vi "runStudy_USRP_2ChNCS_7.vi"() -> (2 "Ch2Amp":dbl[](graph), 3 "Ch1Amp":dbl[](graph), 4 "# elements in queue 2":i32)   [LabVIEW 2016]
uses:
  <instrlib>/niUSRP/niUSRP Timestamp.ctl
  <vilib>/Utility/miscctls.llb/LVDateTimeRec.ctl
  <vilib>/sound2/lvsound2.llb/Sound File Position.ctl
  <vilib>/sound2/lvsound2.llb/Sampling Mode.ctl
  <vilib>/sound2/lvsound2.llb/Sound Data Format.ctl
  <vilib>/Analysis/3filter.llb/Filter Passband Type.ctl
  <instrlib>/niUSRP/niUSRP Configure Time Start Trigger.vi
  <vilib>/sound2/lvsound2.llb/Sound Input Read (DBL).vi
  <instrlib>/niUSRP/niUSRP Write Tx Data (2D CDB).vi
  <instrlib>/niUSRP/niUSRP Fetch Rx Data (2D CDB).vi
  <vilib>/Analysis/3filter.llb/Butterworth Filter (DBL).vi
  <vilib>/Analysis/3filter.llb/Butterworth Filter (CDB).vi
  <vilib>/sound2/lvsound2.llb/Sound File Info (path).vi
  <vilib>/sound2/lvsound2.llb/Sound File Read Open.vi
  <vilib>/sound2/lvsound2.llb/Sound File Read (DBL).vi
  <vilib>/sound2/lvsound2.llb/Sound Output Write (DBL).vi
  <vilib>/measure/NI_MABase.lvlib
  <vilib>/Analysis/NI_AALBase.lvlib
  <vilib>/Analysis/NI_AALPro.lvlib
panel:
  in  "Sound R3a":T1=2 items=["Absolute"=0, "Relative"=2]
  in  "Play sound":u16(ring) items=["No sound", "Demo deep breathing", "Demo fast shallow breathing", "Demo slow shallow breathing", "Demo breath hold", "Demo cough/ laugh", "Demo abdomen movement", "Calibration", "Routine 1", "Routine 3b", "Routine 4/5/7", "Calm music", "Routine 3a"]
  in  "Sound Dcough":T1=2 items=["Absolute"=0, "Relative"=2]
  in  "Sound Dhold":T1=2 items=["Absolute"=0, "Relative"=2]
  in  "Sound Dabd":T1=2 items=["Absolute"=0, "Relative"=2]
  in  "Sound Dss":T1=2 items=["Absolute"=0, "Relative"=2]
  in  "Play/Stop":bool
  in  "Sound Ddeep":T1=2 items=["Absolute"=0, "Relative"=2]
  in  "Sound Dfs":T1=2 items=["Absolute"=0, "Relative"=2]
  in  "Sound R3b":T1=2 items=["Absolute"=0, "Relative"=2]
  in  "Sound R457":T1=2 items=["Absolute"=0, "Relative"=2]
  out "Next Task":string
  out "Calib 7":bool caption="Time has Elapsed"
  out "Calib 5":bool caption="Time has Elapsed"
  out "Calib 4":bool caption="Time has Elapsed"
  out "Calib 3":bool caption="Time has Elapsed"
  in  "Sound Calib":T1=2 items=["Absolute"=0, "Relative"=2]
  out "Calib 1":bool caption="Time has Elapsed"
  in  "Abd Circumference (cm)":string="0"
  in  "Thorax Circumference (cm)":string="0"
  out "Current Task time":dbl(slide) scale=0.0..60.0
  in  "Flush Th":i32=50
  in  "Stop 3":bool
  out "# elements in Mic":i32=5200
  in  "FlushMic":bool
  out "Mic":waveform(dbl)[](graph)
  in  "Device ID":u32 format="%.0x"
  in  "Number of Samples/ch":i32=5000
  in  "Sound Music":T1=2 items=["Absolute"=0, "Relative"=2]
  out "#2b":bool caption="Time has Elapsed"
  in  "Sound R1":T1=2 items=["Absolute"=0, "Relative"=2]
  in  "number of samples/ch":i32=5000
  out "#7":bool caption="Time has Elapsed"
  out "#2a":bool caption="Time has Elapsed"
  out "#6":bool caption="Time has Elapsed"
  out "#5":bool caption="Time has Elapsed"
  out "#4":bool caption="Time has Elapsed"
  in  "Comments":string
  in  "Tab Control 6":enum32{"Amp @500Hz", "Ph @500Hz"}(tab)
  out "IQ Graph 5":dbl[][](graph)
  out "IQ Graph 6":dbl[][](graph)
  in  "Tab Control 3":enum32{"Ch1 Amp", "Ch1 Ph"}(tab)
  in  "fh 1":dbl=26.0 format="%0.2f"
  in  "fl 1":dbl=0.7 format="%0.4f"
  out "Ch1Ph":dbl[](graph)
  in  "fl 3":dbl=0.7 format="%0.4f"
  in  "fh 3":dbl=26.0 format="%0.2f"
  in  "Tab Control 2":enum32{"Amp @50kHz", "Ph @50kHz"}(tab)
  out "Amp both":dbl[][](graph)
  out "Phase Both":dbl[][](graph)
  in  "Tab Control":enum32{"Ch2 Amp", "Ch2 Ph"}(tab)
  in  "fh 2":dbl=26.0 format="%0.2f"
  in  "fl 2":dbl=15.0 format="%0.4f"
  out "Ch2Ph":dbl[](graph)
  in  "fl 4":dbl=15.0 format="%0.4f"
  in  "fh 4":dbl=26.0 format="%0.2f"
  out "ArraySz":i32[](array[numeric])
  in  "Stop Test":bool
  out "#1":bool caption="Time has Elapsed"
  out "#3b":bool caption="Time has Elapsed"
  out "#3a":bool caption="Time has Elapsed"
  out "Elapsed Time (s)":dbl
  in  "Protocol":u16(ring) items=["Not Running", "Test Run", "Routine 1", "Routine 2a", "Routine 2b", "Routine 3a", "Routine 3b", "Routine 4", "Routine 5", "Routine 6", "Routine 7", "Calib1", "calib3", "Calib4", "Calib5", "Calib8"]
  out "Read:Tx IQ Rate":dbl=5000000.0
  out "Read:Rx IQ Rate":dbl=5000000.0
  out "date time rec":T2
  out "Total Routine Time":dbl(slide) scale=0.0..415.0
  out "Current Task":string
  in  "Weight (lbs)":string="0"
  in  "Case Number":string="0"
  in  "Height (cm)":string="0"
  in  "Sex":string(combo)="Female"
  in  "Age (years)":string="0"
  out "Numeric 2":i32=1
  out "Save":bool
  out "Flush":bool
  out "Buffer":bool
  out "Output":i32=1
  out "Configuration:Bandwidth":dbl=5000000.0
  out "Ch2 Amplitude":dbl=0.5 step=0.05 format="%#.6g"
  out "Ch1 Amplitude":dbl=0.5 step=0.05 format="%#.6g"
  out "Dis Sampling Rate":dbl=500.0 format="%#_6p"
  in  "DownSamplingRatio 2":i32=100
  out "Sampling Rate":dbl=50000.0 format="%#_6p"
  out "2Ch Waveforms":dbl[][](array[numeric])
  out "IterationNum":i32=1009
  in  "DownSamplingRatio":i32=40
  out "# elements in queue":i32
  out "BW/2":dbl=1000.0
  out "# of queue 1":i32
  in  "Dis1":bool=TRUE
  out "IQ Graph":dbl[][](graph)
  out "Tx1 Waveform":cdb[][](array[numeric])
  in  "Rx carrier frequency [Hz]":dbl=1900000000.0 format="%#_6p"
  in  "Tx carrier frequency [Hz]":dbl=1900000000.0 format="%#_6p"
  in  "Rx1 Gain 2":dbl=32.0 format="%#_6f"
  in  "Tx1 Gain 2":dbl=22.0 format="%#_6f"
  out "error out":errorcluster
  in  "Start Trigger Time":T3={"whole seconds"=1, "fractional seconds"=0.0}
  in  "Stop":bool
  in  "Channel 2\nTone Amplitude":dbl=0.5 step=0.05 format="%#.6g"
  in  "Channel 2 \nTone Frequency":dbl=131000.0 format="%#_6p"
  in  "Channel 1\nTone Amplitude":dbl=0.5 step=0.05 format="%#.6g"
  in  "Channel 1 \nTone Frequency":dbl=51000.0 format="%#_6p"
  out "Tx1 Waveform Graph":waveform(dbl)[](graph)
  in  "Waveform Size 1":dbl=20000.0
  in  "Device Name":refnum<k15>="MyB210"
  in  "Tx1 Gain 1":dbl=22.0 format="%#_6f"
  in  "Tx IQ Rate 1":dbl=2000000.0 format="%#_6p"
  in  "Rx1 Gain 1":dbl=32.0 format="%#_6f"
  in  "Rx IQ Rate 1":dbl=2000000.0 format="%#_6p"
  # "User Instructions"
  # "Step 1: User Information"
  # "Step 2: Protocol Selection"
  # "Ch 1"
  # "Ch 2"
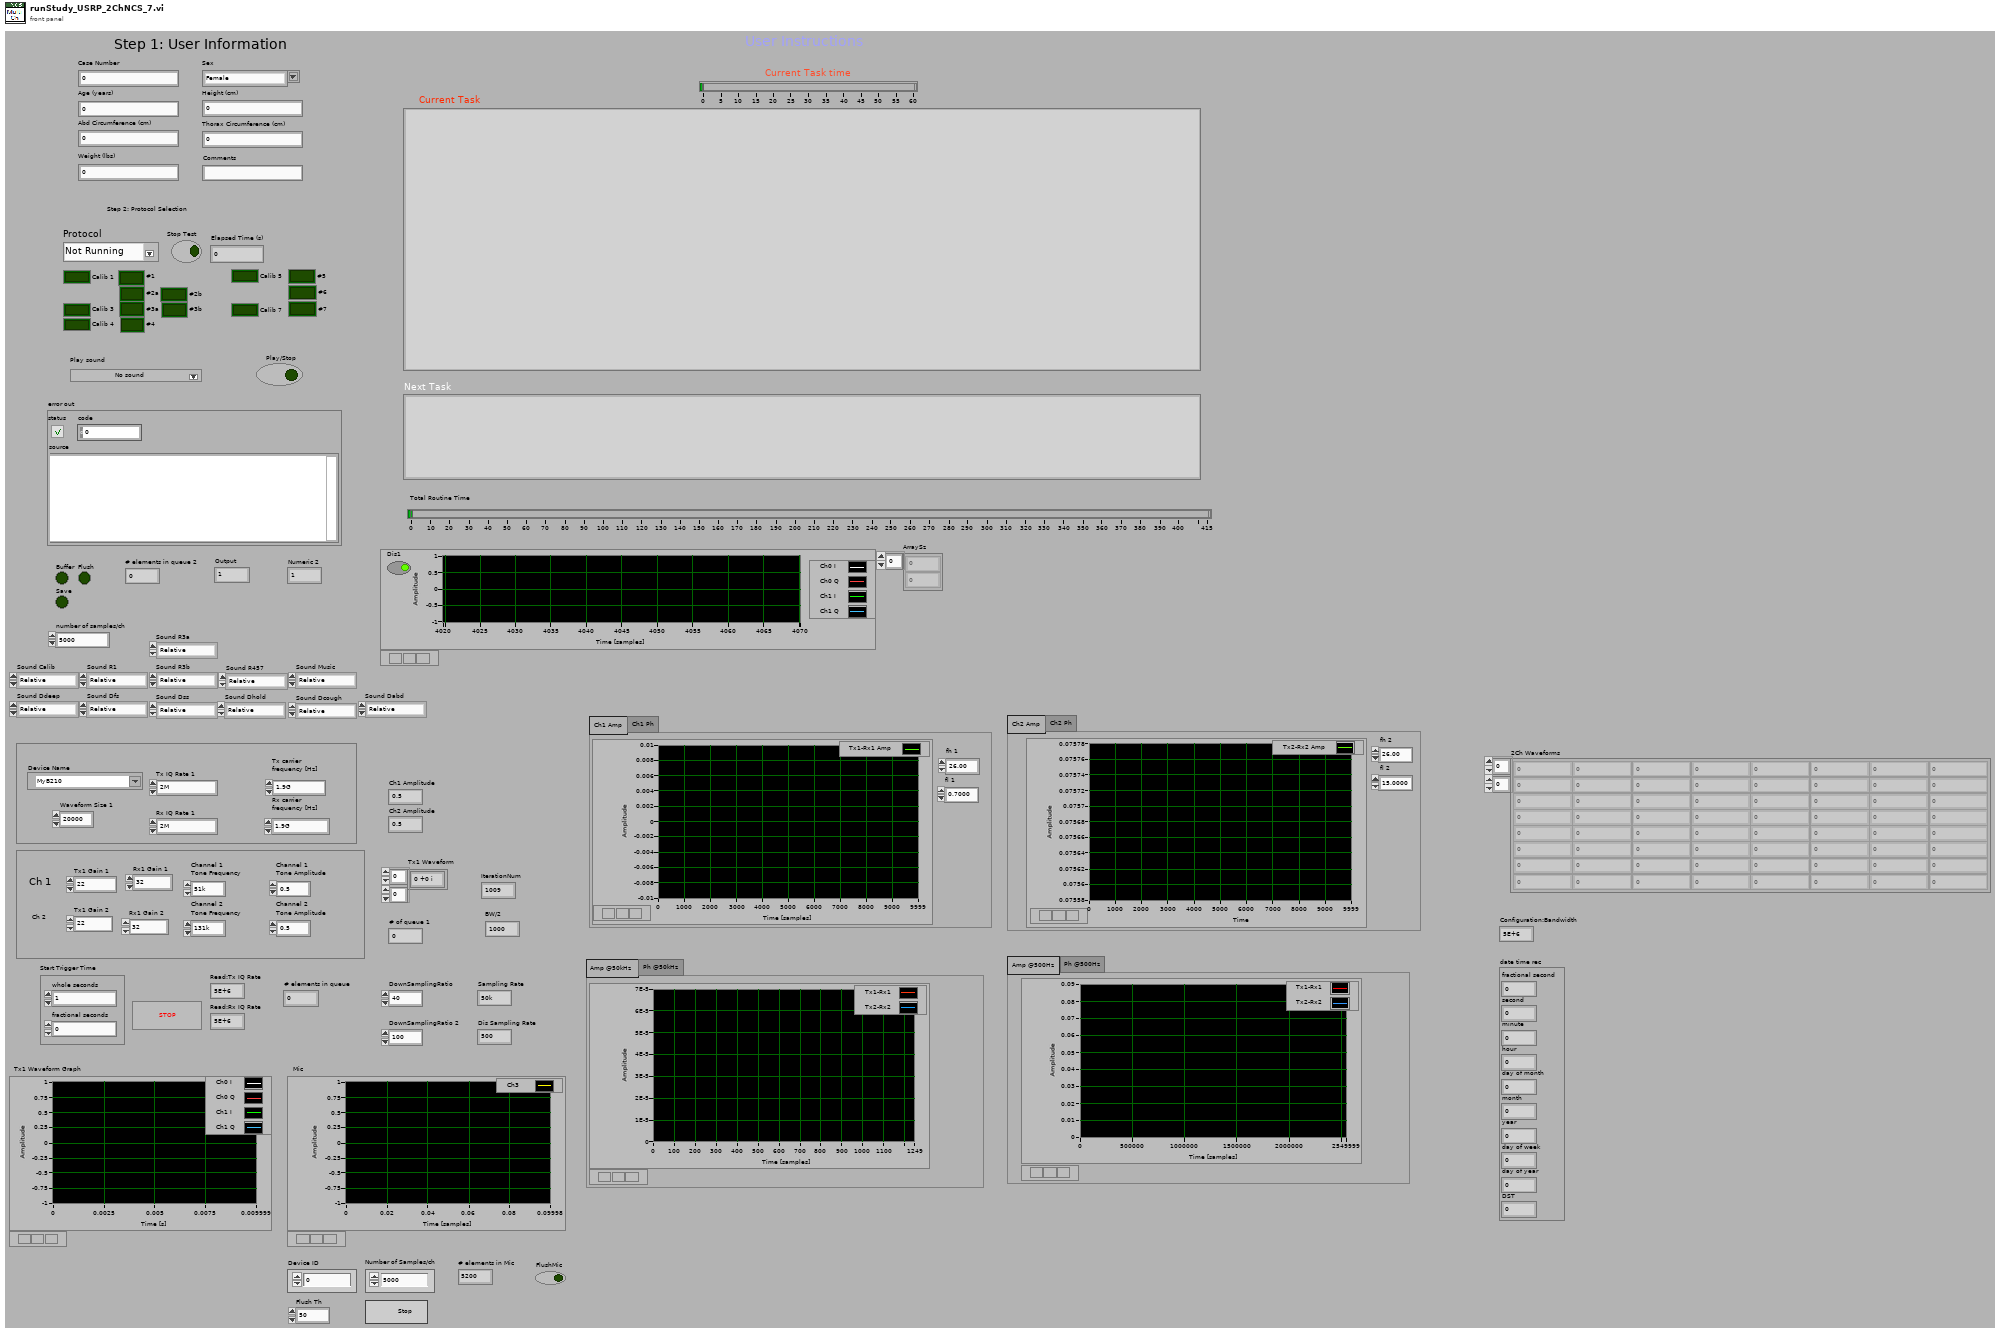
[diagram p1: front panel]
types:
  T1 = typedef "Sound File Position.ctl" = u16
  T2 = typedef "LVDateTimeRec.ctl" = cluster{"fractional second":dbl, "second":i32, "minute":i32, "hour":i32, "day of month":i32, "month":i32, "year":i32, "day of week":i32, "day of year":i32, "DST":i32}
  T3 = typedef "niUSRP Timestamp.ctl" = cluster{"whole seconds":u64, "fractional seconds":dbl}
  T4 = enum16{"Default", "Test", "Routine 1", "Routine 2a", "Routine 2b", "Routine 3a", "Routine 3b", "Routine 4", "Routine 5", "Routine 6", "Routine 7", "Calib1", "Calib3", "Calib4", "Calib5", "Calib7"}
  T5 = typedef "Sound Data Format.ctl" = cluster{"sample rate (S/s)":dbl, "number of channels":i32, "bits per sample":i32}
  T6 = typedef "Sampling Mode.ctl" = i32
  T7 = typedef "Sound File Refnum.ctl" = refnum<file>
  T8 = typedef "Sound Output Task ID.ctl" = u32
  T9 = typedef "NI_AALBase.lvlib/Filter Passband Type.ctl" = enum32{"Lowpass", "Highpass", "Bandpass", "Bandstop"}
  T10 = enum16{"Default", "Test", "Routine 1", "Routine 2", "Routine 3"}
  T11 = typedef "Sound Input Task ID.ctl" = u32
  T12 = enum16{"open", "open or create", "create or replace", "create", "open (read-only)"}
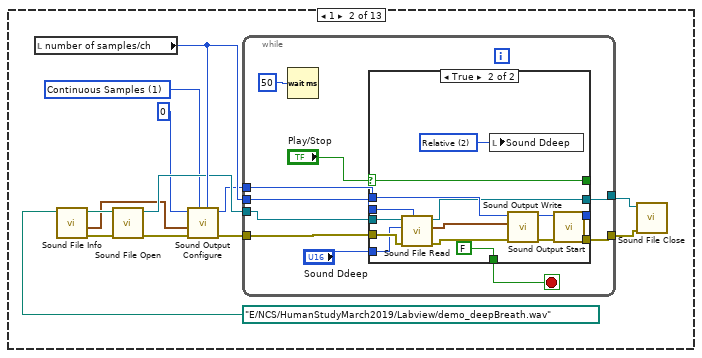
[diagram p3: hidden frame]
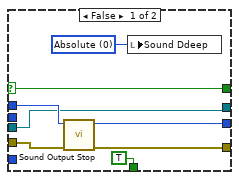
[diagram p4: hidden frame]
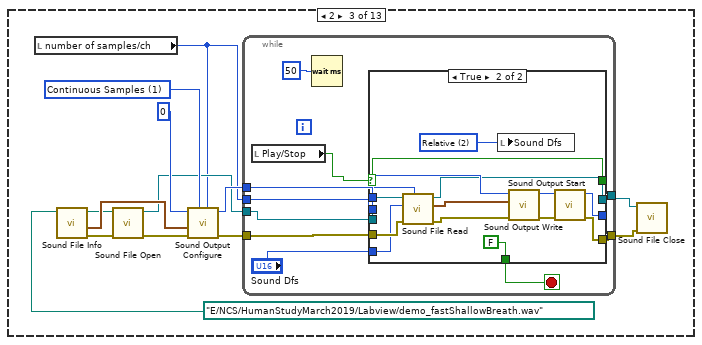
[diagram p5: hidden frame]
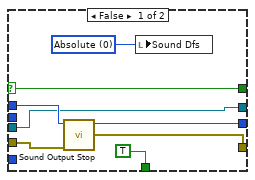
[diagram p6: hidden frame]
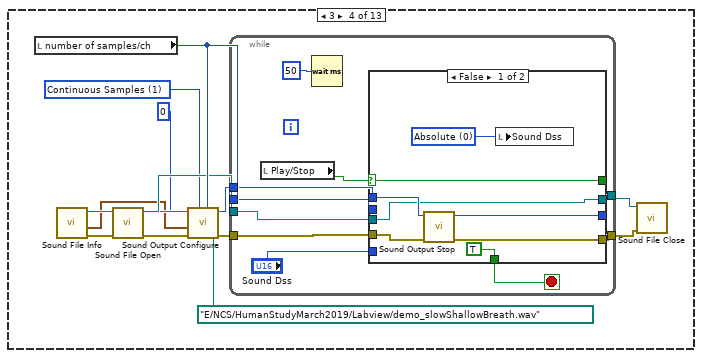
[diagram p7: hidden frame]
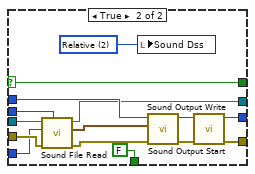
[diagram p8: hidden frame]
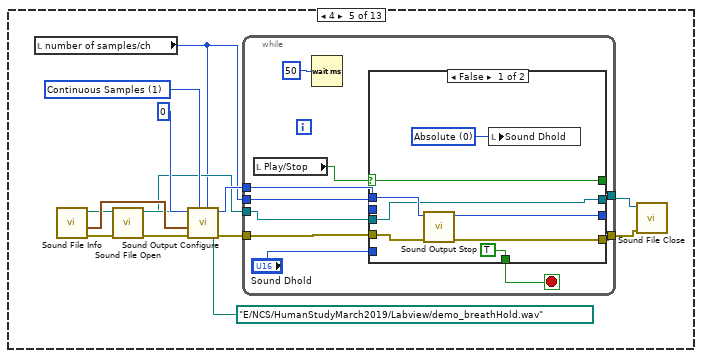
[diagram p9: hidden frame]
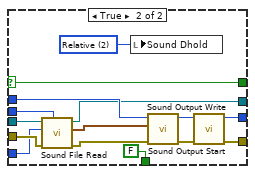
[diagram p10: hidden frame]
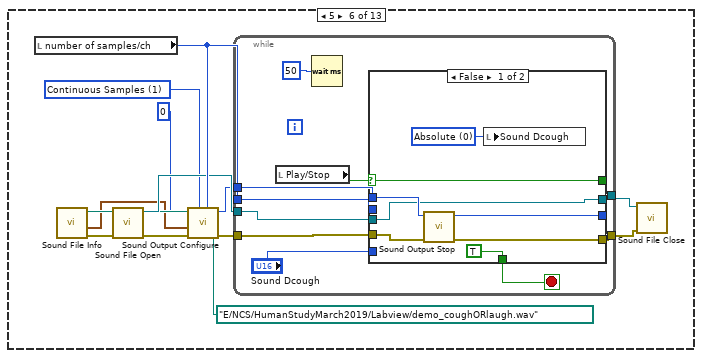
[diagram p11: hidden frame]
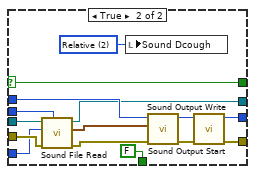
[diagram p12: hidden frame]
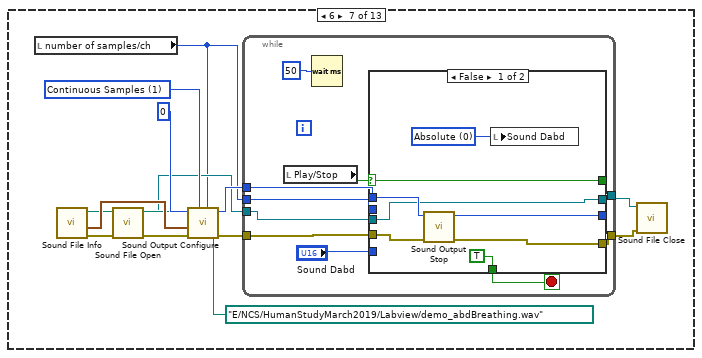
[diagram p13: hidden frame]
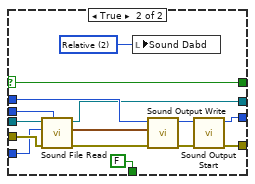
[diagram p14: hidden frame]
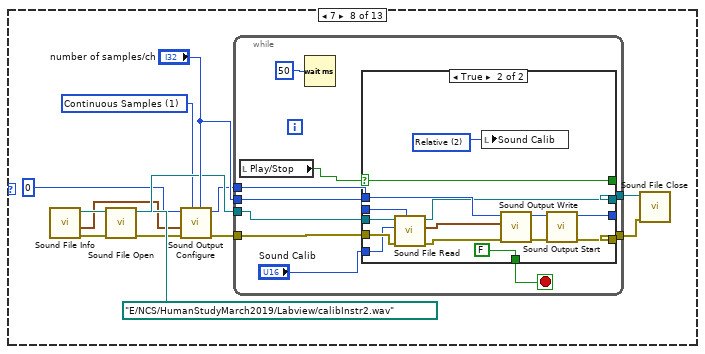
[diagram p15: hidden frame]
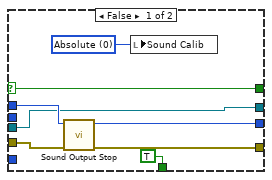
[diagram p16: hidden frame]
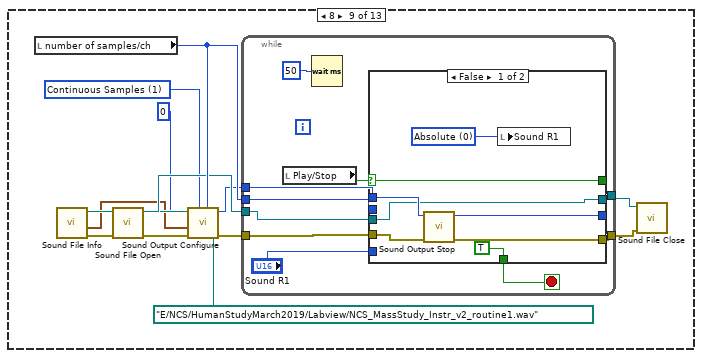
[diagram p17: hidden frame]
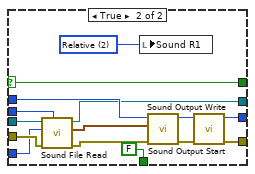
[diagram p18: hidden frame]
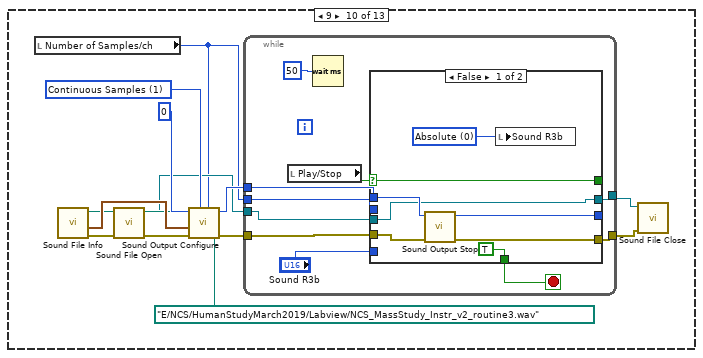
[diagram p19: hidden frame]
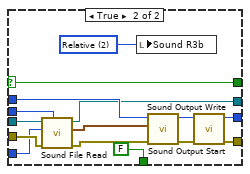
[diagram p20: hidden frame]
diagram:
  w8 = T6 1 items=["Finite Samples", "Continuous Samples"] ("sample mode")
  w16 = 0.0 ("element")
  w17 = 2000 ("dimension size")
  w28 = 4 ("dimension size")
  w65 = "RX2"  # Tx active antenna
  w121 = 1 items=["Now", "Next Timebase Edge"] ("apply timestamp")
  w93 = "TX1"  # Tx active antenna
  # "Microphone core"
  # "DownSamplingRatio"
  # "Set the attributes \nspecific to channel 1."
  # "Set the attributes \nspecific to channel 0."
  # "Set the attributes \nused by both Rx channels"
  # "Set the attributes \nspecific to Rx channel 1."
  # "Set the attributes \nspecific to Rx channel 0."
  n1 = local read "Device Name"() -> (w127:refnum<k15>)
  n2 = call <instrlib>:"niUSRP Open Rx Session.vi"("device names"="Device Name") -> ("session handle out"=w120:refnum<k15>, "error out"=w119:errorcluster)  [unwired: 13 in]
  n3 = property class="niUSRP"(reference=w120, error in=w119, "Enabled Channels"="0,1" ("Configuration:Enabled Channels")) -> (reference out=w118:refnum<k15>, error out=w117:errorcluster)
  n4 = call-poly <instrlib>:"niUSRP Configure Trigger.vi"("session handle"=w118, "start trigger time"="Start Trigger Time", "error in (no error)"=w117) -> ("session handle out"=w114:refnum<k15>, "error out"=w113:errorcluster)  [unwired: 11 in]
  n5 = property class="niUSRP"(reference=w114, error in=w113, "IQ Rate"="Rx IQ Rate 1") -> (reference out=w110:refnum<k15>, error out=w111:errorcluster)
  n6 = property class="niUSRP" props=["Model", "Reference Frequency Source", "Timebase Clock Source"](reference=w110, error in=w111, "Reference Frequency Source"="Internal" ("Clocking and Synchronization:Reference Frequency Source"), "Timebase Clock Source"="Internal" ("Clocking and Synchronization:Timebase Clock Source")) -> (reference out=w106:refnum<k15>, error out=w107:errorcluster)  [unwired: 1 out]
  n7 = property class="niUSRP"(reference=w106, error in=w107, "Carrier Frequency"="Rx carrier frequency [Hz]", "Bandwidth"=5000000.0 ("Configuration:Bandwidth")) -> (reference out=w77:refnum<k15>, error out=w76:errorcluster, "IQ Rate"=→"Read:Rx IQ Rate":dbl)
  n8 = property class="niUSRP"(reference=w77, error in=w76, "Active Channel"="0", "Gain"="Rx1 Gain 1", "Active Antenna"=w65) -> (reference out=w81:refnum<k15>, error out=w80:errorcluster, "Bandwidth"=→"Configuration:Bandwidth":dbl)
  n9 = property class="niUSRP"(reference=w81, error in=w80, "Active Channel"="1", "Gain"="Rx1 Gain 2", "Active Antenna"=w65) -> (reference out=w109:refnum<k15>, error out=w108:errorcluster)
  n10 = call <instrlib>:"niUSRP Open Tx Session.vi"("device names"=w127, "error in (no error)"=w108) -> ("session handle out"=w116:refnum<k15>, "error out"=w115:errorcluster)  [unwired: 12 in]
  n11 = property class="niUSRP"(reference=w116, error in=w115, "Enabled Channels"="0,1" ("Configuration:Enabled Channels")) -> (reference out=w104:refnum<k15>, error out=w103:errorcluster)
  n12 = property class="niUSRP"(reference=w104, error in=w103, "IQ Rate"="Tx IQ Rate 1") -> (reference out=w98:refnum<k15>, error out=w99:errorcluster, "IQ Rate"=w97:dbl)
  n13 = property class="niUSRP" props=["Model", "Reference Frequency Source", "Timebase Clock Source"](reference=w98, error in=w99, "Reference Frequency Source"="Internal" ("Clocking and Synchronization:Reference Frequency Source"), "Timebase Clock Source"="Internal" ("Clocking and Synchronization:Timebase Clock Source")) -> (reference out=w100:refnum<k15>, error out=w101:errorcluster)  [unwired: 1 out]
  n14 = property class="niUSRP"(reference=w100, error in=w101, "Carrier Frequency"="Tx carrier frequency [Hz]") -> (reference out=w70:refnum<k15>, error out=w69:errorcluster, "IQ Rate"=→"Read:Tx IQ Rate":dbl)
  n15 = property class="niUSRP"(reference=w70, error in=w69, "Active Channel"="0", "Gain"="Tx1 Gain 1", "Active Antenna"=w93) -> (reference out=w74:refnum<k15>, error out=w73:errorcluster)
  n16 = property class="niUSRP"(reference=w74, error in=w73, "Active Channel"="1", "Gain"="Tx1 Gain 2", "Active Antenna"=w93) -> (reference out=w95:refnum<k15>, error out=w96:errorcluster)
  n17 = while {
    stop <- FALSE stop-if-true
    n18 = local read "Output"() -> (w134:i32)
    n19 = Wait (ms)(milliseconds to wait=u32 50) -> ()  [unwired: 1 out]
    n20 = case shown="0, Default" w134 {
      tunnel: [w139 "Channel 1\nTone Amplitude"] -> w136
      tunnel: [w139 "Channel 2\nTone Amplitude"] -> w135
      frame 0, Default {
        w139 = 0.0 ("Channel 1\nTone Amplitude")
      }
      frame 1 {
      }
    }
    "Ch1 Amplitude" <- w136
    "Ch2 Amplitude" <- w135
  }
  n21 = call <instrlib>:"niUSRP Commit.vi"("session handle"=w95, "error in (no error)"=w96) -> ("session handle out"=w129:refnum<k15>, "error out"=w130:errorcluster)  [unwired: 12 in]
  n22 = Merge Errors(w108, w130) -> (w24:errorcluster)
  n23 = call <instrlib>:"niUSRP Set Time.vi"("session handle"=w109, "apply timestamp"=w121, "timestamp"=T3 {"whole seconds"=0, "fractional seconds"=0.0}, "error in (no error)"=w24) -> ("session handle out"=w123:refnum<k15>, "error out"=w122:errorcluster)  [unwired: 10 in]
  n24 = call <instrlib>:"niUSRP Initiate.vi"("session handle"=w123, "error in (no error)"=w122) -> ("session handle out"=w133:refnum<k15>, "error out"=w64:errorcluster)  [unwired: 12 in]
  n25 = while {
    tunnel: w97 -> [w152]
    tunnel: w64 -> [w144]
    stop <- FALSE stop-if-true
    # "Generate I and Q waveforms."
    n26 = Wait (ms)(milliseconds to wait=u32 100) -> ()  [unwired: 1 out]
    n27 = Bundle By Name(cluster=cluster{"Fs":dbl, "#s":dbl} {"Fs"=1000.0, "#s"=1000.0} ("sampling info"), "Fs"=w152, "#s"="Waveform Size 1") -> (w153:cluster{"Fs":dbl, "#s":dbl})
    n28 = local read "Ch1 Amplitude"() -> (w143:dbl)
    n29 = local read "Ch2 Amplitude"() -> (w142:dbl)
    n30 = call <vilib>:"Sine Waveform.vi"("sampling info"=w153, "error in (no error)"=w144, "phase"=90.0, "amplitude"=w143, "frequency"="Channel 1 \nTone Frequency") -> ("error out"=w148:errorcluster, "signal out"=w166:waveform(dbl))  [unwired: 5 in]
    n31 = call <vilib>:"Sine Waveform.vi"("sampling info"=w153, "error in (no error)"=w144, "amplitude"=w143, "frequency"="Channel 1 \nTone Frequency") -> ("error out"=w149:errorcluster, "signal out"=w167:waveform(dbl))  [unwired: 6 in]
    n32 = call <vilib>:"Sine Waveform.vi"("sampling info"=w153, "error in (no error)"=w144, "phase"=90.0, "amplitude"=w142, "frequency"="Channel 2 \nTone Frequency") -> ("error out"=w150:errorcluster, "signal out"=w157:waveform(dbl))  [unwired: 5 in]
    n33 = call <vilib>:"Sine Waveform.vi"("sampling info"=w153, "error in (no error)"=w144, "amplitude"=w142, "frequency"="Channel 2 \nTone Frequency") -> ("error out"=w151:errorcluster, "signal out"=w156:waveform(dbl))  [unwired: 6 in]
    n34 = Merge Errors(w148, w149, w150, w151) -> ()  [unwired: 1 out]
    n35 = Build Array(w166, w167, w157, w156) -> (→"Tx1 Waveform Graph":waveform(dbl)[])
    n36 = Unbundle By Name(w166) -> ("Y"=w165:dbl[])
    n37 = Unbundle By Name(w167) -> ("Y"=w164:dbl[])
    n38 = Unbundle By Name(w157) -> ("Y"=w160:dbl[])
    n39 = Unbundle By Name(w156) -> ("Y"=w159:dbl[])
    n40 = Re/Im To Complex(1:w164, 2:w165) -> (0:w155:cdb[])
    n41 = Re/Im To Complex(1:w159, 2:w160) -> (0:w154:cdb[])
    n42 = Build Array(w155, w154) -> (→"Tx1 Waveform":cdb[][])
  }
  n43 = local read "Waveform Size 1"() -> (w58:dbl)
  n44 = Initialize Array(cdb 0.0+0.0i ("element"), 2 ("dimension size"), w58) -> (w55:cdb[][])
  n45 = Obtain Queue(max queue size (-1, unlimited)=-1, name (unnamed)="Rx1Queue", element data type=w55) -> (queue out=w53:refnum<queue>)  [unwired: 2 in, 2 out]
  n46 = while {
    tunnel: w53 -> [w172]
    stop <- FALSE stop-if-true
    n47 = Wait (ms)(milliseconds to wait=u32 2) -> ()  [unwired: 1 out]
    n48 = case shown="True" "Dis1" {
      tunnel: w172 -> [_ w176]
      frame False {
        n49 = Wait (ms)(milliseconds to wait=u32 500) -> ()  [unwired: 1 out]
      }
      frame True {
        n50 = Preview Queue Element(queue=w176) -> (element=w178:cdb[][])  [unwired: 2 in, 3 out]
        n51 = for {
          tunnel: w178 -> [w184] mode=indexing
          shift-right: [w181] -> w177
          shift-left: dbl[][] [] -> [w180]
          n52 = Complex To Re/Im(x + iy=w184) -> (x=w183:dbl[], y=w182:dbl[])
          n53 = Build Array (concatenate)(w180, w183, w182) -> (w181:dbl[][])
        }
        "IQ Graph" <- w177
      }
    }
  }
  n54 = while {
    tunnel: w133 -> [w199]
    tunnel: w64 -> [w198]
    tunnel: [w194] -> w90
    tunnel: [w197] -> w87
    shift-right: [w190] -> _
    shift-left: w53 -> [w191]
    i -> [w187]
    stop <- w193 stop-if-true
    # "Rx on both channels"
    n55 = local read "Waveform Size 1"() -> (w192:dbl)
    n56 = call-poly <instrlib>:"niUSRP Fetch Rx Data (poly).vi"("session handle"=w199, "number of samples"=w192, "error in (no error)"=w198) -> ("session handle out"=w197:refnum<k15>, "data"=w189:cdb[][], "timestamp"=w188:T3, "error out"=w194:errorcluster)  [unwired: 9 in]
    n57 = call <instrlib>:"niUSRP USRP Timestamp to LV Timestamp.vi"("USRP Timestamp"=w188) -> ()  [unwired: 13 in, 2 out]
    n58 = Less Or Equal?(x=w187, y=1) -> (x <= y?=w185:bool)
    n59 = case shown="True" w185 {
      frame False {
        n60 = local write "FlushMic"(FALSE ("FlushMic")) -> ()
      }
      frame True {
        n61 = local write "FlushMic"(TRUE ("FlushMic")) -> ()
      }
    }
    n62 = Enqueue Element(queue=w191, element=w189) -> (queue out=w190:refnum<queue>)  [unwired: 2 in, 2 out]
    n63 = Unbundle By Name(w194) -> ("status"=w196:bool)
    n64 = Or(x=w196, y="Stop") -> (x .or. y?=w193:bool)
  }
  n65 = while {
    tunnel: w129 -> [w209]
    tunnel: w64 -> [w208]
    tunnel: [w206] -> w92
    tunnel: [w204] -> w85
    stop <- w205 stop-if-true
    # "Tx on both channels"
    n66 = local read "Tx1 Waveform"() -> (w202:cdb[][])
    n67 = local read "Stop"() -> (w203:bool)
    n68 = call-poly <instrlib>:"niUSRP Write Tx Data (poly).vi"("session handle"=w209, "data"=w202, "end of data?"=w203, "error in (no error)"=w208) -> ("session handle out"=w204:refnum<k15>, "error out"=w206:errorcluster)  [unwired: 10 in]
    n69 = Unbundle By Name(w206) -> ("status"=w207:bool)
    n70 = Compound Arithmetic op=OR(w207, w203) -> (w205:bool)
  }
  n71 = flat-sequence {
    tunnel: [w211] -> w91
    tunnel: w92 -> [w211]
    tunnel: [w210] -> w86
    tunnel: w85 -> [w210]
    frame #0 {
      n72 = local write "Stop"(TRUE ("STOP")) -> ()
    }
  }
  n73 = while {
    stop <- FALSE stop-if-true
    n74 = Wait (ms)(milliseconds to wait=u32 50) -> ()  [unwired: 1 out]
    n75 = case shown="12" "Play sound" {
      frame 0, Default {
      }
      frame 1 {
        w216 = T6 1 items=["Finite Samples", "Continuous Samples"] ("sample mode")
        n76 = local read "number of samples/ch"() -> (w228:i32)
        n77 = call-poly <vilib>:"Sound File Info.vi"("path"=path "E:/NCS/HumanStudyMarch2019/Labview/demo_deepBreath.wav") -> ("error out"=w220:errorcluster, "sound format"=w219:T5, "path out"=w221:path)  [unwired: 7 in, 1 out]
        n78 = call-poly <vilib>:"Sound File Open.vi"("error in (no error)"=w220, "path"=w221) -> ("error out"=w217:errorcluster, "sound file refnum"=w225:T7)  [unwired: 8 in]
        n79 = call <vilib>:"Sound Output Configure.vi"("number of samples/ch"=w228, "sample mode"=w216, "error in (no error)"=w217, "sound format"=w219, "device ID"=u32 0) -> ("error out"=w226:errorcluster, "task ID"=w224:T8)  [unwired: 5 in]
        n80 = while {
          tunnel: w224 -> [w238]
          tunnel: [w237] -> w223
          tunnel: w225 -> [w232]
          tunnel: w226 -> [w231]
          tunnel: w228 -> [w233]
          tunnel: [w236] -> w227
          stop <- w229 stop-if-true
          n81 = Wait (ms)(milliseconds to wait=u32 50) -> ()  [unwired: 1 out]
          n82 = case shown="True" "Play/Stop" {
            selector: "Play/Stop" -> [w243 w261]
            tunnel: w238 -> [w246 w258]
            tunnel: [w244 w260] -> w237
            tunnel: [w245 w259] -> _
            tunnel: [w243 w261] -> _
            tunnel: [w241 w255] -> w236
            tunnel: w233 -> [_ w252]
            tunnel: w232 -> [w241 w251]
            tunnel: w231 -> [w242 w250]
            tunnel: "Sound Ddeep" -> [_ w249]
            tunnel: [TRUE FALSE] -> w229
            frame False {
              w240 = T1 0 items=["Absolute"=0, "Relative"=2] ("position mode")
              n83 = call <vilib>:"Sound Output Stop.vi"("error in (no error)"=w242, "task ID"=w246) -> ("error out"=w244:errorcluster, "task ID out"=w245:T8)  [unwired: 8 in]
              n84 = local write "Sound Ddeep"(w240) -> ()
            }
            frame True {
              w248 = T1 2 items=["Absolute"=0, "Relative"=2] ("position mode")
              n85 = call-poly <vilib>:"Sound File Read.vi"("number of samples/ch (-1: all)"=w252, "error in (no error)"=w250, "position mode"=w249, "sound file refnum"=w251) -> ("error out"=w254:errorcluster, "data"=w253:waveform(dbl)[], "sound file refnum out"=w255:T7)  [unwired: 3 in, 2 out]
              n86 = local write "Sound Ddeep"(w248) -> ()
              n87 = call-poly <vilib>:"Sound Output Write.vi"("error in (no error)"=w254, "data"=w253, "task ID"=w258) -> ("error out"=w256:errorcluster, "task ID out"=w257:T8)  [unwired: 7 in]
              n88 = call <vilib>:"Sound Output Start.vi"("error in (no error)"=w256, "task ID"=w257) -> ("error out"=w260:errorcluster, "task ID out"=w259:T8)  [unwired: 8 in]
            }
          }
        }
        n89 = call <vilib>:"Sound File Close.vi"("error in (no error)"=w223, "sound file refnum"=w227) -> ()  [unwired: 9 in, 1 out]
      }
      frame 2 {
        w274 = T6 1 items=["Finite Samples", "Continuous Samples"] ("sample mode")
        n90 = local read "number of samples/ch"() -> (w263:i32)
        n91 = call-poly <vilib>:"Sound File Info.vi"("path"=path "E:/NCS/HumanStudyMarch2019/Labview/demo_fastShallowBreath.wav") -> ("error out"=w270:errorcluster, "sound format"=w271:T5, "path out"=w269:path)  [unwired: 7 in, 1 out]
        n92 = call-poly <vilib>:"Sound File Open.vi"("error in (no error)"=w270, "path"=w269) -> ("error out"=w273:errorcluster, "sound file refnum"=w266:T7)  [unwired: 8 in]
        n93 = call <vilib>:"Sound Output Configure.vi"("number of samples/ch"=w263, "sample mode"=w274, "error in (no error)"=w273, "sound format"=w271, "device ID"=u32 0) -> ("error out"=w265:errorcluster, "task ID"=w267:T8)  [unwired: 5 in]
        n94 = while {
          tunnel: w267 -> [w284]
          tunnel: [w283] -> w268
          tunnel: w266 -> [w279]
          tunnel: w265 -> [w278]
          tunnel: w263 -> [w280]
          tunnel: [w282] -> w264
          stop <- w276 stop-if-true
          n95 = local read "Play/Stop"() -> (w275:bool)
          n96 = Wait (ms)(milliseconds to wait=u32 50) -> ()  [unwired: 1 out]
          n97 = case shown="True" w275 {
            selector: w275 -> [w289 w307]
            tunnel: w284 -> [w292 w304]
            tunnel: [w290 w306] -> w283
            tunnel: [w291 w305] -> _
            tunnel: [w289 w307] -> _
            tunnel: [w287 w301] -> w282
            tunnel: w280 -> [_ w298]
            tunnel: w279 -> [w287 w297]
            tunnel: w278 -> [w288 w296]
            tunnel: "Sound Dfs" -> [_ w295]
            tunnel: [TRUE FALSE] -> w276
            frame False {
              w286 = T1 0 items=["Absolute"=0, "Relative"=2] ("position mode")
              n98 = call <vilib>:"Sound Output Stop.vi"("error in (no error)"=w288, "task ID"=w292) -> ("error out"=w290:errorcluster, "task ID out"=w291:T8)  [unwired: 8 in]
              n99 = local write "Sound Dfs"(w286) -> ()
            }
            frame True {
              w294 = T1 2 items=["Absolute"=0, "Relative"=2] ("position mode")
              n100 = call-poly <vilib>:"Sound File Read.vi"("number of samples/ch (-1: all)"=w298, "error in (no error)"=w296, "position mode"=w295, "sound file refnum"=w297) -> ("error out"=w300:errorcluster, "data"=w299:waveform(dbl)[], "sound file refnum out"=w301:T7)  [unwired: 3 in, 2 out]
              n101 = local write "Sound Dfs"(w294) -> ()
              n102 = call-poly <vilib>:"Sound Output Write.vi"("error in (no error)"=w300, "data"=w299, "task ID"=w304) -> ("error out"=w302:errorcluster, "task ID out"=w303:T8)  [unwired: 7 in]
              n103 = call <vilib>:"Sound Output Start.vi"("error in (no error)"=w302, "task ID"=w303) -> ("error out"=w306:errorcluster, "task ID out"=w305:T8)  [unwired: 8 in]
            }
          }
        }
        n104 = call <vilib>:"Sound File Close.vi"("error in (no error)"=w268, "sound file refnum"=w264) -> ()  [unwired: 9 in, 1 out]
      }
      frame 3 {
        w308 = T6 1 items=["Finite Samples", "Continuous Samples"] ("sample mode")
        n105 = local read "number of samples/ch"() -> (w320:i32)
        n106 = call-poly <vilib>:"Sound File Info.vi"("path"=path "E:/NCS/HumanStudyMarch2019/Labview/demo_slowShallowBreath.wav") -> ("error out"=w312:errorcluster, "sound format"=w311:T5, "path out"=w313:path)  [unwired: 7 in, 1 out]
        n107 = call-poly <vilib>:"Sound File Open.vi"("error in (no error)"=w312, "path"=w313) -> ("error out"=w309:errorcluster, "sound file refnum"=w317:T7)  [unwired: 8 in]
        n108 = call <vilib>:"Sound Output Configure.vi"("number of samples/ch"=w320, "sample mode"=w308, "error in (no error)"=w309, "sound format"=w311, "device ID"=u32 0) -> ("error out"=w318:errorcluster, "task ID"=w316:T8)  [unwired: 5 in]
        n109 = while {
          tunnel: w316 -> [w330]
          tunnel: [w329] -> w315
          tunnel: w317 -> [w325]
          tunnel: w318 -> [w324]
          tunnel: w320 -> [w326]
          tunnel: [w328] -> w319
          stop <- w322 stop-if-true
          n110 = local read "Play/Stop"() -> (w321:bool)
          n111 = Wait (ms)(milliseconds to wait=u32 50) -> ()  [unwired: 1 out]
          n112 = case shown="False" w321 {
            selector: w321 -> [w335 w353]
            tunnel: w330 -> [w338 w350]
            tunnel: [w336 w352] -> w329
            tunnel: [w337 w351] -> _
            tunnel: [w335 w353] -> _
            tunnel: [w333 w347] -> w328
            tunnel: w326 -> [_ w344]
            tunnel: w325 -> [w333 w343]
            tunnel: w324 -> [w334 w342]
            tunnel: "Sound Dss" -> [_ w341]
            tunnel: [TRUE FALSE] -> w322
            frame False {
              w332 = T1 0 items=["Absolute"=0, "Relative"=2] ("position mode")
              n113 = call <vilib>:"Sound Output Stop.vi"("error in (no error)"=w334, "task ID"=w338) -> ("error out"=w336:errorcluster, "task ID out"=w337:T8)  [unwired: 8 in]
              n114 = local write "Sound Dss"(w332) -> ()
            }
            frame True {
              w340 = T1 2 items=["Absolute"=0, "Relative"=2] ("position mode")
              n115 = call-poly <vilib>:"Sound File Read.vi"("number of samples/ch (-1: all)"=w344, "error in (no error)"=w342, "position mode"=w341, "sound file refnum"=w343) -> ("error out"=w346:errorcluster, "data"=w345:waveform(dbl)[], "sound file refnum out"=w347:T7)  [unwired: 3 in, 2 out]
              n116 = local write "Sound Dss"(w340) -> ()
              n117 = call-poly <vilib>:"Sound Output Write.vi"("error in (no error)"=w346, "data"=w345, "task ID"=w350) -> ("error out"=w348:errorcluster, "task ID out"=w349:T8)  [unwired: 7 in]
              n118 = call <vilib>:"Sound Output Start.vi"("error in (no error)"=w348, "task ID"=w349) -> ("error out"=w352:errorcluster, "task ID out"=w351:T8)  [unwired: 8 in]
            }
          }
        }
        n119 = call <vilib>:"Sound File Close.vi"("error in (no error)"=w315, "sound file refnum"=w319) -> ()  [unwired: 9 in, 1 out]
      }
      frame 4 {
        w366 = T6 1 items=["Finite Samples", "Continuous Samples"] ("sample mode")
        n120 = local read "number of samples/ch"() -> (w354:i32)
        n121 = call-poly <vilib>:"Sound File Info.vi"("path"=path "E:/NCS/HumanStudyMarch2019/Labview/demo_breathHold.wav") -> ("error out"=w362:errorcluster, "sound format"=w363:T5, "path out"=w361:path)  [unwired: 7 in, 1 out]
        n122 = call-poly <vilib>:"Sound File Open.vi"("error in (no error)"=w362, "path"=w361) -> ("error out"=w365:errorcluster, "sound file refnum"=w357:T7)  [unwired: 8 in]
        n123 = call <vilib>:"Sound Output Configure.vi"("number of samples/ch"=w354, "sample mode"=w366, "error in (no error)"=w365, "sound format"=w363, "device ID"=u32 0) -> ("error out"=w356:errorcluster, "task ID"=w358:T8)  [unwired: 5 in]
        n124 = while {
          tunnel: w358 -> [w376]
          tunnel: [w375] -> w359
          tunnel: w357 -> [w371]
          tunnel: w356 -> [w370]
          tunnel: w354 -> [w372]
          tunnel: [w374] -> w355
          stop <- w368 stop-if-true
          n125 = local read "Play/Stop"() -> (w367:bool)
          n126 = Wait (ms)(milliseconds to wait=u32 50) -> ()  [unwired: 1 out]
          n127 = case shown="False" w367 {
            selector: w367 -> [w381 w399]
            tunnel: w376 -> [w384 w396]
            tunnel: [w382 w398] -> w375
            tunnel: [w383 w397] -> _
            tunnel: [w381 w399] -> _
            tunnel: [w379 w393] -> w374
            tunnel: w372 -> [_ w390]
            tunnel: w371 -> [w379 w389]
            tunnel: w370 -> [w380 w388]
            tunnel: "Sound Dhold" -> [_ w387]
            tunnel: [TRUE FALSE] -> w368
            frame False {
              w378 = T1 0 items=["Absolute"=0, "Relative"=2] ("position mode")
              n128 = call <vilib>:"Sound Output Stop.vi"("error in (no error)"=w380, "task ID"=w384) -> ("error out"=w382:errorcluster, "task ID out"=w383:T8)  [unwired: 8 in]
              n129 = local write "Sound Dhold"(w378) -> ()
            }
            frame True {
              w386 = T1 2 items=["Absolute"=0, "Relative"=2] ("position mode")
              n130 = call-poly <vilib>:"Sound File Read.vi"("number of samples/ch (-1: all)"=w390, "error in (no error)"=w388, "position mode"=w387, "sound file refnum"=w389) -> ("error out"=w392:errorcluster, "data"=w391:waveform(dbl)[], "sound file refnum out"=w393:T7)  [unwired: 3 in, 2 out]
              n131 = local write "Sound Dhold"(w386) -> ()
              n132 = call-poly <vilib>:"Sound Output Write.vi"("error in (no error)"=w392, "data"=w391, "task ID"=w396) -> ("error out"=w394:errorcluster, "task ID out"=w395:T8)  [unwired: 7 in]
              n133 = call <vilib>:"Sound Output Start.vi"("error in (no error)"=w394, "task ID"=w395) -> ("error out"=w398:errorcluster, "task ID out"=w397:T8)  [unwired: 8 in]
            }
          }
        }
        n134 = call <vilib>:"Sound File Close.vi"("error in (no error)"=w359, "sound file refnum"=w355) -> ()  [unwired: 9 in, 1 out]
      }
      frame 5 {
        w400 = T6 1 items=["Finite Samples", "Continuous Samples"] ("sample mode")
        n135 = local read "number of samples/ch"() -> (w412:i32)
        n136 = call-poly <vilib>:"Sound File Info.vi"("path"=path "E:/NCS/HumanStudyMarch2019/Labview/demo_coughORlaugh.wav") -> ("error out"=w404:errorcluster, "sound format"=w403:T5, "path out"=w405:path)  [unwired: 7 in, 1 out]
        n137 = call-poly <vilib>:"Sound File Open.vi"("error in (no error)"=w404, "path"=w405) -> ("error out"=w401:errorcluster, "sound file refnum"=w409:T7)  [unwired: 8 in]
        n138 = call <vilib>:"Sound Output Configure.vi"("number of samples/ch"=w412, "sample mode"=w400, "error in (no error)"=w401, "sound format"=w403, "device ID"=u32 0) -> ("error out"=w410:errorcluster, "task ID"=w408:T8)  [unwired: 5 in]
        n139 = while {
          tunnel: w408 -> [w422]
          tunnel: [w421] -> w407
          tunnel: w409 -> [w417]
          tunnel: w410 -> [w416]
          tunnel: w412 -> [w418]
          tunnel: [w420] -> w411
          stop <- w414 stop-if-true
          n140 = local read "Play/Stop"() -> (w413:bool)
          n141 = Wait (ms)(milliseconds to wait=u32 50) -> ()  [unwired: 1 out]
          n142 = case shown="False" w413 {
            selector: w413 -> [w427 w445]
            tunnel: w422 -> [w430 w442]
            tunnel: [w428 w444] -> w421
            tunnel: [w429 w443] -> _
            tunnel: [w427 w445] -> _
            tunnel: [w425 w439] -> w420
            tunnel: w418 -> [_ w436]
            tunnel: w417 -> [w425 w435]
            tunnel: w416 -> [w426 w434]
            tunnel: "Sound Dcough" -> [_ w433]
            tunnel: [TRUE FALSE] -> w414
            frame False {
              w424 = T1 0 items=["Absolute"=0, "Relative"=2] ("position mode")
              n143 = call <vilib>:"Sound Output Stop.vi"("error in (no error)"=w426, "task ID"=w430) -> ("error out"=w428:errorcluster, "task ID out"=w429:T8)  [unwired: 8 in]
              n144 = local write "Sound Dcough"(w424) -> ()
            }
            frame True {
              w432 = T1 2 items=["Absolute"=0, "Relative"=2] ("position mode")
              n145 = call-poly <vilib>:"Sound File Read.vi"("number of samples/ch (-1: all)"=w436, "error in (no error)"=w434, "position mode"=w433, "sound file refnum"=w435) -> ("error out"=w438:errorcluster, "data"=w437:waveform(dbl)[], "sound file refnum out"=w439:T7)  [unwired: 3 in, 2 out]
              n146 = local write "Sound Dcough"(w432) -> ()
              n147 = call-poly <vilib>:"Sound Output Write.vi"("error in (no error)"=w438, "data"=w437, "task ID"=w442) -> ("error out"=w440:errorcluster, "task ID out"=w441:T8)  [unwired: 7 in]
              n148 = call <vilib>:"Sound Output Start.vi"("error in (no error)"=w440, "task ID"=w441) -> ("error out"=w444:errorcluster, "task ID out"=w443:T8)  [unwired: 8 in]
            }
          }
        }
        n149 = call <vilib>:"Sound File Close.vi"("error in (no error)"=w407, "sound file refnum"=w411) -> ()  [unwired: 9 in, 1 out]
      }
      frame 6 {
        w458 = T6 1 items=["Finite Samples", "Continuous Samples"] ("sample mode")
        n150 = local read "number of samples/ch"() -> (w446:i32)
        n151 = call-poly <vilib>:"Sound File Info.vi"("path"=path "E:/NCS/HumanStudyMarch2019/Labview/demo_abdBreathing.wav") -> ("error out"=w454:errorcluster, "sound format"=w455:T5, "path out"=w453:path)  [unwired: 7 in, 1 out]
        n152 = call-poly <vilib>:"Sound File Open.vi"("error in (no error)"=w454, "path"=w453) -> ("error out"=w457:errorcluster, "sound file refnum"=w449:T7)  [unwired: 8 in]
        n153 = call <vilib>:"Sound Output Configure.vi"("number of samples/ch"=w446, "sample mode"=w458, "error in (no error)"=w457, "sound format"=w455, "device ID"=u32 0) -> ("error out"=w448:errorcluster, "task ID"=w450:T8)  [unwired: 5 in]
        n154 = while {
          tunnel: w450 -> [w468]
          tunnel: [w467] -> w451
          tunnel: w449 -> [w463]
          tunnel: w448 -> [w462]
          tunnel: w446 -> [w464]
          tunnel: [w466] -> w447
          stop <- w459 stop-if-true
          n155 = local read "Play/Stop"() -> (w460:bool)
          n156 = Wait (ms)(milliseconds to wait=u32 50) -> ()  [unwired: 1 out]
          n157 = case shown="False" w460 {
            selector: w460 -> [w473 w491]
            tunnel: w468 -> [w476 w488]
            tunnel: [w474 w490] -> w467
            tunnel: [w475 w489] -> _
            tunnel: [w473 w491] -> _
            tunnel: [w471 w485] -> w466
            tunnel: w464 -> [_ w482]
            tunnel: w463 -> [w471 w481]
            tunnel: w462 -> [w472 w480]
            tunnel: "Sound Dabd" -> [_ w479]
            tunnel: [TRUE FALSE] -> w459
            frame False {
              w470 = T1 0 items=["Absolute"=0, "Relative"=2] ("position mode")
              n158 = call <vilib>:"Sound Output Stop.vi"("error in (no error)"=w472, "task ID"=w476) -> ("error out"=w474:errorcluster, "task ID out"=w475:T8)  [unwired: 8 in]
              n159 = local write "Sound Dabd"(w470) -> ()
            }
            frame True {
              w478 = T1 2 items=["Absolute"=0, "Relative"=2] ("position mode")
              n160 = call-poly <vilib>:"Sound File Read.vi"("number of samples/ch (-1: all)"=w482, "error in (no error)"=w480, "position mode"=w479, "sound file refnum"=w481) -> ("error out"=w484:errorcluster, "data"=w483:waveform(dbl)[], "sound file refnum out"=w485:T7)  [unwired: 3 in, 2 out]
              n161 = local write "Sound Dabd"(w478) -> ()
              n162 = call-poly <vilib>:"Sound Output Write.vi"("error in (no error)"=w484, "data"=w483, "task ID"=w488) -> ("error out"=w486:errorcluster, "task ID out"=w487:T8)  [unwired: 7 in]
              n163 = call <vilib>:"Sound Output Start.vi"("error in (no error)"=w486, "task ID"=w487) -> ("error out"=w490:errorcluster, "task ID out"=w489:T8)  [unwired: 8 in]
            }
          }
        }
        n164 = call <vilib>:"Sound File Close.vi"("error in (no error)"=w451, "sound file refnum"=w447) -> ()  [unwired: 9 in, 1 out]
      }
      frame 7 {
        w492 = T6 1 items=["Finite Samples", "Continuous Samples"] ("sample mode")
        n165 = call-poly <vilib>:"Sound File Info.vi"("path"=path "E:/NCS/HumanStudyMarch2019/Labview/calibInstr2.wav") -> ("error out"=w496:errorcluster, "sound format"=w495:T5, "path out"=w497:path)  [unwired: 7 in, 1 out]
        n166 = call-poly <vilib>:"Sound File Open.vi"("error in (no error)"=w496, "path"=w497) -> ("error out"=w493:errorcluster, "sound file refnum"=w501:T7)  [unwired: 8 in]
        n167 = call <vilib>:"Sound Output Configure.vi"("number of samples/ch"="number of samples/ch", "sample mode"=w492, "error in (no error)"=w493, "sound format"=w495, "device ID"=u32 0) -> ("error out"=w502:errorcluster, "task ID"=w500:T8)  [unwired: 5 in]
        n168 = while {
          tunnel: w500 -> [w514]
          tunnel: [w513] -> w499
          tunnel: w501 -> [w509]
          tunnel: w502 -> [w508]
          tunnel: "number of samples/ch" -> [w510]
          tunnel: [w512] -> w503
          stop <- w505 stop-if-true
          n169 = local read "Play/Stop"() -> (w506:bool)
          n170 = Wait (ms)(milliseconds to wait=u32 50) -> ()  [unwired: 1 out]
          n171 = case shown="True" w506 {
            selector: w506 -> [w519 w537]
            tunnel: w514 -> [w522 w534]
            tunnel: [w520 w536] -> w513
            tunnel: [w521 w535] -> _
            tunnel: [w519 w537] -> _
            tunnel: [w517 w531] -> w512
            tunnel: w510 -> [_ w528]
            tunnel: w509 -> [w517 w527]
            tunnel: w508 -> [w518 w526]
            tunnel: "Sound Calib" -> [_ w525]
            tunnel: [TRUE FALSE] -> w505
            frame False {
              w516 = T1 0 items=["Absolute"=0, "Relative"=2] ("position mode")
              n172 = call <vilib>:"Sound Output Stop.vi"("error in (no error)"=w518, "task ID"=w522) -> ("error out"=w520:errorcluster, "task ID out"=w521:T8)  [unwired: 8 in]
              n173 = local write "Sound Calib"(w516) -> ()
            }
            frame True {
              w524 = T1 2 items=["Absolute"=0, "Relative"=2] ("position mode")
              n174 = call-poly <vilib>:"Sound File Read.vi"("number of samples/ch (-1: all)"=w528, "error in (no error)"=w526, "position mode"=w525, "sound file refnum"=w527) -> ("error out"=w530:errorcluster, "data"=w529:waveform(dbl)[], "sound file refnum out"=w531:T7)  [unwired: 3 in, 2 out]
              n175 = local write "Sound Calib"(w524) -> ()
              n176 = call-poly <vilib>:"Sound Output Write.vi"("error in (no error)"=w530, "data"=w529, "task ID"=w534) -> ("error out"=w532:errorcluster, "task ID out"=w533:T8)  [unwired: 7 in]
              n177 = call <vilib>:"Sound Output Start.vi"("error in (no error)"=w532, "task ID"=w533) -> ("error out"=w536:errorcluster, "task ID out"=w535:T8)  [unwired: 8 in]
            }
          }
        }
        n178 = call <vilib>:"Sound File Close.vi"("error in (no error)"=w499, "sound file refnum"=w503) -> ()  [unwired: 9 in, 1 out]
      }
      frame 8 {
        w538 = T6 1 items=["Finite Samples", "Continuous Samples"] ("sample mode")
        n179 = local read "number of samples/ch"() -> (w550:i32)
        n180 = call-poly <vilib>:"Sound File Info.vi"("path"=path "E:/NCS/HumanStudyMarch2019/Labview/NCS_MassStudy_Instr_v2_routine1.wav") -> ("error out"=w542:errorcluster, "sound format"=w541:T5, "path out"=w543:path)  [unwired: 7 in, 1 out]
        n181 = call-poly <vilib>:"Sound File Open.vi"("error in (no error)"=w542, "path"=w543) -> ("error out"=w539:errorcluster, "sound file refnum"=w547:T7)  [unwired: 8 in]
        n182 = call <vilib>:"Sound Output Configure.vi"("number of samples/ch"=w550, "sample mode"=w538, "error in (no error)"=w539, "sound format"=w541, "device ID"=u32 0) -> ("error out"=w548:errorcluster, "task ID"=w546:T8)  [unwired: 5 in]
        n183 = while {
          tunnel: w546 -> [w560]
          tunnel: [w559] -> w545
          tunnel: w547 -> [w555]
          tunnel: w548 -> [w554]
          tunnel: w550 -> [w556]
          tunnel: [w558] -> w549
          stop <- w551 stop-if-true
          n184 = local read "Play/Stop"() -> (w552:bool)
          n185 = Wait (ms)(milliseconds to wait=u32 50) -> ()  [unwired: 1 out]
          n186 = case shown="False" w552 {
            selector: w552 -> [w565 w583]
            tunnel: w560 -> [w568 w580]
            tunnel: [w566 w582] -> w559
            tunnel: [w567 w581] -> _
            tunnel: [w565 w583] -> _
            tunnel: [w563 w577] -> w558
            tunnel: w556 -> [_ w574]
            tunnel: w555 -> [w563 w573]
            tunnel: w554 -> [w564 w572]
            tunnel: "Sound R1" -> [_ w571]
            tunnel: [TRUE FALSE] -> w551
            frame False {
              w562 = T1 0 items=["Absolute"=0, "Relative"=2] ("position mode")
              n187 = call <vilib>:"Sound Output Stop.vi"("error in (no error)"=w564, "task ID"=w568) -> ("error out"=w566:errorcluster, "task ID out"=w567:T8)  [unwired: 8 in]
              n188 = local write "Sound R1"(w562) -> ()
            }
            frame True {
              w570 = T1 2 items=["Absolute"=0, "Relative"=2] ("position mode")
              n189 = call-poly <vilib>:"Sound File Read.vi"("number of samples/ch (-1: all)"=w574, "error in (no error)"=w572, "position mode"=w571, "sound file refnum"=w573) -> ("error out"=w576:errorcluster, "data"=w575:waveform(dbl)[], "sound file refnum out"=w577:T7)  [unwired: 3 in, 2 out]
              n190 = local write "Sound R1"(w570) -> ()
              n191 = call-poly <vilib>:"Sound Output Write.vi"("error in (no error)"=w576, "data"=w575, "task ID"=w580) -> ("error out"=w578:errorcluster, "task ID out"=w579:T8)  [unwired: 7 in]
              n192 = call <vilib>:"Sound Output Start.vi"("error in (no error)"=w578, "task ID"=w579) -> ("error out"=w582:errorcluster, "task ID out"=w581:T8)  [unwired: 8 in]
            }
          }
        }
        n193 = call <vilib>:"Sound File Close.vi"("error in (no error)"=w545, "sound file refnum"=w549) -> ()  [unwired: 9 in, 1 out]
      }
      frame 9 {
        w596 = T6 1 items=["Finite Samples", "Continuous Samples"] ("sample mode")
        n194 = local read "Number of Samples/ch"() -> (w584:i32)
        n195 = call-poly <vilib>:"Sound File Info.vi"("path"=path "E:/NCS/HumanStudyMarch2019/Labview/NCS_MassStudy_Instr_v2_routine3.wav") -> ("error out"=w592:errorcluster, "sound format"=w593:T5, "path out"=w591:path)  [unwired: 7 in, 1 out]
        n196 = call-poly <vilib>:"Sound File Open.vi"("error in (no error)"=w592, "path"=w591) -> ("error out"=w595:errorcluster, "sound file refnum"=w587:T7)  [unwired: 8 in]
        n197 = call <vilib>:"Sound Output Configure.vi"("number of samples/ch"=w584, "sample mode"=w596, "error in (no error)"=w595, "sound format"=w593, "device ID"=u32 0) -> ("error out"=w586:errorcluster, "task ID"=w588:T8)  [unwired: 5 in]
        n198 = while {
          tunnel: w588 -> [w606]
          tunnel: [w605] -> w589
          tunnel: w587 -> [w601]
          tunnel: w586 -> [w600]
          tunnel: w584 -> [w602]
          tunnel: [w604] -> w585
          stop <- w597 stop-if-true
          n199 = local read "Play/Stop"() -> (w598:bool)
          n200 = Wait (ms)(milliseconds to wait=u32 50) -> ()  [unwired: 1 out]
          n201 = case shown="False" w598 {
            selector: w598 -> [w611 w629]
            tunnel: w606 -> [w614 w626]
            tunnel: [w612 w628] -> w605
            tunnel: [w613 w627] -> _
            tunnel: [w611 w629] -> _
            tunnel: [w609 w623] -> w604
            tunnel: w602 -> [_ w620]
            tunnel: w601 -> [w609 w619]
            tunnel: w600 -> [w610 w618]
            tunnel: "Sound R3b" -> [_ w617]
            tunnel: [TRUE FALSE] -> w597
            frame False {
              w608 = T1 0 items=["Absolute"=0, "Relative"=2] ("position mode")
              n202 = call <vilib>:"Sound Output Stop.vi"("error in (no error)"=w610, "task ID"=w614) -> ("error out"=w612:errorcluster, "task ID out"=w613:T8)  [unwired: 8 in]
              n203 = local write "Sound R3b"(w608) -> ()
            }
            frame True {
              w616 = T1 2 items=["Absolute"=0, "Relative"=2] ("position mode")
              n204 = call-poly <vilib>:"Sound File Read.vi"("number of samples/ch (-1: all)"=w620, "error in (no error)"=w618, "position mode"=w617, "sound file refnum"=w619) -> ("error out"=w622:errorcluster, "data"=w621:waveform(dbl)[], "sound file refnum out"=w623:T7)  [unwired: 3 in, 2 out]
              n205 = local write "Sound R3b"(w616) -> ()
              n206 = call-poly <vilib>:"Sound Output Write.vi"("error in (no error)"=w622, "data"=w621, "task ID"=w626) -> ("error out"=w624:errorcluster, "task ID out"=w625:T8)  [unwired: 7 in]
              n207 = call <vilib>:"Sound Output Start.vi"("error in (no error)"=w624, "task ID"=w625) -> ("error out"=w628:errorcluster, "task ID out"=w627:T8)  [unwired: 8 in]
            }
          }
        }
        n208 = call <vilib>:"Sound File Close.vi"("error in (no error)"=w589, "sound file refnum"=w585) -> ()  [unwired: 9 in, 1 out]
      }
      frame 10 {
        w630 = T6 1 items=["Finite Samples", "Continuous Samples"] ("sample mode")
        n209 = local read "Number of Samples/ch"() -> (w642:i32)
        n210 = call-poly <vilib>:"Sound File Info.vi"("path"=path "E:/NCS/HumanStudyMarch2019/Labview/NCS_MassStudy_Instr_v2_routine457.wav") -> ("error out"=w634:errorcluster, "sound format"=w633:T5, "path out"=w635:path)  [unwired: 7 in, 1 out]
        n211 = call-poly <vilib>:"Sound File Open.vi"("error in (no error)"=w634, "path"=w635) -> ("error out"=w631:errorcluster, "sound file refnum"=w639:T7)  [unwired: 8 in]
        n212 = call <vilib>:"Sound Output Configure.vi"("number of samples/ch"=w642, "sample mode"=w630, "error in (no error)"=w631, "sound format"=w633, "device ID"=u32 0) -> ("error out"=w640:errorcluster, "task ID"=w638:T8)  [unwired: 5 in]
        n213 = while {
          tunnel: w638 -> [w652]
          tunnel: [w651] -> w637
          tunnel: w639 -> [w647]
          tunnel: w640 -> [w646]
          tunnel: w642 -> [w648]
          tunnel: [w650] -> w641
          stop <- w643 stop-if-true
          n214 = local read "Play/Stop"() -> (w644:bool)
          n215 = Wait (ms)(milliseconds to wait=u32 50) -> ()  [unwired: 1 out]
          n216 = case shown="False" w644 {
            selector: w644 -> [w657 w675]
            tunnel: w652 -> [w660 w672]
            tunnel: [w658 w674] -> w651
            tunnel: [w659 w673] -> _
            tunnel: [w657 w675] -> _
            tunnel: [w655 w669] -> w650
            tunnel: w648 -> [_ w666]
            tunnel: w647 -> [w655 w665]
            tunnel: w646 -> [w656 w664]
            tunnel: "Sound R457" -> [_ w663]
            tunnel: [TRUE FALSE] -> w643
            frame False {
              w654 = T1 0 items=["Absolute"=0, "Relative"=2] ("position mode")
              n217 = call <vilib>:"Sound Output Stop.vi"("error in (no error)"=w656, "task ID"=w660) -> ("error out"=w658:errorcluster, "task ID out"=w659:T8)  [unwired: 8 in]
              n218 = local write "Sound R457"(w654) -> ()
            }
            frame True {
              w662 = T1 2 items=["Absolute"=0, "Relative"=2] ("position mode")
              n219 = call-poly <vilib>:"Sound File Read.vi"("number of samples/ch (-1: all)"=w666, "error in (no error)"=w664, "position mode"=w663, "sound file refnum"=w665) -> ("error out"=w668:errorcluster, "data"=w667:waveform(dbl)[], "sound file refnum out"=w669:T7)  [unwired: 3 in, 2 out]
              n220 = local write "Sound R457"(w662) -> ()
              n221 = call-poly <vilib>:"Sound Output Write.vi"("error in (no error)"=w668, "data"=w667, "task ID"=w672) -> ("error out"=w670:errorcluster, "task ID out"=w671:T8)  [unwired: 7 in]
              n222 = call <vilib>:"Sound Output Start.vi"("error in (no error)"=w670, "task ID"=w671) -> ("error out"=w674:errorcluster, "task ID out"=w673:T8)  [unwired: 8 in]
            }
          }
        }
        n223 = call <vilib>:"Sound File Close.vi"("error in (no error)"=w637, "sound file refnum"=w641) -> ()  [unwired: 9 in, 1 out]
      }
      frame 11 {
        w676 = T6 1 items=["Finite Samples", "Continuous Samples"] ("sample mode")
        n224 = local read "number of samples/ch"() -> (w688:i32)
        n225 = call-poly <vilib>:"Sound File Info.vi"("path"=path "E:/NCS/HumanStudyMarch2019/Labview/calmMusic2.wav") -> ("error out"=w680:errorcluster, "sound format"=w679:T5, "path out"=w681:path)  [unwired: 7 in, 1 out]
        n226 = call-poly <vilib>:"Sound File Open.vi"("error in (no error)"=w680, "path"=w681) -> ("error out"=w677:errorcluster, "sound file refnum"=w685:T7)  [unwired: 8 in]
        n227 = call <vilib>:"Sound Output Configure.vi"("number of samples/ch"=w688, "sample mode"=w676, "error in (no error)"=w677, "sound format"=w679, "device ID"=u32 0) -> ("error out"=w686:errorcluster, "task ID"=w684:T8)  [unwired: 5 in]
        n228 = while {
          tunnel: w684 -> [w698]
          tunnel: [w697] -> w683
          tunnel: w685 -> [w693]
          tunnel: w686 -> [w692]
          tunnel: w688 -> [w694]
          tunnel: [w696] -> w687
          stop <- w689 stop-if-true
          n229 = local read "Play/Stop"() -> (w690:bool)
          n230 = Wait (ms)(milliseconds to wait=u32 50) -> ()  [unwired: 1 out]
          n231 = case shown="False" w690 {
            selector: w690 -> [w703 w721]
            tunnel: w698 -> [w706 w718]
            tunnel: [w704 w720] -> w697
            tunnel: [w705 w719] -> _
            tunnel: [w703 w721] -> _
            tunnel: [w701 w715] -> w696
            tunnel: w694 -> [_ w712]
            tunnel: w693 -> [w701 w711]
            tunnel: w692 -> [w702 w710]
            tunnel: "Sound Music" -> [_ w709]
            tunnel: [TRUE FALSE] -> w689
            frame False {
              w700 = T1 0 items=["Absolute"=0, "Relative"=2] ("position mode")
              n232 = call <vilib>:"Sound Output Stop.vi"("error in (no error)"=w702, "task ID"=w706) -> ("error out"=w704:errorcluster, "task ID out"=w705:T8)  [unwired: 8 in]
              n233 = local write "Sound Music"(w700) -> ()
            }
            frame True {
              w708 = T1 2 items=["Absolute"=0, "Relative"=2] ("position mode")
              n234 = call-poly <vilib>:"Sound File Read.vi"("number of samples/ch (-1: all)"=w712, "error in (no error)"=w710, "position mode"=w709, "sound file refnum"=w711) -> ("error out"=w714:errorcluster, "data"=w713:waveform(dbl)[], "sound file refnum out"=w715:T7)  [unwired: 3 in, 2 out]
              n235 = local write "Sound Music"(w708) -> ()
              n236 = call-poly <vilib>:"Sound Output Write.vi"("error in (no error)"=w714, "data"=w713, "task ID"=w718) -> ("error out"=w716:errorcluster, "task ID out"=w717:T8)  [unwired: 7 in]
              n237 = call <vilib>:"Sound Output Start.vi"("error in (no error)"=w716, "task ID"=w717) -> ("error out"=w720:errorcluster, "task ID out"=w719:T8)  [unwired: 8 in]
            }
          }
        }
        n238 = call <vilib>:"Sound File Close.vi"("error in (no error)"=w683, "sound file refnum"=w687) -> ()  [unwired: 9 in, 1 out]
      }
      frame 12 {
        w722 = T6 1 items=["Finite Samples", "Continuous Samples"] ("sample mode")
        n239 = local read "number of samples/ch"() -> (w734:i32)
        n240 = call-poly <vilib>:"Sound File Info.vi"("path"=path "E:/NCS/HumanStudyMarch2019/Labview/NCS_massStudy_bikeTiming.wav") -> ("error out"=w726:errorcluster, "sound format"=w725:T5, "path out"=w727:path)  [unwired: 7 in, 1 out]
        n241 = call-poly <vilib>:"Sound File Open.vi"("error in (no error)"=w726, "path"=w727) -> ("error out"=w723:errorcluster, "sound file refnum"=w731:T7)  [unwired: 8 in]
        n242 = call <vilib>:"Sound Output Configure.vi"("number of samples/ch"=w734, "sample mode"=w722, "error in (no error)"=w723, "sound format"=w725, "device ID"=u32 0) -> ("error out"=w732:errorcluster, "task ID"=w730:T8)  [unwired: 5 in]
        n243 = while {
          tunnel: w730 -> [w744]
          tunnel: [w743] -> w729
          tunnel: w731 -> [w739]
          tunnel: w732 -> [w738]
          tunnel: w734 -> [w740]
          tunnel: [w742] -> w733
          stop <- w735 stop-if-true
          n244 = local read "Play/Stop"() -> (w736:bool)
          n245 = Wait (ms)(milliseconds to wait=u32 50) -> ()  [unwired: 1 out]
          n246 = case shown="False" w736 {
            selector: w736 -> [w749 w767]
            tunnel: w744 -> [w752 w764]
            tunnel: [w750 w766] -> w743
            tunnel: [w751 w765] -> _
            tunnel: [w749 w767] -> _
            tunnel: [w747 w761] -> w742
            tunnel: w740 -> [_ w758]
            tunnel: w739 -> [w747 w757]
            tunnel: w738 -> [w748 w756]
            tunnel: "Sound R3a" -> [_ w755]
            tunnel: [TRUE FALSE] -> w735
            frame False {
              w746 = T1 0 items=["Absolute"=0, "Relative"=2] ("position mode")
              n247 = call <vilib>:"Sound Output Stop.vi"("error in (no error)"=w748, "task ID"=w752) -> ("error out"=w750:errorcluster, "task ID out"=w751:T8)  [unwired: 8 in]
              n248 = local write "Sound R3a"(w746) -> ()
            }
            frame True {
              w754 = T1 2 items=["Absolute"=0, "Relative"=2] ("position mode")
              n249 = call-poly <vilib>:"Sound File Read.vi"("number of samples/ch (-1: all)"=w758, "error in (no error)"=w756, "position mode"=w755, "sound file refnum"=w757) -> ("error out"=w760:errorcluster, "data"=w759:waveform(dbl)[], "sound file refnum out"=w761:T7)  [unwired: 3 in, 2 out]
              n250 = local write "Sound R3a"(w754) -> ()
              n251 = call-poly <vilib>:"Sound Output Write.vi"("error in (no error)"=w760, "data"=w759, "task ID"=w764) -> ("error out"=w762:errorcluster, "task ID out"=w763:T8)  [unwired: 7 in]
              n252 = call <vilib>:"Sound Output Start.vi"("error in (no error)"=w762, "task ID"=w763) -> ("error out"=w766:errorcluster, "task ID out"=w765:T8)  [unwired: 8 in]
            }
          }
        }
        n253 = call <vilib>:"Sound File Close.vi"("error in (no error)"=w729, "sound file refnum"=w733) -> ()  [unwired: 9 in, 1 out]
      }
    }
  }
  n254 = local read "Rx IQ Rate 1"() -> (w33:dbl)
  n255 = flat-sequence {
    tunnel: [w769] -> w89
    tunnel: w90 -> [w769]
    tunnel: [w768] -> w88
    tunnel: w87 -> [w768]
    frame #0 {
      n256 = local write "Stop"(TRUE ("STOP")) -> ()
    }
  }
  n257 = local read "Waveform Size 1"() -> (w46:dbl)
  n258 = Divide(x=w33, y="DownSamplingRatio") -> (x/y=→"Sampling Rate":dbl)
  n259 = call <instrlib>:"niUSRP Abort.vi"("session handle"=w88, "error in (no error)"=w89) -> ("session handle out"=w126:refnum<k15>, "error out"=w125:errorcluster)  [unwired: 12 in]
  n260 = Divide(x=2000.0, y=2.0) -> (x/y=→"BW/2":dbl)
  n261 = call <instrlib>:"niUSRP Close Session.vi"("session handle"=w126, "error in (no error)"=w125) -> ("error out"=w84:errorcluster)  [unwired: 13 in]
  n262 = call <instrlib>:"niUSRP Close Session.vi"("session handle"=w86, "error in (no error)"=w91) -> ("error out"=w83:errorcluster)  [unwired: 13 in]
  n263 = Divide(x=w46, y="DownSamplingRatio") -> (x/y=w27:dbl)
  n264 = flat-sequence {
    tunnel: w84 -> [w773]
    tunnel: w83 -> [w772]
    tunnel: [w771] -> w82
    frame #0 {
      n265 = Merge Errors(w773, w772) -> (w771:errorcluster)
      n266 = local write "Stop"(FALSE ("STOP")) -> ()
    }
  }
  n267 = Obtain Queue(name (unnamed)="Microphone", element data type=0.0 ("element")) -> (queue out=w2:refnum<queue>)  [unwired: 3 in, 2 out]
  n268 = Initialize Array(0.0 ("element"), w28, w27) -> (w47:dbl[][])
  n269 = Initialize Array(0.0 ("element"), w28, w27) -> (w35:dbl[][])
  n270 = local read "Channel 1 \nTone Frequency"() -> (w20:dbl)
  n271 = local read "Channel 2 \nTone Frequency"() -> (w19:dbl)
  n272 = Obtain Queue(name (unnamed)="Buffer", element data type=w35) -> (queue out=w34:refnum<queue>)  [unwired: 3 in, 2 out]
  n273 = Obtain Queue(name (unnamed)="ChsQueue", element data type=w47) -> (queue out=w45:refnum<queue>)  [unwired: 3 in, 2 out]
  n274 = local read "Waveform Size 1"() -> (w21:dbl)
  n275 = local read "Rx IQ Rate 1"() -> (w18:dbl)
  n276 = while {
    tunnel: w53 -> [w849]
    tunnel: w45 -> [w826]
    tunnel: w34 -> [w825]
    tunnel: w21 -> [w815]
    tunnel: w20 -> [w781]
    tunnel: w19 -> [w782]
    tunnel: w18 -> [w814]
    tunnel: w2 -> [w776]
    stop <- FALSE stop-if-true
    w783 = 1
    # "Note the order, it is not the same as above."
    # "Rx 2 - Tx 2"
    # "Rx 1 - Tx 1"
    # "Tx2 to Rx2 QueInd_1"
    # "Tx1 to Rx1 QueInd_0"
    # "100 times"
    n277 = Dequeue Element(queue=w849) -> (element=w851:cdb[][])  [unwired: 2 in, 3 out]
    n278 = Get Queue Status(queue=w849) -> (# elements in queue=→"# of queue 1":i32)  [unwired: 2 in, 7 out]
    n279 = Get Queue Status(queue=w776) -> (# elements in queue=w779:i32)  [unwired: 2 in, 7 out]
    n280 = call "NCS_IQ_TwoTx.vi"("Coerced IQ rate"=w814, "Waveform Size"=w815, "Channel 1\nTone Frequency"=w782, "Channel 1\nTone Amplitude"=w783, "Channel 0\nTone Frequency"=w781, "Channel 0\nTone Amplitude"=w783) -> ("IQ waveform array"=w800:cdb[][])  [unwired: 2 in, 2 out]
    n281 = Less?(x=w779, y="Flush Th") -> (x < y?=w777:bool)
    n282 = Index Array(array=w800, index (row)=1) -> (element=w784:cdb[])  [unwired: 1 in]
    n283 = Index Array(array=w851, index (row)=1) -> (element=w818:cdb[])  [unwired: 1 in]
    n284 = Index Array(array=w851, index (row)=0) -> (element=w808:cdb[])  [unwired: 1 in]
    n285 = Index Array(array=w800, index (row)=0) -> (element=w785:cdb[])  [unwired: 1 in]
    n286 = local read "Channel 2 \nTone Frequency"() -> (w823:dbl)
    n287 = local read "Channel 1 \nTone Frequency"() -> (w845:dbl)
    n288 = local read "BW/2"() -> (w840:dbl)
    n289 = local read "BW/2"() -> (w822:dbl)
    n290 = local read "Rx IQ Rate 1"() -> (w820:dbl)
    n291 = local read "Rx IQ Rate 1"() -> (w824:dbl)
    n292 = Subtract(x=w845, y=w840) -> (x-y=w846:dbl)
    n293 = Add(x=w845, y=w840) -> (x+y=w847:dbl)
    n294 = Subtract(x=w823, y=w822) -> (x-y=w838:dbl)
    n295 = Add(x=w823, y=w822) -> (x+y=w839:dbl)
    n296 = Complex To Polar(r * e^(i*theta)=w785) -> (theta=w810:dbl[])  [unwired: 1 out]
    n297 = call-poly <vilib>:"Butterworth Filter.vi"("init/cont (init:F)"=TRUE, "order"=2, "filter type"=Filter_Passband_Type."Bandpass", "low cutoff freq: fl"=w846, "high cutoff freq: fh"=w847, "sampling freq: fs"=w824, "X"=w808) -> ("Filtered X"=w842:cdb[])  [unwired: 1 in, 1 out]
    n298 = call-poly <vilib>:"Butterworth Filter.vi"("init/cont (init:F)"=TRUE, "order"=2, "filter type"=Filter_Passband_Type."Bandpass", "low cutoff freq: fl"=w838, "high cutoff freq: fh"=w839, "sampling freq: fs"=w820, "X"=w818) -> ("Filtered X"=w835:cdb[])  [unwired: 1 in, 1 out]
    n299 = case shown="False" w777 {
      tunnel: [dbl[] [0.0] w860] -> w775
      tunnel: w776 -> [w855 w859]
      frame True {
        n300 = Flush Queue(queue=w855) -> ()  [unwired: 1 in, 3 out]
      }
      frame False {
        n301 = local read "DownSamplingRatio"() -> (w857:i32)
        n302 = local read "Waveform Size 1"() -> (w858:dbl)
        n303 = Divide(x=w858, y=w857) -> (x/y=w856:dbl)
        n304 = for {
          N: w856 -> [_]
          tunnel: w859 -> [w862]
          tunnel: [w861] -> w860 mode=indexing
          n305 = Dequeue Element(queue=w862) -> (element=w861:dbl)  [unwired: 2 in, 3 out]
        }
      }
    }
    n306 = Complex To Polar(r * e^(i*theta)=w835) -> (r=w829:dbl[], theta=w796:dbl[])
    n307 = Complex To Polar(r * e^(i*theta)=w784) -> (theta=w797:dbl[])  [unwired: 1 out]
    n308 = Complex To Polar(r * e^(i*theta)=w842) -> (r=w833:dbl[], theta=w809:dbl[])
    n309 = Subtract(x=w809, y=w810) -> (x-y=w812:dbl[])
    n310 = call <vilib>:"Unwrap Phase.vi"("phase unit"=1 ("y"), "Phase"=w812) -> ("Unwrapped Phase"=w806:dbl[])  [unwired: 8 in, 1 out]
    n311 = Subtract(x=w796, y=w797) -> (x-y=w799:dbl[])
    n312 = call <vilib>:"Unwrap Phase.vi"("phase unit"=1 ("y"), "Phase"=w799) -> ("Unwrapped Phase"=w793:dbl[])  [unwired: 8 in, 1 out]
    n313 = local read "DownSamplingRatio"() -> (w802:i32)
    n314 = local read "DownSamplingRatio"() -> (w791:i32)
    n315 = local read "Waveform Size 1"() -> (w821:dbl)
    n316 = local read "Waveform Size 1"() -> (w819:dbl)
    n317 = Divide(x=w821, y=w802) -> (x/y=w805:dbl)
    n318 = Divide(x=w819, y=w791) -> (x/y=w792:dbl)
    n319 = Reshape Array(w833, w805, w802) -> (w807:dbl[][])
    n320 = Reshape Array(w806, w805, w802) -> (w804:dbl[][])
    n321 = Reshape Array(w829, w792, w791) -> (w831:dbl[][])
    n322 = Reshape Array(w793, w792, w791) -> (w794:dbl[][])
    n323 = for {
      tunnel: w807 -> [w875] mode=indexing
      tunnel: [w874] -> w832 mode=indexing
      tunnel: w804 -> [w873] mode=indexing
      tunnel: [w872] -> w803 mode=indexing
      n324 = Add Array Elements(numeric array=w875) -> (sum=w874:dbl)
      n325 = Add Array Elements(numeric array=w873) -> (sum=w872:dbl)
    }
    n326 = for {
      tunnel: w831 -> [w871] mode=indexing
      tunnel: [w870] -> w830 mode=indexing
      tunnel: [w869] -> w795 mode=indexing
      tunnel: w794 -> [w868] mode=indexing
      n327 = Add Array Elements(numeric array=w868) -> (sum=w869:dbl)
      n328 = Add Array Elements(numeric array=w871) -> (sum=w870:dbl)
    }
    n329 = Divide(x=w832, y=w802) -> (x/y=w828:dbl[])
    n330 = Divide(x=w803, y=w802) -> (x/y=w789:dbl[])
    n331 = Divide(x=w830, y=w791) -> (x/y=w827:dbl[])
    n332 = Divide(x=w795, y=w791) -> (x/y=w790:dbl[])
    n333 = Build Array(w828, w827) -> (w788:dbl[][])
    "Amp both" <- w788
    n334 = Build Array(w789, w790) -> (w780:dbl[][])
    "Phase Both" <- w780
    n335 = Build Array (concatenate)(w788, w780, w775) -> (w787:dbl[][])
    n336 = Array Size(array=w787) -> (size(s)=→"ArraySz":i32[])
    n337 = local read "Flush"() -> (w816:bool)
    n338 = local read "Buffer"() -> (w817:bool)
    n339 = Enqueue Element(queue=w826, element=w787) -> ()  [unwired: 2 in, 3 out]
    n340 = case shown="False" w817 {
      tunnel: w825 -> [w864 w867]
      tunnel: w787 -> [_ w866]
      tunnel: w816 -> [w863 _]
      frame False {
        n341 = case shown="True" w863 {
          tunnel: w864 -> [_ w865]
          frame False {
          }
          frame True {
            n342 = Flush Queue(queue=w865) -> ()  [unwired: 1 in, 3 out]
          }
        }
      }
      frame True {
        n343 = Enqueue Element(queue=w867, element=w866) -> ()  [unwired: 2 in, 3 out]
      }
    }
  }
  n344 = while {
    shift-right: [w883] -> _
    shift-left: T4."Default" -> [w884]
    stop <- FALSE stop-if-true
    n345 = case shown="5" w884 {
      tunnel: ["Protocol" w901 w924 w1009 w1037 w1061 w1093 w1180 w1267 w1350 w1379 w1465 w1534 w1603 w1672 w1741] -> w883
      tunnel: [0 1 2 8 9 5 6 7 8 9 10 11 12 13 14 15] -> w882
      tunnel: [w888 w899 w918 w1003 w1031 w1055 w1085 w1171 w1258 w1344 w1368 w1456 w1525 w1594 w1663 w1732] -> w880
      tunnel: [w891 w906 w914 "Listen to the calm relaxing music." "Perform the online attention test." "Perform spontaneous breathing" w1086 w1169 w1257 "Read aloud the following text in between the lines:\n-----------------------------------------------------------------------\nFour score and seven years ago our fathers brought forth on this continent, a new nation, conceived in Liberty, and dedicated to the proposition that all men are created equal… That this nation, under God, shall have a new birth of freedom-and that government of the people, by the people, for the people, shall not perish from the earth.\n\nI am Sam. Sam I am. That Sam-I-am! That Sam-I-am! I do not like that Sam-I-am!\nDo you like green eggs and ham? I do not like them, Sam-I-am. I do not like green eggs and ham. Would you like them here or there? I would not like them here or there. I would not like them anywhere. I do not like green eggs and ham. I do not like them, Sam-I-am.\nWould you like them in a house? Would you like them with a mouse? I do not like them in a house. I do not like them with a mouse. I do not like them here or there. I do not like them anywhere. I do not like green eggs and ham. I do not like them, Sam-I-am.\n-----------------------------------------------------------------------\nWhen finished, take a deep breath and open mouth say \"Ah\" (like doctor checking your throat).\nPerform normal breathing until next instruction." w1369 w1455 w1524 w1593 w1662 w1731] -> w881
      tunnel: [w889 w907 w919 w1006 w1034 w1058 w1089 w1176 w1263 w1347 w1375 w1461 w1530 w1599 w1668 w1737] -> w879
      tunnel: [w888 w899 w915 w1003 w1031 w1055 w1082 w1170 w1256 w1344 w1370 w1454 w1523 w1592 w1661 w1730] -> w878
      tunnel: ["" "" w912 "" "" "" w1081 w1168 w1255 "" w1367 w1453 w1522 w1591 w1660 w1729] -> w876
      frame 0, Default {
        w891 = "Wait for instructions."  # Default
        w888 = 0.0
        # "Waiting - intermediate state"
        n346 = Seconds To Date/Time(time stamp (now)=0.0) -> (date time rec=w889:T2)  [unwired: 1 in]
        "Output" <- 0 ("Output")
        "Buffer" <- FALSE
        "Flush" <- FALSE ("Flush")
        "Save" <- FALSE ("Save")
      }
      frame 1 {
        w899 = 0.0
        w906 = "This is Test run. \nPress STOP TEST to exit and return to default."  # Default
        # "Test"
        n347 = Seconds To Date/Time(time stamp (now)=0.0) -> (date time rec=w907:T2)  [unwired: 1 in]
        n348 = local write "Output"(1) -> ()
        n349 = local write "Buffer"(FALSE ("Buffer")) -> ()
        n350 = local write "Flush"(FALSE ("Flush")) -> ()
        n351 = local write "Save"(FALSE ("Save")) -> ()
        n352 = case shown="True" "Stop Test" {
          tunnel: [T10."Test" w911] -> w901
          frame False {
          }
          frame True {
            w911 = T4."Default"
            n353 = local write "Protocol"(w911) -> ()
          }
        }
      }
      frame 2 {
        w921 = 520.0  # Routine Time
        # "Routine 1"
        n354 = property on="Total Routine Time" class="Slide (strict)"("Scale.Maximum"=w921) -> ()  [unwired: 2 in, 2 out]
        n355 = call "Elapsed Time5"("Time Target (s)"=w921, "Auto Reset"=FALSE) -> ("Get Start Time (s)"=w920:dbl, "Elapsed Time (s)"=w918:dbl, "Time has Elapsed"=w922:bool)  [unwired: 10 in, 5 out]
        "#1" <- w922
        n356 = Seconds To Date/Time(time stamp (now)=w920) -> (date time rec=w919:T2)  [unwired: 1 in]
        n357 = Not(x=w922) -> (.not. x?=w925:bool)
        n358 = script code="t = [0,4,10,14,20,80,84,90,94,100,104,110,114,120,124,130,134,140,140.75,141.5,...\n    142.25,143,143.75,144.5,145.25,146,146.75,147.5,148.25,149,149.75,150.5,151.25,...\n    152,152.75,153,154.25,155,155.75,156.5,157.25,158,158.75,159.5,160.25,161,...\n    161.75,162.5,163.25,164,164.75,165.5,166.25,167,167.75,168.5,169.25,170,...\n    200,203.75,207.5,211.25,215,218.75,222.5,226.25,230,260,280,300,320,340,...\n    344,359,363,378,381,396,399,415,460,470,473,477,487,490,494,504,507,511,520];\n\nevent = [1,2,1,2,0,1,2,1,2,1,2,1,2,1,2,1,2,3,4,3,...\n        4,3,4,3,4,3,4,3,4,3,4,3,4,...\n        3,4,3,4,3,4,3,4,3,4,3,4,3,...\n        4,3,4,3,4,3,4,3,4,3,4,0,...\n        5,6,5,6,5,6,5,6,0,7,0,7,0,8,...\n        0,8,0,9,0,9,0,10,0,12,13,0,12,13,0,12,13,0,14];\n\nfor i = 2:length(t)\n    if ((x>=t(i-1)) &&  (x<t(i)))\n        y = event(i-1);\n        yNext = event(i);\n        dt = t(i) - t(i-1);\n        break;\n    end\nend"("x"=w918) -> ("y"=w913:dbl, "dt"=w916:dbl, "yNext"=w917:dbl)  [unwired: 1 in, 1 out]
        n359 = case shown="True" w925 {
          tunnel: [w984 w996] -> w924
          frame False {
            n360 = flat-sequence {
              tunnel: [w992] -> w984
              frame #0 {
                n361 = local write "Buffer"(FALSE ("Buffer")) -> ()
                n362 = local write "Play/Stop"(FALSE ("Play/Stop")) -> ()
              }
              frame #1 {
                n363 = local write "Output"(0 ("Output")) -> ()
                n364 = local write "Save"(TRUE ("Save")) -> ()
              }
              frame #2 {
                n365 = Wait (ms)(milliseconds to wait=u32 500) -> ()  [unwired: 1 out]
              }
              frame #3 {
                n366 = local write "Flush"(TRUE ("Flush")) -> ()
              }
              frame #4 {
                w991 = u16 0 items=["No sound", "Demo deep breathing", "Demo fast shallow breathing", "Demo slow shallow breathing", "Demo breath hold", "Demo cough/ laugh", "Demo abdomen movement", "Calibration", "Routine 1", "Routine 3", "Routine 4/5/7", "Calm music"] ("Play sound")
                w992 = u16 0 items=["Default", "Test", "Routine 1", "Routine 2", "Routine 3", "Routine 4", "Routine 5", "Routine 6a", "Routine 6b", "Routine 7", "Routine 8"] ("Protocol")
                n367 = local write "Flush"(FALSE ("Flush")) -> ()
                n368 = local write "Save"(FALSE ("Save")) -> ()
                n369 = local write "Protocol"(w992) -> ()
                n370 = local write "Play sound"(w991) -> ()
              }
            }
          }
          frame True {
            w995 = u16 8 items=["No sound", "Demo deep breathing", "Demo fast shallow breathing", "Demo slow shallow breathing", "Demo breath hold", "Demo cough/ laugh", "Demo abdomen movement", "Calibration", "Routine 1", "Routine 3", "Routine 4/5/7", "Calm music"] ("Play sound")
            n371 = local write "Play sound"(w995) -> ()
            n372 = flat-sequence {
              tunnel: [T4."Routine 1"] -> w996
              frame #0 {
                n373 = local write "Output"(1 ("Open")) -> ()
                n374 = local write "Play/Stop"(TRUE ("Play/Stop")) -> ()
              }
              frame #1 {
                n375 = local write "Buffer"(TRUE ("Buffer")) -> ()
              }
              frame #2 {
              }
            }
          }
        }
        n376 = case shown="0, Default" w913 {
          tunnel: ["\nPerform normal breathing, NO deep breathing or breath hold." "Inhale a slow deep breath." "\nExhale slowly." "Quick inhale.\n\n\n\nIf you cannot sustain for long, resume normal breathing." "\nQuick exhale.\n\n\nIf you cannot sustain for long, resume normal breathing." "Slow shallow inhale.\n\n\n\nIf you cannot sustain for long, resume normal breathing." "\nSlow exhale.\n\n\nIf you cannot sustain for long, resume normal breathing." "Exhale the current breath  and HOLD.\n\n\nIf you cannot sustain for long, resume normal breathing." "Perform voluntary coughing \n" "Perform voluntary laugh\n\n" "Read aloud the following text in between the lines:\n-----------------------------------------------------------------------\nFour score and seven years ago our fathers brought forth on this continent, a new nation, conceived in Liberty, and dedicated to the proposition that all men are created equal… That this nation, under God, shall have a new birth of freedom-and that government of the people, by the people, for the people, shall not perish from the earth.\n\n-----------------------------------------------------------------------\nWhen finished, take a deep breath and open mouth say \"Ah\" (like doctor checking your throat).\nPerform normal breathing until next instruction." "Exhale current breath and HOLD. Push abdomen inwards." "Relax abdomen back to normal and keep holding breath."] -> w914
          frame 0, Default {
          }
          frame 1 {
          }
          frame 2 {
          }
          frame 3 {
          }
          frame 4 {
          }
          frame 5 {
          }
          frame 6 {
          }
          frame 7 {
          }
          frame 8 {
          }
          frame 9 {
          }
          frame 10 {
          }
          frame 12 {
          }
          frame 13 {
          }
        }
        n377 = case shown="14" w917 {
          tunnel: ["\nPerform normal breathing, NO deep breathing or breath hold." "Inhale a slow deep breath." "\nExhale slowly." "Quick inhale.\n\n\n\nIf you cannot sustain for long, resume normal breathing." "\nQuick exhale.\n\n\nIf you cannot sustain for long, resume normal breathing." "Slow shallow inhale.\n\n\n\nIf you cannot sustain for long, resume normal breathing." "\nSlow exhale.\n\n\nIf you cannot sustain for long, resume normal breathing." "Exhale the current breath  and HOLD.\n\n\nIf you cannot sustain for long, resume normal breathing." "Perform voluntary coughing \n" "Perform voluntary laugh\n\n" "Read aloud the following text in between the lines:\n-----------------------------------------------------------------------\nFour score and seven years ago our fathers brought forth on this continent, a new nation, conceived in Liberty, and dedicated to the proposition that all men are created equal… That this nation, under God, shall have a new birth of freedom-and that government of the people, by the people, for the people, shall not perish from the earth.\n\n-----------------------------------------------------------------------\nWhen finished, take a deep breath and open mouth say \"Ah\" (like doctor checking your throat).\nPerform normal breathing until next instruction." "Exhale current breath and HOLD. Push abdomen inwards." "Relax abdomen back to normal and keep holding breath." "Study completed!"] -> w912
          frame 0, Default {
          }
          frame 1 {
          }
          frame 2 {
          }
          frame 3 {
          }
          frame 4 {
          }
          frame 5 {
          }
          frame 6 {
          }
          frame 7 {
          }
          frame 8 {
          }
          frame 9 {
          }
          frame 10 {
          }
          frame 12 {
          }
          frame 13 {
          }
          frame 14 {
          }
        }
        n378 = case shown="2" w913 {
          tunnel: w916 -> [w929 w931 w933 w935 w937 w939 w941 w943 w945 w947 w949 w951 w953 w956]
          tunnel: [w928 w930 w932 w934 w936 w938 w940 w942 w944 w946 w948 w950 w952 w955] -> w915
          frame 1 {
            n379 = property on="Current Task time" class="Slide (strict)"("Scale.Maximum"=w929) -> ()  [unwired: 2 in, 2 out]
            n380 = call "Elapsed Time11"("Time Target (s)"=w929) -> ("Elapsed Time (s)"=w928:dbl)  [unwired: 11 in, 7 out]
            n381 = property on="Current Task time" class="Slide (strict)"("Scale.Minimum"=0.0 ("Scale.Range:Minimum")) -> ()  [unwired: 2 in, 2 out]
          }
          frame 2 {
            n382 = property on="Current Task time" class="Slide (strict)"("Scale.Maximum"=w931) -> ()  [unwired: 2 in, 2 out]
            n383 = call "Elapsed Time12"("Time Target (s)"=w931) -> ("Elapsed Time (s)"=w930:dbl)  [unwired: 11 in, 7 out]
          }
          frame 3 {
            n384 = property on="Current Task time" class="Slide (strict)"("Scale.Maximum"=w933) -> ()  [unwired: 2 in, 2 out]
            n385 = call "Elapsed Time13"("Time Target (s)"=w933) -> ("Elapsed Time (s)"=w932:dbl)  [unwired: 11 in, 7 out]
          }
          frame 4 {
            n386 = property on="Current Task time" class="Slide (strict)"("Scale.Maximum"=w935) -> ()  [unwired: 2 in, 2 out]
            n387 = call "Elapsed Time14"("Time Target (s)"=w935) -> ("Elapsed Time (s)"=w934:dbl)  [unwired: 11 in, 7 out]
          }
          frame 5 {
            n388 = property on="Current Task time" class="Slide (strict)"("Scale.Maximum"=w937) -> ()  [unwired: 2 in, 2 out]
            n389 = call "Elapsed Time15"("Time Target (s)"=w937) -> ("Elapsed Time (s)"=w936:dbl)  [unwired: 11 in, 7 out]
          }
          frame 6 {
            n390 = property on="Current Task time" class="Slide (strict)"("Scale.Maximum"=w939) -> ()  [unwired: 2 in, 2 out]
            n391 = call "Elapsed Time16"("Time Target (s)"=w939) -> ("Elapsed Time (s)"=w938:dbl)  [unwired: 11 in, 7 out]
          }
          frame 7 {
            n392 = property on="Current Task time" class="Slide (strict)"("Scale.Maximum"=w941) -> ()  [unwired: 2 in, 2 out]
            n393 = call "Elapsed Time17"("Time Target (s)"=w941) -> ("Elapsed Time (s)"=w940:dbl)  [unwired: 11 in, 7 out]
          }
          frame 8 {
            n394 = property on="Current Task time" class="Slide (strict)"("Scale.Maximum"=w943) -> ()  [unwired: 2 in, 2 out]
            n395 = call "Elapsed Time18"("Time Target (s)"=w943) -> ("Elapsed Time (s)"=w942:dbl)  [unwired: 11 in, 7 out]
          }
          frame 9 {
            n396 = property on="Current Task time" class="Slide (strict)"("Scale.Maximum"=w945) -> ()  [unwired: 2 in, 2 out]
            n397 = call "Elapsed Time19"("Time Target (s)"=w945) -> ("Elapsed Time (s)"=w944:dbl)  [unwired: 11 in, 7 out]
          }
          frame 10 {
            n398 = property on="Current Task time" class="Slide (strict)"("Scale.Maximum"=w947) -> ()  [unwired: 2 in, 2 out]
            n399 = call "Elapsed Time20"("Time Target (s)"=w947) -> ("Elapsed Time (s)"=w946:dbl)  [unwired: 11 in, 7 out]
          }
          frame 11 {
            n400 = property on="Current Task time" class="Slide (strict)"("Scale.Maximum"=w949) -> ()  [unwired: 2 in, 2 out]
            n401 = call "Elapsed Time21"("Time Target (s)"=w949) -> ("Elapsed Time (s)"=w948:dbl)  [unwired: 11 in, 7 out]
          }
          frame 12 {
            n402 = property on="Current Task time" class="Slide (strict)"("Scale.Maximum"=w951) -> ()  [unwired: 2 in, 2 out]
            n403 = call "Elapsed Time22"("Time Target (s)"=w951) -> ("Elapsed Time (s)"=w950:dbl)  [unwired: 11 in, 7 out]
          }
          frame 13 {
            n404 = property on="Current Task time" class="Slide (strict)"("Scale.Maximum"=w953) -> ()  [unwired: 2 in, 2 out]
            n405 = call "Elapsed Time23"("Time Target (s)"=w953) -> ("Elapsed Time (s)"=w952:dbl)  [unwired: 11 in, 7 out]
          }
          frame 0, Default {
            n406 = property on="Current Task time" class="Slide (strict)"("Scale.Maximum"=w956) -> ()  [unwired: 2 in, 2 out]
            n407 = call "Elapsed Time24"("Time Target (s)"=w956) -> ("Elapsed Time (s)"=w955:dbl)  [unwired: 11 in, 7 out]
            n408 = property on="Current Task time" class="Slide (strict)"("Scale.Minimum"=0.0 ("Scale.Range:Minimum")) -> ()  [unwired: 2 in, 2 out]
          }
        }
      }
      frame 3 {
        w1002 = 180.0  # Routine Time
        # "Routine 2a: Attention test - relaxing music"
        n409 = property on="Total Routine Time" class="Slide (strict)"("Scale.Maximum"=w1002) -> ()  [unwired: 2 in, 2 out]
        n410 = property on="Current Task time" class="Slide (strict)"("Scale.Maximum"=w1002) -> ()  [unwired: 2 in, 2 out]
        n411 = call "Elapsed Time7"("Time Target (s)"=w1002, "Auto Reset"=FALSE ("Timer Reset")) -> ("Get Start Time (s)"=w1005:dbl, "Elapsed Time (s)"=w1003:dbl, "Time has Elapsed"=w1007:bool)  [unwired: 10 in, 5 out]
        "#2a" <- w1007
        n412 = Seconds To Date/Time(time stamp (now)=w1005) -> (date time rec=w1006:T2)  [unwired: 1 in]
        n413 = Not(x=w1007) -> (.not. x?=w1010:bool)
        n414 = case shown="True" w1010 {
          tunnel: [w1012 w1024] -> w1009
          frame False {
            n415 = flat-sequence {
              tunnel: [w1020] -> w1012
              frame #0 {
                n416 = local write "Buffer"(FALSE ("Buffer")) -> ()
                n417 = local write "Play/Stop"(FALSE ("PlayMusic")) -> ()
              }
              frame #1 {
                n418 = local write "Output"(0 ("Output")) -> ()
                n419 = local write "Save"(TRUE ("Save")) -> ()
              }
              frame #2 {
                n420 = Wait (ms)(milliseconds to wait=u32 500) -> ()  [unwired: 1 out]
              }
              frame #3 {
                n421 = local write "Flush"(TRUE ("Flush")) -> ()
              }
              frame #4 {
                w1019 = u16 0 items=["No sound", "Demo deep breathing", "Demo fast shallow breathing", "Demo slow shallow breathing", "Demo breath hold", "Demo cough/ laugh", "Demo abdomen movement", "Calibration", "Routine 1", "Routine 3", "Routine 4/5/7", "Calm music"] ("Play sound")
                w1020 = T4."Default"
                n422 = local write "Flush"(FALSE ("Flush")) -> ()
                n423 = local write "Save"(FALSE ("Save")) -> ()
                n424 = local write "Protocol"(w1020) -> ()
                n425 = local write "Play sound"(w1019) -> ()
              }
            }
          }
          frame True {
            w1023 = u16 11 items=["No sound", "Demo deep breathing", "Demo fast shallow breathing", "Demo slow shallow breathing", "Demo breath hold", "Demo cough/ laugh", "Demo abdomen movement", "Calibration", "Routine 1", "Routine 3", "Routine 4/5/7", "Calm music"] ("Play sound")
            n426 = local write "Play sound"(w1023) -> ()
            n427 = flat-sequence {
              tunnel: [T4."Routine 2a"] -> w1024
              frame #0 {
                n428 = local write "Output"(1 ("Open")) -> ()
                n429 = local write "Play/Stop"(TRUE ("PlayMusic")) -> ()
              }
              frame #1 {
                n430 = local write "Buffer"(TRUE ("Buffer")) -> ()
              }
              frame #2 {
              }
            }
          }
        }
      }
      frame 4 {
        w1030 = 320.0  # Routine Time
        # "Routine 2b: Attention test"
        n431 = property on="Total Routine Time" class="Slide (strict)"("Scale.Maximum"=w1030) -> ()  [unwired: 2 in, 2 out]
        n432 = property on="Current Task time" class="Slide (strict)"("Scale.Maximum"=w1030) -> ()  [unwired: 2 in, 2 out]
        n433 = call "Elapsed Time9"("Time Target (s)"=w1030, "Auto Reset"=FALSE ("Timer Reset")) -> ("Get Start Time (s)"=w1033:dbl, "Elapsed Time (s)"=w1031:dbl, "Time has Elapsed"=w1035:bool)  [unwired: 10 in, 5 out]
        "#2b" <- w1035
        n434 = Seconds To Date/Time(time stamp (now)=w1033) -> (date time rec=w1034:T2)  [unwired: 1 in]
        n435 = Not(x=w1035) -> (.not. x?=w1038:bool)
        n436 = case shown="False" w1038 {
          tunnel: [w1040 w1049] -> w1037
          frame False {
            n437 = flat-sequence {
              tunnel: [w1046] -> w1040
              frame #0 {
                n438 = local write "Buffer"(FALSE ("Buffer")) -> ()
              }
              frame #1 {
                n439 = local write "Output"(0 ("Output")) -> ()
                n440 = local write "Save"(TRUE ("Save")) -> ()
              }
              frame #2 {
                n441 = Wait (ms)(milliseconds to wait=u32 500) -> ()  [unwired: 1 out]
              }
              frame #3 {
                n442 = local write "Flush"(TRUE ("Flush")) -> ()
              }
              frame #4 {
                w1046 = T4."Default"
                n443 = local write "Flush"(FALSE ("Flush")) -> ()
                n444 = local write "Save"(FALSE ("Save")) -> ()
                n445 = local write "Protocol"(w1046) -> ()
              }
            }
          }
          frame True {
            n446 = flat-sequence {
              tunnel: [T4."Routine 2b"] -> w1049
              frame #0 {
                n447 = local write "Output"(1 ("Open")) -> ()
              }
              frame #1 {
                n448 = local write "Buffer"(TRUE ("Buffer")) -> ()
              }
              frame #2 {
              }
            }
          }
        }
      }
      frame 5 {
        w1054 = 300.0  # Routine Time
        # "Routine 3a: Exercising"
        n449 = property on="Total Routine Time" class="Slide (strict)"("Scale.Maximum"=w1054) -> ()  [unwired: 2 in, 2 out]
        n450 = call "Elapsed Time3"("Time Target (s)"=w1054, "Auto Reset"=FALSE ("Timer Reset")) -> ("Get Start Time (s)"=w1057:dbl, "Elapsed Time (s)"=w1055:dbl, "Time has Elapsed"=w1059:bool)  [unwired: 10 in, 5 out]
        "#3a" <- w1059
        n451 = Seconds To Date/Time(time stamp (now)=w1057) -> (date time rec=w1058:T2)  [unwired: 1 in]
        n452 = Not(x=w1059) -> (.not. x?=w1062:bool)
        n453 = property on="Current Task time" class="Slide (strict)"("Scale.Maximum"=w1054) -> ()  [unwired: 2 in, 2 out]
        n454 = case shown="False" w1062 {
          tunnel: [w1064 w1076] -> w1061
          frame False {
            n455 = flat-sequence {
              tunnel: [w1072] -> w1064
              frame #0 {
                n456 = local write "Buffer"(FALSE ("Buffer")) -> ()
                n457 = local write "Play/Stop"(FALSE ("Play/Stop")) -> ()
              }
              frame #1 {
                n458 = local write "Output"(0 ("Output")) -> ()
                n459 = local write "Save"(TRUE ("Save")) -> ()
              }
              frame #2 {
                n460 = Wait (ms)(milliseconds to wait=u32 500) -> ()  [unwired: 1 out]
              }
              frame #3 {
                n461 = local write "Flush"(TRUE ("Flush")) -> ()
              }
              frame #4 {
                w1071 = u16 0 items=["No sound", "Demo deep breathing", "Demo fast shallow breathing", "Demo slow shallow breathing", "Demo breath hold", "Demo cough/ laugh", "Demo abdomen movement", "Calibration", "Routine 1", "Routine 3b", "Routine 4/5/7", "Calm music", "Routine 3a"] ("Play sound")
                w1072 = T4."Default"
                n462 = local write "Flush"(FALSE ("Flush")) -> ()
                n463 = local write "Save"(FALSE ("Save")) -> ()
                n464 = local write "Play sound"(w1071) -> ()
                n465 = local write "Protocol"(w1072) -> ()
              }
            }
          }
          frame True {
            w1075 = u16 12 items=["No sound", "Demo deep breathing", "Demo fast shallow breathing", "Demo slow shallow breathing", "Demo breath hold", "Demo cough/ laugh", "Demo abdomen movement", "Calibration", "Routine 1", "Routine 3b", "Routine 4/5/7", "Calm music", "Routine 3a"] ("Play sound")
            n466 = local write "Play sound"(w1075) -> ()
            n467 = flat-sequence {
              tunnel: [T4."Routine 3a"] -> w1076
              frame #0 {
                n468 = local write "Output"(1 ("Open")) -> ()
                n469 = local write "Play/Stop"(TRUE ("Play/Stop")) -> ()
              }
              frame #1 {
                n470 = local write "Buffer"(TRUE ("Buffer")) -> ()
              }
              frame #2 {
              }
            }
          }
        }
      }
      frame 6 {
        w1090 = 395.0  # Routine Time
        # "Routine 3b: On chair after exercising"
        n471 = property on="Total Routine Time" class="Slide (strict)"("Scale.Maximum"=w1090) -> ()  [unwired: 2 in, 2 out]
        n472 = call "Elapsed Time4"("Time Target (s)"=w1090, "Auto Reset"=FALSE ("Timer Reset")) -> ("Get Start Time (s)"=w1088:dbl, "Elapsed Time (s)"=w1085:dbl, "Time has Elapsed"=w1091:bool)  [unwired: 10 in, 5 out]
        "#3b" <- w1091
        n473 = Seconds To Date/Time(time stamp (now)=w1088) -> (date time rec=w1089:T2)  [unwired: 1 in]
        n474 = Not(x=w1091) -> (.not. x?=w1094:bool)
        n475 = script code="t = [20,80,84,90,94,100,104,110,114,120,124,130,134,140,140.75,141.5,...\n    142.25,143,143.75,144.5,145.25,146,146.75,147.5,148.25,149,149.75,150.5,151.25,...\n    152,152.75,153,154.25,155,155.75,156.5,157.25,158,158.75,159.5,160.25,161,...\n    161.75,162.5,163.25,164,164.75,165.5,166.25,167,167.75,168.5,169.25,170,...\n    200,203.75,207.5,211.25,215,218.75,222.5,226.25,230,260,280,300,320,340,...\n    344,359,363,378,381,396,399,415];\n\nt = t - 20; \n\nevent = [0,1,2,1,2,1,2,1,2,1,2,1,2,3,4,3,...\n        4,3,4,3,4,3,4,3,4,3,4,3,4,...\n        3,4,3,4,3,4,3,4,3,4,3,4,3,...\n        4,3,4,3,4,3,4,3,4,3,4,0,...\n        5,6,5,6,5,6,5,6,0,7,0,7,0,8,...\n        0,8,0,9,0,9,0,14];\n\nfor i = 2:length(t)\n    if ((x>=t(i-1)) &&  (x<t(i)))\n        y = event(i-1);\n        yNext = event(i);\n        dt = t(i) - t(i-1);\n        break;\n    end\nend"("x"=w1085) -> ("y"=w1083:dbl, "dt"=w1084:dbl, "yNext"=w1087:dbl)  [unwired: 1 in, 1 out]
        n476 = case shown="True" w1094 {
          tunnel: [w1151 w1163] -> w1093
          frame False {
            n477 = flat-sequence {
              tunnel: [w1159] -> w1151
              frame #0 {
                n478 = local write "Play/Stop"(FALSE ("PlayInstr")) -> ()
                n479 = local write "Buffer"(FALSE ("Buffer")) -> ()
              }
              frame #1 {
                n480 = local write "Output"(0 ("Output")) -> ()
                n481 = local write "Save"(TRUE ("Save")) -> ()
              }
              frame #2 {
                n482 = Wait (ms)(milliseconds to wait=u32 500) -> ()  [unwired: 1 out]
              }
              frame #3 {
                n483 = local write "Flush"(TRUE ("Flush")) -> ()
              }
              frame #4 {
                w1158 = u16 0 items=["No sound", "Demo deep breathing", "Demo fast shallow breathing", "Demo slow shallow breathing", "Demo breath hold", "Demo cough/ laugh", "Demo abdomen movement", "Calibration", "Routine 1", "Routine 3", "Routine 4/5/7", "Calm music"] ("Play sound")
                w1159 = T4."Default"
                n484 = local write "Flush"(FALSE ("Flush")) -> ()
                n485 = local write "Save"(FALSE ("Save")) -> ()
                n486 = local write "Protocol"(w1159) -> ()
                n487 = local write "Play sound"(w1158) -> ()
              }
            }
          }
          frame True {
            w1162 = u16 9 items=["No sound", "Demo deep breathing", "Demo fast shallow breathing", "Demo slow shallow breathing", "Demo breath hold", "Demo cough/ laugh", "Demo abdomen movement", "Calibration", "Routine 1", "Routine 3", "Routine 4/5/7", "Calm music"] ("Play sound")
            n488 = local write "Play sound"(w1162) -> ()
            n489 = flat-sequence {
              tunnel: [T4."Routine 3b"] -> w1163
              frame #0 {
                n490 = local write "Output"(1 ("Open")) -> ()
                n491 = local write "Play/Stop"(TRUE ("PlayInstr")) -> ()
              }
              frame #1 {
                n492 = local write "Buffer"(TRUE ("Buffer")) -> ()
              }
              frame #2 {
              }
            }
          }
        }
        n493 = case shown="6" w1083 {
          tunnel: ["\nPerform normal breathing, NO deep breathing or breath hold." "Inhale a slow deep breath." "\nExhale slowly." "Quick inhale.\n\n\n\nIf you cannot sustain for long, resume normal breathing." "\nQuick exhale.\n\n\nIf you cannot sustain for long, resume normal breathing." "Slow shallow inhale.\n\n\n\nIf you cannot sustain for long, resume normal breathing." "\nSlow exhale.\n\n\nIf you cannot sustain for long, resume normal breathing." "Exhale the current breath  and HOLD.\n\n\nIf you cannot sustain for long, resume normal breathing." "Perform voluntary coughing \n" "Perform voluntary laugh\n\n" "Read aloud the following text in between the lines:\n-----------------------------------------------------------------------\nFour score and seven years ago our fathers brought forth on this continent, a new nation, conceived in Liberty, and dedicated to the proposition that all men are created equal… That this nation, under God, shall have a new birth of freedom-and that government of the people, by the people, for the people, shall not perish from the earth.\n\n-----------------------------------------------------------------------\nWhen finished, take a deep breath and open mouth say \"Ah\" (like doctor checking your throat).\nPerform normal breathing until next instruction." "Exhale current breath and HOLD. Push abdomen inwards." "Relax abdomen back to normal and keep holding breath."] -> w1086
          frame 0, Default {
          }
          frame 1 {
          }
          frame 2 {
          }
          frame 3 {
          }
          frame 4 {
          }
          frame 5 {
          }
          frame 6 {
          }
          frame 7 {
          }
          frame 8 {
          }
          frame 9 {
          }
          frame 10 {
          }
          frame 12 {
          }
          frame 13 {
          }
        }
        n494 = case shown="14" w1087 {
          tunnel: ["\nPerform normal breathing, NO deep breathing or breath hold." "Inhale a slow deep breath." "\nExhale slowly." "Quick inhale.\n\n\n\nIf you cannot sustain for long, resume normal breathing." "\nQuick exhale.\n\n\nIf you cannot sustain for long, resume normal breathing." "Slow shallow inhale.\n\n\n\nIf you cannot sustain for long, resume normal breathing." "\nSlow exhale.\n\n\nIf you cannot sustain for long, resume normal breathing." "Exhale the current breath  and HOLD.\n\n\nIf you cannot sustain for long, resume normal breathing." "Perform voluntary coughing \n" "Perform voluntary laugh\n\n" "Read aloud the following text in between the lines:\n-----------------------------------------------------------------------\nFour score and seven years ago our fathers brought forth on this continent, a new nation, conceived in Liberty, and dedicated to the proposition that all men are created equal… That this nation, under God, shall have a new birth of freedom-and that government of the people, by the people, for the people, shall not perish from the earth.\n\n-----------------------------------------------------------------------\nWhen finished, take a deep breath and open mouth say \"Ah\" (like doctor checking your throat).\nPerform normal breathing until next instruction." "Exhale current breath and HOLD. Push abdomen inwards." "Relax abdomen back to normal and keep holding breath." "Study completed!"] -> w1081
          frame 0, Default {
          }
          frame 1 {
          }
          frame 2 {
          }
          frame 3 {
          }
          frame 4 {
          }
          frame 5 {
          }
          frame 6 {
          }
          frame 7 {
          }
          frame 8 {
          }
          frame 9 {
          }
          frame 10 {
          }
          frame 12 {
          }
          frame 13 {
          }
          frame 14 {
          }
        }
        n495 = case shown="1" w1083 {
          tunnel: w1084 -> [w1097 w1099 w1101 w1103 w1105 w1107 w1109 w1111 w1113 w1115 w1117 w1119 w1121 w1123]
          tunnel: [w1096 w1098 w1100 w1102 w1104 w1106 w1108 w1110 w1112 w1114 w1116 w1118 w1120 w1122] -> w1082
          frame 1 {
            n496 = property on="Current Task time" class="Slide (strict)"("Scale.Maximum"=w1097) -> ()  [unwired: 2 in, 2 out]
            n497 = call "Elapsed Time10"("Time Target (s)"=w1097) -> ("Elapsed Time (s)"=w1096:dbl)  [unwired: 11 in, 7 out]
          }
          frame 2 {
            n498 = property on="Current Task time" class="Slide (strict)"("Scale.Maximum"=w1099) -> ()  [unwired: 2 in, 2 out]
            n499 = call "Elapsed Time25"("Time Target (s)"=w1099) -> ("Elapsed Time (s)"=w1098:dbl)  [unwired: 11 in, 7 out]
          }
          frame 3 {
            n500 = property on="Current Task time" class="Slide (strict)"("Scale.Maximum"=w1101) -> ()  [unwired: 2 in, 2 out]
            n501 = call "Elapsed Time26"("Time Target (s)"=w1101) -> ("Elapsed Time (s)"=w1100:dbl)  [unwired: 11 in, 7 out]
          }
          frame 4 {
            n502 = property on="Current Task time" class="Slide (strict)"("Scale.Maximum"=w1103) -> ()  [unwired: 2 in, 2 out]
            n503 = call "Elapsed Time27"("Time Target (s)"=w1103) -> ("Elapsed Time (s)"=w1102:dbl)  [unwired: 11 in, 7 out]
          }
          frame 5 {
            n504 = property on="Current Task time" class="Slide (strict)"("Scale.Maximum"=w1105) -> ()  [unwired: 2 in, 2 out]
            n505 = call "Elapsed Time28"("Time Target (s)"=w1105) -> ("Elapsed Time (s)"=w1104:dbl)  [unwired: 11 in, 7 out]
          }
          frame 6 {
            n506 = property on="Current Task time" class="Slide (strict)"("Scale.Maximum"=w1107) -> ()  [unwired: 2 in, 2 out]
            n507 = call "Elapsed Time29"("Time Target (s)"=w1107) -> ("Elapsed Time (s)"=w1106:dbl)  [unwired: 11 in, 7 out]
          }
          frame 7 {
            n508 = property on="Current Task time" class="Slide (strict)"("Scale.Maximum"=w1109) -> ()  [unwired: 2 in, 2 out]
            n509 = call "Elapsed Time30"("Time Target (s)"=w1109) -> ("Elapsed Time (s)"=w1108:dbl)  [unwired: 11 in, 7 out]
          }
          frame 8 {
            n510 = property on="Current Task time" class="Slide (strict)"("Scale.Maximum"=w1111) -> ()  [unwired: 2 in, 2 out]
            n511 = call "Elapsed Time31"("Time Target (s)"=w1111) -> ("Elapsed Time (s)"=w1110:dbl)  [unwired: 11 in, 7 out]
          }
          frame 9 {
            n512 = property on="Current Task time" class="Slide (strict)"("Scale.Maximum"=w1113) -> ()  [unwired: 2 in, 2 out]
            n513 = call "Elapsed Time32"("Time Target (s)"=w1113) -> ("Elapsed Time (s)"=w1112:dbl)  [unwired: 11 in, 7 out]
          }
          frame 10 {
            n514 = property on="Current Task time" class="Slide (strict)"("Scale.Maximum"=w1115) -> ()  [unwired: 2 in, 2 out]
            n515 = call "Elapsed Time33"("Time Target (s)"=w1115) -> ("Elapsed Time (s)"=w1114:dbl)  [unwired: 11 in, 7 out]
          }
          frame 11 {
            n516 = property on="Current Task time" class="Slide (strict)"("Scale.Maximum"=w1117) -> ()  [unwired: 2 in, 2 out]
            n517 = call "Elapsed Time70"("Time Target (s)"=w1117) -> ("Elapsed Time (s)"=w1116:dbl)  [unwired: 11 in, 7 out]
          }
          frame 12 {
            n518 = property on="Current Task time" class="Slide (strict)"("Scale.Maximum"=w1119) -> ()  [unwired: 2 in, 2 out]
            n519 = call "Elapsed Time119"("Time Target (s)"=w1119) -> ("Elapsed Time (s)"=w1118:dbl)  [unwired: 11 in, 7 out]
          }
          frame 13 {
            n520 = property on="Current Task time" class="Slide (strict)"("Scale.Maximum"=w1121) -> ()  [unwired: 2 in, 2 out]
            n521 = call "Elapsed Time120"("Time Target (s)"=w1121) -> ("Elapsed Time (s)"=w1120:dbl)  [unwired: 11 in, 7 out]
          }
          frame 0, Default {
            n522 = property on="Current Task time" class="Slide (strict)"("Scale.Maximum"=w1123) -> ()  [unwired: 2 in, 2 out]
            n523 = call "Elapsed Time121"("Time Target (s)"=w1123) -> ("Elapsed Time (s)"=w1122:dbl)  [unwired: 11 in, 7 out]
          }
        }
      }
      frame 7 {
        w1177 = 415.0  # Routine Time
        # "Routine 4: Lying on bed in supine"
        n524 = property on="Total Routine Time" class="Slide (strict)"("Scale.Maximum"=w1177) -> ()  [unwired: 2 in, 2 out]
        n525 = call "Elapsed Time"("Time Target (s)"=w1177, "Auto Reset"=FALSE ("Timer Reset")) -> ("Get Start Time (s)"=w1175:dbl, "Elapsed Time (s)"=w1171:dbl, "Time has Elapsed"=w1178:bool)  [unwired: 10 in, 5 out]
        "#4" <- w1178
        n526 = Seconds To Date/Time(time stamp (now)=w1175) -> (date time rec=w1176:T2)  [unwired: 1 in]
        n527 = Not(x=w1178) -> (.not. x?=w1181:bool)
        n528 = script code="t = [0,4,10,14,20,80,84,90,94,100,104,110,114,120,124,130,134,140,140.75,141.5,...\n    142.25,143,143.75,144.5,145.25,146,146.75,147.5,148.25,149,149.75,150.5,151.25,...\n    152,152.75,153,154.25,155,155.75,156.5,157.25,158,158.75,159.5,160.25,161,...\n    161.75,162.5,163.25,164,164.75,165.5,166.25,167,167.75,168.5,169.25,170,...\n    200,203.75,207.5,211.25,215,218.75,222.5,226.25,230,260,280,300,320,340,...\n    344,359,363,378,381,396,399,415];\n\nevent = [1,2,1,2,0,1,2,1,2,1,2,1,2,1,2,1,2,3,4,3,...\n        4,3,4,3,4,3,4,3,4,3,4,3,4,...\n        3,4,3,4,3,4,3,4,3,4,3,4,3,...\n        4,3,4,3,4,3,4,3,4,3,4,0,...\n        5,6,5,6,5,6,5,6,0,7,0,7,0,8,...\n        0,8,0,9,0,9,0,14];\n\nfor i = 2:length(t)\n    if ((x>=t(i-1)) &&  (x<t(i)))\n        y = event(i-1);\n        yNext = event(i);\n        dt = t(i) - t(i-1);\n        break;\n    end\nend"("x"=w1171) -> ("y"=w1172:dbl, "dt"=w1173:dbl, "yNext"=w1174:dbl)  [unwired: 1 in, 1 out]
        n529 = case shown="False" w1181 {
          tunnel: [w1238 w1250] -> w1180
          frame False {
            n530 = flat-sequence {
              tunnel: [w1246] -> w1238
              frame #0 {
                n531 = local write "Buffer"(FALSE ("Buffer")) -> ()
                n532 = local write "Play/Stop"(FALSE ("PlayInstr")) -> ()
              }
              frame #1 {
                n533 = local write "Output"(0 ("Output")) -> ()
                n534 = local write "Save"(TRUE ("Save")) -> ()
              }
              frame #2 {
                n535 = Wait (ms)(milliseconds to wait=u32 500) -> ()  [unwired: 1 out]
              }
              frame #3 {
                n536 = local write "Flush"(TRUE ("Flush")) -> ()
              }
              frame #4 {
                w1245 = u16 0 items=["No sound", "Demo deep breathing", "Demo fast shallow breathing", "Demo slow shallow breathing", "Demo breath hold", "Demo cough/ laugh", "Demo abdomen movement", "Calibration", "Routine 1", "Routine 3", "Routine 4/5/7", "Calm music"] ("Play sound")
                w1246 = T4."Default"
                n537 = local write "Flush"(FALSE ("Flush")) -> ()
                n538 = local write "Save"(FALSE ("Save")) -> ()
                n539 = local write "Play sound"(w1245) -> ()
                n540 = local write "Protocol"(w1246) -> ()
              }
            }
          }
          frame True {
            w1249 = u16 10 items=["No sound", "Demo deep breathing", "Demo fast shallow breathing", "Demo slow shallow breathing", "Demo breath hold", "Demo cough/ laugh", "Demo abdomen movement", "Calibration", "Routine 1", "Routine 3", "Routine 4/5/7", "Calm music"] ("Play sound")
            n541 = local write "Play sound"(w1249) -> ()
            n542 = flat-sequence {
              tunnel: [T4."Routine 4"] -> w1250
              frame #0 {
                n543 = local write "Output"(1 ("Open")) -> ()
                n544 = local write "Play/Stop"(TRUE ("PlayInstruction")) -> ()
              }
              frame #1 {
                n545 = local write "Buffer"(TRUE ("Buffer")) -> ()
              }
              frame #2 {
              }
            }
          }
        }
        n546 = case shown="0, Default" w1172 {
          tunnel: ["\nPerform normal breathing, NO deep breathing or breath hold." "Inhale a slow deep breath." "\nExhale slowly." "Quick inhale.\n\n\n\nIf you cannot sustain for long, resume normal breathing." "\nQuick exhale.\n\n\nIf you cannot sustain for long, resume normal breathing." "Slow shallow inhale.\n\n\n\nIf you cannot sustain for long, resume normal breathing." "\nSlow exhale.\n\n\nIf you cannot sustain for long, resume normal breathing." "Exhale the current breath  and HOLD.\n\n\nIf you cannot sustain for long, resume normal breathing." "Perform voluntary coughing \n" "Perform voluntary laugh\n\n" "Read aloud the following text in between the lines:\n-----------------------------------------------------------------------\nFour score and seven years ago our fathers brought forth on this continent, a new nation, conceived in Liberty, and dedicated to the proposition that all men are created equal… That this nation, under God, shall have a new birth of freedom-and that government of the people, by the people, for the people, shall not perish from the earth.\n\n-----------------------------------------------------------------------\nWhen finished, take a deep breath and open mouth say \"Ah\" (like doctor checking your throat).\nPerform normal breathing until next instruction." "Exhale current breath and HOLD. Push abdomen inwards." "Relax abdomen back to normal and keep holding breath."] -> w1169
          frame 0, Default {
          }
          frame 1 {
          }
          frame 2 {
          }
          frame 3 {
          }
          frame 4 {
          }
          frame 5 {
          }
          frame 6 {
          }
          frame 7 {
          }
          frame 8 {
          }
          frame 9 {
          }
          frame 10 {
          }
          frame 12 {
          }
          frame 13 {
          }
        }
        n547 = case shown="14" w1174 {
          tunnel: ["\nPerform normal breathing, NO deep breathing or breath hold." "Inhale a slow deep breath." "\nExhale slowly." "Quick inhale.\n\n\n\nIf you cannot sustain for long, resume normal breathing." "\nQuick exhale.\n\n\nIf you cannot sustain for long, resume normal breathing." "Slow shallow inhale.\n\n\n\nIf you cannot sustain for long, resume normal breathing." "\nSlow exhale.\n\n\nIf you cannot sustain for long, resume normal breathing." "Exhale the current breath  and HOLD.\n\n\nIf you cannot sustain for long, resume normal breathing." "Perform voluntary coughing \n" "Perform voluntary laugh\n\n" "Read aloud the following text in between the lines:\n-----------------------------------------------------------------------\nFour score and seven years ago our fathers brought forth on this continent, a new nation, conceived in Liberty, and dedicated to the proposition that all men are created equal… That this nation, under God, shall have a new birth of freedom-and that government of the people, by the people, for the people, shall not perish from the earth.\n\n-----------------------------------------------------------------------\nWhen finished, take a deep breath and open mouth say \"Ah\" (like doctor checking your throat).\nPerform normal breathing until next instruction." "Exhale current breath and HOLD. Push abdomen inwards." "Relax abdomen back to normal and keep holding breath." "Study Completed!"] -> w1168
          frame 0, Default {
          }
          frame 1 {
          }
          frame 2 {
          }
          frame 3 {
          }
          frame 4 {
          }
          frame 5 {
          }
          frame 6 {
          }
          frame 7 {
          }
          frame 8 {
          }
          frame 9 {
          }
          frame 10 {
          }
          frame 12 {
          }
          frame 13 {
          }
          frame 14 {
          }
        }
        n548 = case shown="5" w1172 {
          tunnel: w1173 -> [w1184 w1186 w1188 w1190 w1192 w1194 w1196 w1198 w1200 w1202 w1204 w1206 w1208 w1210]
          tunnel: [w1183 w1185 w1187 w1189 w1191 w1193 w1195 w1197 w1199 w1201 w1203 w1205 w1207 w1209] -> w1170
          frame 1 {
            n549 = property on="Current Task time" class="Slide (strict)"("Scale.Maximum"=w1184) -> ()  [unwired: 2 in, 2 out]
            n550 = call "Elapsed Time34"("Time Target (s)"=w1184) -> ("Elapsed Time (s)"=w1183:dbl)  [unwired: 11 in, 7 out]
          }
          frame 2 {
            n551 = property on="Current Task time" class="Slide (strict)"("Scale.Maximum"=w1186) -> ()  [unwired: 2 in, 2 out]
            n552 = call "Elapsed Time35"("Time Target (s)"=w1186) -> ("Elapsed Time (s)"=w1185:dbl)  [unwired: 11 in, 7 out]
          }
          frame 3 {
            n553 = property on="Current Task time" class="Slide (strict)"("Scale.Maximum"=w1188) -> ()  [unwired: 2 in, 2 out]
            n554 = call "Elapsed Time36"("Time Target (s)"=w1188) -> ("Elapsed Time (s)"=w1187:dbl)  [unwired: 11 in, 7 out]
          }
          frame 4 {
            n555 = property on="Current Task time" class="Slide (strict)"("Scale.Maximum"=w1190) -> ()  [unwired: 2 in, 2 out]
            n556 = call "Elapsed Time37"("Time Target (s)"=w1190) -> ("Elapsed Time (s)"=w1189:dbl)  [unwired: 11 in, 7 out]
          }
          frame 5 {
            n557 = property on="Current Task time" class="Slide (strict)"("Scale.Maximum"=w1192) -> ()  [unwired: 2 in, 2 out]
            n558 = call "Elapsed Time38"("Time Target (s)"=w1192) -> ("Elapsed Time (s)"=w1191:dbl)  [unwired: 11 in, 7 out]
          }
          frame 6 {
            n559 = property on="Current Task time" class="Slide (strict)"("Scale.Maximum"=w1194) -> ()  [unwired: 2 in, 2 out]
            n560 = call "Elapsed Time39"("Time Target (s)"=w1194) -> ("Elapsed Time (s)"=w1193:dbl)  [unwired: 11 in, 7 out]
          }
          frame 7 {
            n561 = property on="Current Task time" class="Slide (strict)"("Scale.Maximum"=w1196) -> ()  [unwired: 2 in, 2 out]
            n562 = call "Elapsed Time40"("Time Target (s)"=w1196) -> ("Elapsed Time (s)"=w1195:dbl)  [unwired: 11 in, 7 out]
          }
          frame 8 {
            n563 = property on="Current Task time" class="Slide (strict)"("Scale.Maximum"=w1198) -> ()  [unwired: 2 in, 2 out]
            n564 = call "Elapsed Time41"("Time Target (s)"=w1198) -> ("Elapsed Time (s)"=w1197:dbl)  [unwired: 11 in, 7 out]
          }
          frame 9 {
            n565 = property on="Current Task time" class="Slide (strict)"("Scale.Maximum"=w1200) -> ()  [unwired: 2 in, 2 out]
            n566 = call "Elapsed Time42"("Time Target (s)"=w1200) -> ("Elapsed Time (s)"=w1199:dbl)  [unwired: 11 in, 7 out]
          }
          frame 10 {
            n567 = property on="Current Task time" class="Slide (strict)"("Scale.Maximum"=w1202) -> ()  [unwired: 2 in, 2 out]
            n568 = call "Elapsed Time43"("Time Target (s)"=w1202) -> ("Elapsed Time (s)"=w1201:dbl)  [unwired: 11 in, 7 out]
          }
          frame 11 {
            n569 = property on="Current Task time" class="Slide (strict)"("Scale.Maximum"=w1204) -> ()  [unwired: 2 in, 2 out]
            n570 = call "Elapsed Time44"("Time Target (s)"=w1204) -> ("Elapsed Time (s)"=w1203:dbl)  [unwired: 11 in, 7 out]
          }
          frame 12 {
            n571 = property on="Current Task time" class="Slide (strict)"("Scale.Maximum"=w1206) -> ()  [unwired: 2 in, 2 out]
            n572 = call "Elapsed Time45"("Time Target (s)"=w1206) -> ("Elapsed Time (s)"=w1205:dbl)  [unwired: 11 in, 7 out]
          }
          frame 13 {
            n573 = property on="Current Task time" class="Slide (strict)"("Scale.Maximum"=w1208) -> ()  [unwired: 2 in, 2 out]
            n574 = call "Elapsed Time122"("Time Target (s)"=w1208) -> ("Elapsed Time (s)"=w1207:dbl)  [unwired: 11 in, 7 out]
          }
          frame 0, Default {
            n575 = property on="Current Task time" class="Slide (strict)"("Scale.Maximum"=w1210) -> ()  [unwired: 2 in, 2 out]
            n576 = call "Elapsed Time123"("Time Target (s)"=w1210) -> ("Elapsed Time (s)"=w1209:dbl)  [unwired: 11 in, 7 out]
          }
        }
      }
      frame 8 {
        w1264 = 415.0  # Routine Time
        # "Routine 5: Lying on bed turned"
        n577 = property on="Total Routine Time" class="Slide (strict)"("Scale.Maximum"=w1264) -> ()  [unwired: 2 in, 2 out]
        n578 = call "Elapsed Time2"("Time Target (s)"=w1264, "Auto Reset"=FALSE ("Timer Reset")) -> ("Get Start Time (s)"=w1262:dbl, "Elapsed Time (s)"=w1258:dbl, "Time has Elapsed"=w1265:bool)  [unwired: 10 in, 5 out]
        "#5" <- w1265
        n579 = Seconds To Date/Time(time stamp (now)=w1262) -> (date time rec=w1263:T2)  [unwired: 1 in]
        n580 = Not(x=w1265) -> (.not. x?=w1268:bool)
        n581 = script code="t = [0,4,10,14,20,80,84,90,94,100,104,110,114,120,124,130,134,140,140.75,141.5,...\n    142.25,143,143.75,144.5,145.25,146,146.75,147.5,148.25,149,149.75,150.5,151.25,...\n    152,152.75,153,154.25,155,155.75,156.5,157.25,158,158.75,159.5,160.25,161,...\n    161.75,162.5,163.25,164,164.75,165.5,166.25,167,167.75,168.5,169.25,170,...\n    200,203.75,207.5,211.25,215,218.75,222.5,226.25,230,260,280,300,320,340,...\n    344,359,363,378,381,396,399,415];\n\nevent = [1,2,1,2,0,1,2,1,2,1,2,1,2,1,2,1,2,3,4,3,...\n        4,3,4,3,4,3,4,3,4,3,4,3,4,...\n        3,4,3,4,3,4,3,4,3,4,3,4,3,...\n        4,3,4,3,4,3,4,3,4,3,4,0,...\n        5,6,5,6,5,6,5,6,0,7,0,7,0,8,...\n        0,8,0,9,0,9,0,14];\n\nfor i = 2:length(t)\n    if ((x>=t(i-1)) &&  (x<t(i)))\n        y = event(i-1);\n        yNext = event(i);\n        dt = t(i) - t(i-1);\n        break;\n    end\nend"("x"=w1258) -> ("y"=w1259:dbl, "dt"=w1260:dbl, "yNext"=w1261:dbl)  [unwired: 1 in, 1 out]
        n582 = case shown="False" w1268 {
          tunnel: [w1325 w1337] -> w1267
          frame False {
            n583 = flat-sequence {
              tunnel: [w1333] -> w1325
              frame #0 {
                n584 = local write "Buffer"(FALSE ("Buffer")) -> ()
                n585 = local write "Play/Stop"(FALSE ("PlayInstruction")) -> ()
              }
              frame #1 {
                n586 = local write "Output"(0 ("Output")) -> ()
                n587 = local write "Save"(TRUE ("Save")) -> ()
              }
              frame #2 {
                n588 = Wait (ms)(milliseconds to wait=u32 500) -> ()  [unwired: 1 out]
              }
              frame #3 {
                n589 = local write "Flush"(TRUE ("Flush")) -> ()
              }
              frame #4 {
                w1332 = u16 0 items=["No sound", "Demo deep breathing", "Demo fast shallow breathing", "Demo slow shallow breathing", "Demo breath hold", "Demo cough/ laugh", "Demo abdomen movement", "Calibration", "Routine 1", "Routine 3", "Routine 4/5/7", "Calm music"] ("Play sound")
                w1333 = T4."Default"
                n590 = local write "Flush"(FALSE ("Flush")) -> ()
                n591 = local write "Save"(FALSE ("Save")) -> ()
                n592 = local write "Protocol"(w1333) -> ()
                n593 = local write "Play sound"(w1332) -> ()
              }
            }
          }
          frame True {
            w1336 = u16 10 items=["No sound", "Demo deep breathing", "Demo fast shallow breathing", "Demo slow shallow breathing", "Demo breath hold", "Demo cough/ laugh", "Demo abdomen movement", "Calibration", "Routine 1", "Routine 3", "Routine 4/5/7", "Calm music"] ("Play sound")
            n594 = local write "Play sound"(w1336) -> ()
            n595 = flat-sequence {
              tunnel: [T4."Routine 5"] -> w1337
              frame #0 {
                n596 = local write "Output"(1 ("Open")) -> ()
                n597 = local write "Play/Stop"(TRUE ("PlayInstruction")) -> ()
              }
              frame #1 {
                n598 = local write "Buffer"(TRUE ("Buffer")) -> ()
              }
              frame #2 {
              }
            }
          }
        }
        n599 = case shown="0, Default" w1259 {
          tunnel: ["\nPerform normal breathing, NO deep breathing or breath hold." "Inhale a slow deep breath." "\nExhale slowly." "Quick inhale.\n\n\n\nIf you cannot sustain for long, resume normal breathing." "\nQuick exhale.\n\n\nIf you cannot sustain for long, resume normal breathing." "Slow shallow inhale.\n\n\n\nIf you cannot sustain for long, resume normal breathing." "\nSlow exhale.\n\n\nIf you cannot sustain for long, resume normal breathing." "Exhale the current breath  and HOLD.\n\n\nIf you cannot sustain for long, resume normal breathing." "Perform voluntary coughing \n" "Perform voluntary laugh\n\n" "Read aloud the following text in between the lines:\n-----------------------------------------------------------------------\nFour score and seven years ago our fathers brought forth on this continent, a new nation, conceived in Liberty, and dedicated to the proposition that all men are created equal… That this nation, under God, shall have a new birth of freedom-and that government of the people, by the people, for the people, shall not perish from the earth.\n\n-----------------------------------------------------------------------\nWhen finished, take a deep breath and open mouth say \"Ah\" (like doctor checking your throat).\nPerform normal breathing until next instruction." "Exhale current breath and HOLD. Push abdomen inwards." "Relax abdomen back to normal and keep holding breath."] -> w1257
          frame 0, Default {
          }
          frame 1 {
          }
          frame 2 {
          }
          frame 3 {
          }
          frame 4 {
          }
          frame 5 {
          }
          frame 6 {
          }
          frame 7 {
          }
          frame 8 {
          }
          frame 9 {
          }
          frame 10 {
          }
          frame 12 {
          }
          frame 13 {
          }
        }
        n600 = case shown="14" w1261 {
          tunnel: ["\nPerform normal breathing, NO deep breathing or breath hold." "Inhale a slow deep breath." "\nExhale slowly." "Quick inhale.\n\n\n\nIf you cannot sustain for long, resume normal breathing." "\nQuick exhale.\n\n\nIf you cannot sustain for long, resume normal breathing." "Slow shallow inhale.\n\n\n\nIf you cannot sustain for long, resume normal breathing." "\nSlow exhale.\n\n\nIf you cannot sustain for long, resume normal breathing." "Exhale the current breath  and HOLD.\n\n\nIf you cannot sustain for long, resume normal breathing." "Perform voluntary coughing \n" "Perform voluntary laugh\n\n" "Read aloud the following text in between the lines:\n-----------------------------------------------------------------------\nFour score and ...\n-----------------------------------------------------------------------\nWhen finished, take a deep breath and open mouth say \"Ah\" (like doctor checking your throat).\nPerform normal breathing until next instruction." "Exhale current breath and HOLD. Push abdomen inwards." "Relax abdomen back to normal and keep holding breath." "Study Completed!"] -> w1255
          frame 0, Default {
          }
          frame 1 {
          }
          frame 2 {
          }
          frame 3 {
          }
          frame 4 {
          }
          frame 5 {
          }
          frame 6 {
          }
          frame 7 {
          }
          frame 8 {
          }
          frame 9 {
          }
          frame 10 {
          }
          frame 12 {
          }
          frame 13 {
          }
          frame 14 {
          }
        }
        n601 = case shown="0, Default" w1259 {
          tunnel: w1260 -> [w1271 w1273 w1275 w1277 w1279 w1281 w1283 w1285 w1287 w1289 w1291 w1293 w1295 w1297]
          tunnel: [w1270 w1272 w1274 w1276 w1278 w1280 w1282 w1284 w1286 w1288 w1290 w1292 w1294 w1296] -> w1256
          frame 1 {
            n602 = property on="Current Task time" class="Slide (strict)"("Scale.Maximum"=w1271) -> ()  [unwired: 2 in, 2 out]
            n603 = call "Elapsed Time46"("Time Target (s)"=w1271) -> ("Elapsed Time (s)"=w1270:dbl)  [unwired: 11 in, 7 out]
          }
          frame 2 {
            n604 = property on="Current Task time" class="Slide (strict)"("Scale.Maximum"=w1273) -> ()  [unwired: 2 in, 2 out]
            n605 = call "Elapsed Time47"("Time Target (s)"=w1273) -> ("Elapsed Time (s)"=w1272:dbl)  [unwired: 11 in, 7 out]
          }
          frame 3 {
            n606 = property on="Current Task time" class="Slide (strict)"("Scale.Maximum"=w1275) -> ()  [unwired: 2 in, 2 out]
            n607 = call "Elapsed Time48"("Time Target (s)"=w1275) -> ("Elapsed Time (s)"=w1274:dbl)  [unwired: 11 in, 7 out]
          }
          frame 4 {
            n608 = property on="Current Task time" class="Slide (strict)"("Scale.Maximum"=w1277) -> ()  [unwired: 2 in, 2 out]
            n609 = call "Elapsed Time49"("Time Target (s)"=w1277) -> ("Elapsed Time (s)"=w1276:dbl)  [unwired: 11 in, 7 out]
          }
          frame 5 {
            n610 = property on="Current Task time" class="Slide (strict)"("Scale.Maximum"=w1279) -> ()  [unwired: 2 in, 2 out]
            n611 = call "Elapsed Time50"("Time Target (s)"=w1279) -> ("Elapsed Time (s)"=w1278:dbl)  [unwired: 11 in, 7 out]
          }
          frame 6 {
            n612 = property on="Current Task time" class="Slide (strict)"("Scale.Maximum"=w1281) -> ()  [unwired: 2 in, 2 out]
            n613 = call "Elapsed Time51"("Time Target (s)"=w1281) -> ("Elapsed Time (s)"=w1280:dbl)  [unwired: 11 in, 7 out]
          }
          frame 7 {
            n614 = property on="Current Task time" class="Slide (strict)"("Scale.Maximum"=w1283) -> ()  [unwired: 2 in, 2 out]
            n615 = call "Elapsed Time52"("Time Target (s)"=w1283) -> ("Elapsed Time (s)"=w1282:dbl)  [unwired: 11 in, 7 out]
          }
          frame 8 {
            n616 = property on="Current Task time" class="Slide (strict)"("Scale.Maximum"=w1285) -> ()  [unwired: 2 in, 2 out]
            n617 = call "Elapsed Time53"("Time Target (s)"=w1285) -> ("Elapsed Time (s)"=w1284:dbl)  [unwired: 11 in, 7 out]
          }
          frame 9 {
            n618 = property on="Current Task time" class="Slide (strict)"("Scale.Maximum"=w1287) -> ()  [unwired: 2 in, 2 out]
            n619 = call "Elapsed Time54"("Time Target (s)"=w1287) -> ("Elapsed Time (s)"=w1286:dbl)  [unwired: 11 in, 7 out]
          }
          frame 10 {
            n620 = property on="Current Task time" class="Slide (strict)"("Scale.Maximum"=w1289) -> ()  [unwired: 2 in, 2 out]
            n621 = call "Elapsed Time55"("Time Target (s)"=w1289) -> ("Elapsed Time (s)"=w1288:dbl)  [unwired: 11 in, 7 out]
          }
          frame 11 {
            n622 = property on="Current Task time" class="Slide (strict)"("Scale.Maximum"=w1291) -> ()  [unwired: 2 in, 2 out]
            n623 = call "Elapsed Time56"("Time Target (s)"=w1291) -> ("Elapsed Time (s)"=w1290:dbl)  [unwired: 11 in, 7 out]
          }
          frame 12 {
            n624 = property on="Current Task time" class="Slide (strict)"("Scale.Maximum"=w1293) -> ()  [unwired: 2 in, 2 out]
            n625 = call "Elapsed Time57"("Time Target (s)"=w1293) -> ("Elapsed Time (s)"=w1292:dbl)  [unwired: 11 in, 7 out]
          }
          frame 13 {
            n626 = property on="Current Task time" class="Slide (strict)"("Scale.Maximum"=w1295) -> ()  [unwired: 2 in, 2 out]
            n627 = call "Elapsed Time124"("Time Target (s)"=w1295) -> ("Elapsed Time (s)"=w1294:dbl)  [unwired: 11 in, 7 out]
          }
          frame 0, Default {
            n628 = property on="Current Task time" class="Slide (strict)"("Scale.Maximum"=w1297) -> ()  [unwired: 2 in, 2 out]
            n629 = call "Elapsed Time125"("Time Target (s)"=w1297) -> ("Elapsed Time (s)"=w1296:dbl)  [unwired: 11 in, 7 out]
          }
        }
      }
      frame 9 {
        w1343 = 180.0  # Routine Time
        # "Routine 6 Voice recognition"
        n630 = property on="Current Task time" class="Slide (strict)"("Scale.Maximum"=w1343) -> ()  [unwired: 2 in, 2 out]
        n631 = property on="Total Routine Time" class="Slide (strict)"("Scale.Maximum"=w1343) -> ()  [unwired: 2 in, 2 out]
        n632 = call "Elapsed Time6"("Time Target (s)"=w1343, "Auto Reset"=FALSE ("Timer Reset")) -> ("Get Start Time (s)"=w1346:dbl, "Elapsed Time (s)"=w1344:dbl, "Time has Elapsed"=w1348:bool)  [unwired: 10 in, 5 out]
        "#6" <- w1348
        n633 = Seconds To Date/Time(time stamp (now)=w1346) -> (date time rec=w1347:T2)  [unwired: 1 in]
        n634 = Not(x=w1348) -> (.not. x?=w1351:bool)
        n635 = case shown="True" w1351 {
          tunnel: [w1353 w1362] -> w1350
          frame False {
            n636 = flat-sequence {
              tunnel: [w1359] -> w1353
              frame #0 {
                n637 = local write "Buffer"(FALSE ("Buffer")) -> ()
              }
              frame #1 {
                n638 = local write "Output"(0 ("Output")) -> ()
                n639 = local write "Save"(TRUE ("Save")) -> ()
              }
              frame #2 {
                n640 = Wait (ms)(milliseconds to wait=u32 500) -> ()  [unwired: 1 out]
              }
              frame #3 {
                n641 = local write "Flush"(TRUE ("Flush")) -> ()
              }
              frame #4 {
                w1359 = T4."Default"
                n642 = local write "Flush"(FALSE ("Flush")) -> ()
                n643 = local write "Save"(FALSE ("Save")) -> ()
                n644 = local write "Protocol"(w1359) -> ()
              }
            }
          }
          frame True {
            n645 = flat-sequence {
              tunnel: [T4."Routine 6"] -> w1362
              frame #0 {
                n646 = local write "Output"(1 ("Open")) -> ()
              }
              frame #1 {
                n647 = local write "Buffer"(TRUE ("Buffer")) -> ()
              }
              frame #2 {
              }
            }
          }
        }
      }
      frame 10 {
        w1376 = 415.0  # Routine Time
        # "Routine 7: In car seat"
        n648 = property on="Total Routine Time" class="Slide (strict)"("Scale.Maximum"=w1376) -> ()  [unwired: 2 in, 2 out]
        n649 = call "Elapsed Time8"("Time Target (s)"=w1376, "Reset"=FALSE) -> ("Get Start Time (s)"=w1374:dbl, "Elapsed Time (s)"=w1368:dbl, "Time has Elapsed"=w1377:bool)  [unwired: 10 in, 5 out]
        "#7" <- w1377
        n650 = Seconds To Date/Time(time stamp (now)=w1374) -> (date time rec=w1375:T2)  [unwired: 1 in]
        n651 = Not(x=w1377) -> (.not. x?=w1380:bool)
        n652 = script code="t = [0,4,10,14,20,80,84,90,94,100,104,110,114,120,124,130,134,140,140.75,141.5,...\n    142.25,143,143.75,144.5,145.25,146,146.75,147.5,148.25,149,149.75,150.5,151.25,...\n    152,152.75,153,154.25,155,155.75,156.5,157.25,158,158.75,159.5,160.25,161,...\n    161.75,162.5,163.25,164,164.75,165.5,166.25,167,167.75,168.5,169.25,170,...\n    200,203.75,207.5,211.25,215,218.75,222.5,226.25,230,260,280,300,320,340,...\n    344,359,363,378,381,396,399,415];\n\nevent = [1,2,1,2,0,1,2,1,2,1,2,1,2,1,2,1,2,3,4,3,...\n        4,3,4,3,4,3,4,3,4,3,4,3,4,...\n        3,4,3,4,3,4,3,4,3,4,3,4,3,...\n        4,3,4,3,4,3,4,3,4,3,4,0,...\n        5,6,5,6,5,6,5,6,0,7,0,7,0,8,...\n        0,8,0,9,0,9,0,14];\n\nfor i = 2:length(t)\n    if ((x>=t(i-1)) &&  (x<t(i)))\n        y = event(i-1);\n        yNext = event(i);\n        dt = t(i) - t(i-1);\n        break;\n    end\nend"("x"=w1368) -> ("y"=w1371:dbl, "dt"=w1372:dbl, "yNext"=w1373:dbl)  [unwired: 1 in, 1 out]
        n653 = case shown="True" w1380 {
          tunnel: [w1436 w1448] -> w1379
          frame False {
            n654 = flat-sequence {
              tunnel: [w1444] -> w1436
              frame #0 {
                n655 = local write "Buffer"(FALSE ("Buffer")) -> ()
                n656 = local write "Play/Stop"(FALSE ("PlayInstr")) -> ()
              }
              frame #1 {
                n657 = local write "Output"(0 ("Output")) -> ()
                n658 = local write "Save"(TRUE ("Save")) -> ()
              }
              frame #2 {
                n659 = Wait (ms)(milliseconds to wait=u32 500) -> ()  [unwired: 1 out]
              }
              frame #3 {
                n660 = local write "Flush"(TRUE ("Flush")) -> ()
              }
              frame #4 {
                w1443 = u16 0 items=["No sound", "Demo deep breathing", "Demo fast shallow breathing", "Demo slow shallow breathing", "Demo breath hold", "Demo cough/ laugh", "Demo abdomen movement", "Calibration", "Routine 1", "Routine 3", "Routine 4/5/7", "Calm music"] ("Play sound")
                w1444 = T4."Default"
                n661 = local write "Flush"(FALSE ("Flush")) -> ()
                n662 = local write "Save"(FALSE ("Save")) -> ()
                n663 = local write "Play sound"(w1443) -> ()
                n664 = local write "Protocol"(w1444) -> ()
              }
            }
          }
          frame True {
            w1447 = u16 10 items=["No sound", "Demo deep breathing", "Demo fast shallow breathing", "Demo slow shallow breathing", "Demo breath hold", "Demo cough/ laugh", "Demo abdomen movement", "Calibration", "Routine 1", "Routine 3", "Routine 4/5/7", "Calm music"] ("Play sound")
            n665 = local write "Play sound"(w1447) -> ()
            n666 = flat-sequence {
              tunnel: [w1452] -> w1448
              frame #0 {
                n667 = local write "Output"(1 ("Open")) -> ()
                n668 = local write "Play/Stop"(TRUE ("PlayInstr")) -> ()
              }
              frame #1 {
                n669 = local write "Buffer"(TRUE ("Buffer")) -> ()
              }
              frame #2 {
                n670 = local read "Protocol"() -> (w1452:u16)
              }
            }
          }
        }
        n671 = case shown="0, Default" w1371 {
          tunnel: ["\nPerform normal breathing, NO deep breathing or breath hold." "Inhale a slow deep breath." "\nExhale slowly." "Quick inhale.\n\n\n\nIf you cannot sustain for long, resume normal breathing." "\nQuick exhale.\n\n\nIf you cannot sustain for long, resume normal breathing." "Slow shallow inhale.\n\n\n\nIf you cannot sustain for long, resume normal breathing." "\nSlow exhale.\n\n\nIf you cannot sustain for long, resume normal breathing." "Exhale the current breath  and HOLD.\n\n\nIf you cannot sustain for long, resume normal breathing." "Perform voluntary coughing \n" "Perform voluntary laugh\n\n" "Read aloud the following text in between the lines:\n-----------------------------------------------------------------------\nFour score and seven years ago our fathers brought forth on this continent, a new nation, conceived in Liberty, and dedicated to the proposition that all men are created equal… That this nation, under God, shall have a new birth of freedom-and that government of the people, by the people, for the people, shall not perish from the earth.\n\n-----------------------------------------------------------------------\nWhen finished, take a deep breath and open mouth say \"Ah\" (like doctor checking your throat).\nPerform normal breathing until next instruction." "Exhale current breath and HOLD. Push abdomen inwards." "Relax abdomen back to normal and keep holding breath."] -> w1369
          frame 0, Default {
          }
          frame 1 {
          }
          frame 2 {
          }
          frame 3 {
          }
          frame 4 {
          }
          frame 5 {
          }
          frame 6 {
          }
          frame 7 {
          }
          frame 8 {
          }
          frame 9 {
          }
          frame 10 {
          }
          frame 12 {
          }
          frame 13 {
          }
        }
        n672 = case shown="14" w1373 {
          tunnel: ["\nPerform normal breathing, NO deep breathing or breath hold." "Inhale a slow deep breath." "\nExhale slowly." "Quick inhale.\n\n\n\nIf you cannot sustain for long, resume normal breathing." "\nQuick exhale.\n\n\nIf you cannot sustain for long, resume normal breathing." "Slow shallow inhale.\n\n\n\nIf you cannot sustain for long, resume normal breathing." "\nSlow exhale.\n\n\nIf you cannot sustain for long, resume normal breathing." "Exhale the current breath  and HOLD.\n\n\nIf you cannot sustain for long, resume normal breathing." "Perform voluntary coughing \n" "Perform voluntary laugh\n\n" "Read aloud the following text in between the lines:\n-----------------------------------------------------------------------\nFour score and ...\n-----------------------------------------------------------------------\nWhen finished, take a deep breath and open mouth say \"Ah\" (like doctor checking your throat).\nPerform normal breathing until next instruction." "Exhale current breath and HOLD. Push abdomen inwards." "Relax abdomen back to normal and keep holding breath." "Study Completed!"] -> w1367
          frame 0, Default {
          }
          frame 1 {
          }
          frame 2 {
          }
          frame 3 {
          }
          frame 4 {
          }
          frame 5 {
          }
          frame 6 {
          }
          frame 7 {
          }
          frame 8 {
          }
          frame 9 {
          }
          frame 10 {
          }
          frame 12 {
          }
          frame 13 {
          }
          frame 14 {
          }
        }
        n673 = case shown="0, Default" w1371 {
          tunnel: w1372 -> [w1382 w1384 w1386 w1388 w1390 w1392 w1394 w1396 w1398 w1400 w1402 w1404 w1406 w1408]
          tunnel: [w1381 w1383 w1385 w1387 w1389 w1391 w1393 w1395 w1397 w1399 w1401 w1403 w1405 w1407] -> w1370
          frame 1 {
            n674 = property on="Current Task time" class="Slide (strict)"("Scale.Maximum"=w1382) -> ()  [unwired: 2 in, 2 out]
            n675 = call "Elapsed Time58"("Time Target (s)"=w1382) -> ("Elapsed Time (s)"=w1381:dbl)  [unwired: 11 in, 7 out]
          }
          frame 2 {
            n676 = property on="Current Task time" class="Slide (strict)"("Scale.Maximum"=w1384) -> ()  [unwired: 2 in, 2 out]
            n677 = call "Elapsed Time59"("Time Target (s)"=w1384) -> ("Elapsed Time (s)"=w1383:dbl)  [unwired: 11 in, 7 out]
          }
          frame 3 {
            n678 = property on="Current Task time" class="Slide (strict)"("Scale.Maximum"=w1386) -> ()  [unwired: 2 in, 2 out]
            n679 = call "Elapsed Time60"("Time Target (s)"=w1386) -> ("Elapsed Time (s)"=w1385:dbl)  [unwired: 11 in, 7 out]
          }
          frame 4 {
            n680 = property on="Current Task time" class="Slide (strict)"("Scale.Maximum"=w1388) -> ()  [unwired: 2 in, 2 out]
            n681 = call "Elapsed Time61"("Time Target (s)"=w1388) -> ("Elapsed Time (s)"=w1387:dbl)  [unwired: 11 in, 7 out]
          }
          frame 5 {
            n682 = property on="Current Task time" class="Slide (strict)"("Scale.Maximum"=w1390) -> ()  [unwired: 2 in, 2 out]
            n683 = call "Elapsed Time62"("Time Target (s)"=w1390) -> ("Elapsed Time (s)"=w1389:dbl)  [unwired: 11 in, 7 out]
          }
          frame 6 {
            n684 = property on="Current Task time" class="Slide (strict)"("Scale.Maximum"=w1392) -> ()  [unwired: 2 in, 2 out]
            n685 = call "Elapsed Time63"("Time Target (s)"=w1392) -> ("Elapsed Time (s)"=w1391:dbl)  [unwired: 11 in, 7 out]
          }
          frame 7 {
            n686 = property on="Current Task time" class="Slide (strict)"("Scale.Maximum"=w1394) -> ()  [unwired: 2 in, 2 out]
            n687 = call "Elapsed Time64"("Time Target (s)"=w1394) -> ("Elapsed Time (s)"=w1393:dbl)  [unwired: 11 in, 7 out]
          }
          frame 8 {
            n688 = property on="Current Task time" class="Slide (strict)"("Scale.Maximum"=w1396) -> ()  [unwired: 2 in, 2 out]
            n689 = call "Elapsed Time65"("Time Target (s)"=w1396) -> ("Elapsed Time (s)"=w1395:dbl)  [unwired: 11 in, 7 out]
          }
          frame 9 {
            n690 = property on="Current Task time" class="Slide (strict)"("Scale.Maximum"=w1398) -> ()  [unwired: 2 in, 2 out]
            n691 = call "Elapsed Time66"("Time Target (s)"=w1398) -> ("Elapsed Time (s)"=w1397:dbl)  [unwired: 11 in, 7 out]
          }
          frame 10 {
            n692 = property on="Current Task time" class="Slide (strict)"("Scale.Maximum"=w1400) -> ()  [unwired: 2 in, 2 out]
            n693 = call "Elapsed Time67"("Time Target (s)"=w1400) -> ("Elapsed Time (s)"=w1399:dbl)  [unwired: 11 in, 7 out]
          }
          frame 11 {
            n694 = property on="Current Task time" class="Slide (strict)"("Scale.Maximum"=w1402) -> ()  [unwired: 2 in, 2 out]
            n695 = call "Elapsed Time68"("Time Target (s)"=w1402) -> ("Elapsed Time (s)"=w1401:dbl)  [unwired: 11 in, 7 out]
          }
          frame 12 {
            n696 = property on="Current Task time" class="Slide (strict)"("Scale.Maximum"=w1404) -> ()  [unwired: 2 in, 2 out]
            n697 = call "Elapsed Time69"("Time Target (s)"=w1404) -> ("Elapsed Time (s)"=w1403:dbl)  [unwired: 11 in, 7 out]
          }
          frame 13 {
            n698 = property on="Current Task time" class="Slide (strict)"("Scale.Maximum"=w1406) -> ()  [unwired: 2 in, 2 out]
            n699 = call "Elapsed Time126"("Time Target (s)"=w1406) -> ("Elapsed Time (s)"=w1405:dbl)  [unwired: 11 in, 7 out]
          }
          frame 0, Default {
            n700 = property on="Current Task time" class="Slide (strict)"("Scale.Maximum"=w1408) -> ()  [unwired: 2 in, 2 out]
            n701 = call "Elapsed Time127"("Time Target (s)"=w1408) -> ("Elapsed Time (s)"=w1407:dbl)  [unwired: 11 in, 7 out]
          }
        }
      }
      frame 11 {
        w1462 = 51.0  # Routine Time
        # "Calibration Routine 1"
        n702 = property on="Total Routine Time" class="Slide (strict)"("Scale.Maximum"=w1462) -> ()  [unwired: 2 in, 2 out]
        n703 = call "Elapsed Time71"("Time Target (s)"=w1462, "Auto Reset"=FALSE ("Timer Reset")) -> ("Get Start Time (s)"=w1460:dbl, "Elapsed Time (s)"=w1456:dbl, "Time has Elapsed"=w1463:bool)  [unwired: 10 in, 5 out]
        "Calib 1" <- w1463
        n704 = Seconds To Date/Time(time stamp (now)=w1460) -> (date time rec=w1461:T2)  [unwired: 1 in]
        n705 = Not(x=w1463) -> (.not. x?=w1466:bool)
        n706 = script code="t = [0,15,18,22.5,25.5,30,33,37.5,40.5,45,45.75,46.5,47.25,48,48.75,49.5,50.25,51];\n\nevent = [0,1,2,1,2,1,2,1,2,3,4,3,4,3,4,3,4,3,4,14];\n\nfor i = 2:length(t)\n    if ((x>=t(i-1)) &&  (x<t(i)))\n        y = event(i-1);\n        yNext = event(i);\n        dt = t(i) - t(i-1);\n        break;\n    end\nend"("x"=w1456) -> ("y"=w1457:dbl, "dt"=w1458:dbl, "yNext"=w1459:dbl)  [unwired: 1 in, 1 out]
        n707 = case shown="True" w1466 {
          tunnel: [w1505 w1517] -> w1465
          frame False {
            n708 = flat-sequence {
              tunnel: [w1513] -> w1505
              frame #0 {
                n709 = local write "Buffer"(FALSE ("Buffer")) -> ()
                n710 = local write "Play/Stop"(FALSE ("Play\nCalibration")) -> ()
              }
              frame #1 {
                n711 = local write "Output"(0 ("Output")) -> ()
                n712 = local write "Save"(TRUE ("Save")) -> ()
              }
              frame #2 {
                n713 = Wait (ms)(milliseconds to wait=u32 500) -> ()  [unwired: 1 out]
              }
              frame #3 {
                n714 = local write "Flush"(TRUE ("Flush")) -> ()
              }
              frame #4 {
                w1512 = u16 0 items=["No sound", "Demo deep breathing", "Demo fast shallow breathing", "Demo slow shallow breathing", "Demo breath hold", "Demo cough/ laugh", "Demo abdomen movement", "Calibration", "Routine 1", "Routine 3", "Routine 4/5/7", "Calm music"] ("Play sound")
                w1513 = T4."Default"
                n715 = local write "Flush"(FALSE ("Flush")) -> ()
                n716 = local write "Save"(FALSE ("Save")) -> ()
                n717 = local write "Protocol"(w1513) -> ()
                n718 = local write "Play sound"(w1512) -> ()
              }
            }
          }
          frame True {
            w1516 = u16 7 items=["No sound", "Demo deep breathing", "Demo fast shallow breathing", "Demo slow shallow breathing", "Demo breath hold", "Demo cough/ laugh", "Demo abdomen movement", "Calibration", "Routine 1", "Routine 3", "Routine 4/5/7", "Calm music"] ("Play sound")
            n719 = local write "Play sound"(w1516) -> ()
            n720 = flat-sequence {
              tunnel: [T4."Calib1"] -> w1517
              frame #0 {
                n721 = local write "Play/Stop"(TRUE ("Play\nCalibration")) -> ()
                n722 = local write "Output"(1 ("Open")) -> ()
              }
              frame #1 {
                n723 = local write "Buffer"(TRUE ("Buffer")) -> ()
              }
              frame #2 {
              }
            }
          }
        }
        n724 = case shown="0, Default" w1457 {
          tunnel: ["\nPerform normal breathing, NO deep breathing or breath hold." "Inhale a slow deep breath." "\nExhale slowly." "Quick inhale.\n\n\n\nIf you cannot sustain for long, resume normal breathing." "\nQuick exhale.\n\n\nIf you cannot sustain for long, resume normal breathing." "Slow shallow inhale.\n\n\n\nIf you cannot sustain for long, resume normal breathing." "\nSlow exhale.\n\n\nIf you cannot sustain for long, resume normal breathing." "Exhale the current breath  and HOLD.\n\n\nIf you cannot sustain for long, resume normal breathing." "Perform voluntary coughing \n" "Perform voluntary laugh\n\n" "Read aloud the following text in between the lines:\n-----------------------------------------------------------------------\nFour score and seven years ago our fathers brought forth on this continent, a new nation, conceived in Liberty, and dedicated to the proposition that all men are created equal… That this nation, under God, shall have a new birth of freedom-and that government of the people, by the people, for the people, shall not perish from the earth.\n\n-----------------------------------------------------------------------\nWhen finished, take a deep breath and open mouth say \"Ah\" (like doctor checking your throat).\nPerform normal breathing until next instruction." "Exhale current breath and HOLD. Push abdomen inwards." "Relax abdomen back to normal and keep holding breath."] -> w1455
          frame 0, Default {
          }
          frame 1 {
          }
          frame 2 {
          }
          frame 3 {
          }
          frame 4 {
          }
          frame 5 {
          }
          frame 6 {
          }
          frame 7 {
          }
          frame 8 {
          }
          frame 9 {
          }
          frame 10 {
          }
          frame 12 {
          }
          frame 13 {
          }
        }
        n725 = case shown="0, Default" w1459 {
          tunnel: ["\nPerform normal breathing, NO deep breathing or breath hold." "Inhale a slow deep breath." "\nExhale slowly." "Quick inhale.\n\n\n\nIf you cannot sustain for long, resume normal breathing." "\nQuick exhale.\n\n\nIf you cannot sustain for long, resume normal breathing." "Slow shallow inhale.\n\n\n\nIf you cannot sustain for long, resume normal breathing." "\nSlow exhale.\n\n\nIf you cannot sustain for long, resume normal breathing." "Exhale the current breath  and HOLD.\n\n\nIf you cannot sustain for long, resume normal breathing." "Perform voluntary coughing \n" "Perform voluntary laugh\n\n" "Read aloud the following text in between the lines:\n-----------------------------------------------------------------------\nFour score and ...\n-----------------------------------------------------------------------\nWhen finished, take a deep breath and open mouth say \"Ah\" (like doctor checking your throat).\nPerform normal breathing until next instruction." "Exhale current breath and HOLD. Push abdomen inwards." "Relax abdomen back to normal and keep holding breath." "Study completed!"] -> w1453
          frame 0, Default {
          }
          frame 1 {
          }
          frame 2 {
          }
          frame 3 {
          }
          frame 4 {
          }
          frame 5 {
          }
          frame 6 {
          }
          frame 7 {
          }
          frame 8 {
          }
          frame 9 {
          }
          frame 10 {
          }
          frame 12 {
          }
          frame 13 {
          }
          frame 14 {
          }
        }
        n726 = case shown="0, Default" w1457 {
          tunnel: w1458 -> [w1469 w1471 w1473 w1475 w1477]
          tunnel: [w1468 w1470 w1472 w1474 w1476] -> w1454
          frame 1 {
            n727 = property on="Current Task time" class="Slide (strict)"("Scale.Maximum"=w1469) -> ()  [unwired: 2 in, 2 out]
            n728 = call "Elapsed Time72"("Time Target (s)"=w1469) -> ("Elapsed Time (s)"=w1468:dbl)  [unwired: 11 in, 7 out]
          }
          frame 2 {
            n729 = property on="Current Task time" class="Slide (strict)"("Scale.Maximum"=w1471) -> ()  [unwired: 2 in, 2 out]
            n730 = call "Elapsed Time73"("Time Target (s)"=w1471) -> ("Elapsed Time (s)"=w1470:dbl)  [unwired: 11 in, 7 out]
          }
          frame 3 {
            n731 = property on="Current Task time" class="Slide (strict)"("Scale.Maximum"=w1473) -> ()  [unwired: 2 in, 2 out]
            n732 = call "Elapsed Time74"("Time Target (s)"=w1473) -> ("Elapsed Time (s)"=w1472:dbl)  [unwired: 11 in, 7 out]
          }
          frame 4 {
            n733 = property on="Current Task time" class="Slide (strict)"("Scale.Maximum"=w1475) -> ()  [unwired: 2 in, 2 out]
            n734 = call "Elapsed Time75"("Time Target (s)"=w1475) -> ("Elapsed Time (s)"=w1474:dbl)  [unwired: 11 in, 7 out]
          }
          frame 0, Default {
            n735 = property on="Current Task time" class="Slide (strict)"("Scale.Maximum"=w1477) -> ()  [unwired: 2 in, 2 out]
            n736 = call "Elapsed Time134"("Time Target (s)"=w1477) -> ("Elapsed Time (s)"=w1476:dbl)  [unwired: 11 in, 7 out]
          }
        }
      }
      frame 12 {
        w1531 = 51.0  # Routine Time
        # "Calibration Routine 3"
        n737 = property on="Total Routine Time" class="Slide (strict)"("Scale.Maximum"=w1531) -> ()  [unwired: 2 in, 2 out]
        n738 = call "Elapsed Time76"("Time Target (s)"=w1531, "Auto Reset"=FALSE ("Timer Reset")) -> ("Get Start Time (s)"=w1529:dbl, "Elapsed Time (s)"=w1525:dbl, "Time has Elapsed"=w1532:bool)  [unwired: 10 in, 5 out]
        "Calib 3" <- w1532
        n739 = Seconds To Date/Time(time stamp (now)=w1529) -> (date time rec=w1530:T2)  [unwired: 1 in]
        n740 = Not(x=w1532) -> (.not. x?=w1535:bool)
        n741 = script code="t = [0,15,18,22.5,25.5,30,33,37.5,40.5,45,45.75,46.5,47.25,48,48.75,49.5,50.25,51];\n\nevent = [0,1,2,1,2,1,2,1,2,3,4,3,4,3,4,3,4,3,4,14];\n\nfor i = 2:length(t)\n    if ((x>=t(i-1)) &&  (x<t(i)))\n        y = event(i-1);\n        yNext = event(i);\n        dt = t(i) - t(i-1);\n        break;\n    end\nend"("x"=w1525) -> ("y"=w1526:dbl, "dt"=w1527:dbl, "yNext"=w1528:dbl)  [unwired: 1 in, 1 out]
        n742 = case shown="True" w1535 {
          tunnel: [w1574 w1586] -> w1534
          frame False {
            n743 = flat-sequence {
              tunnel: [w1582] -> w1574
              frame #0 {
                n744 = local write "Buffer"(FALSE ("Buffer")) -> ()
                n745 = local write "Play/Stop"(FALSE ("Play\nCalibration")) -> ()
              }
              frame #1 {
                n746 = local write "Output"(0 ("Output")) -> ()
                n747 = local write "Save"(TRUE ("Save")) -> ()
              }
              frame #2 {
                n748 = Wait (ms)(milliseconds to wait=u32 500) -> ()  [unwired: 1 out]
              }
              frame #3 {
                n749 = local write "Flush"(TRUE ("Flush")) -> ()
              }
              frame #4 {
                w1581 = u16 0 items=["No sound", "Demo deep breathing", "Demo fast shallow breathing", "Demo slow shallow breathing", "Demo breath hold", "Demo cough/ laugh", "Demo abdomen movement", "Calibration", "Routine 1", "Routine 3", "Routine 4/5/7", "Calm music"] ("Play sound")
                w1582 = T4."Default"
                n750 = local write "Flush"(FALSE ("Flush")) -> ()
                n751 = local write "Save"(FALSE ("Save")) -> ()
                n752 = local write "Protocol"(w1582) -> ()
                n753 = local write "Play sound"(w1581) -> ()
              }
            }
          }
          frame True {
            w1585 = u16 7 items=["No sound", "Demo deep breathing", "Demo fast shallow breathing", "Demo slow shallow breathing", "Demo breath hold", "Demo cough/ laugh", "Demo abdomen movement", "Calibration", "Routine 1", "Routine 3", "Routine 4/5/7", "Calm music"] ("Play sound")
            n754 = local write "Play sound"(w1585) -> ()
            n755 = flat-sequence {
              tunnel: [T4."Calib3"] -> w1586
              frame #0 {
                n756 = local write "Output"(1 ("Open")) -> ()
                n757 = local write "Play/Stop"(TRUE ("Play\nCalibration")) -> ()
              }
              frame #1 {
                n758 = local write "Buffer"(TRUE ("Buffer")) -> ()
              }
              frame #2 {
              }
            }
          }
        }
        n759 = case shown="0, Default" w1526 {
          tunnel: ["\nPerform normal breathing, NO deep breathing or breath hold." "Inhale a slow deep breath." "\nExhale slowly." "Quick inhale.\n\n\n\nIf you cannot sustain for long, resume normal breathing." "\nQuick exhale.\n\n\nIf you cannot sustain for long, resume normal breathing." "Slow shallow inhale.\n\n\n\nIf you cannot sustain for long, resume normal breathing." "\nSlow exhale.\n\n\nIf you cannot sustain for long, resume normal breathing." "Exhale the current breath  and HOLD.\n\n\nIf you cannot sustain for long, resume normal breathing." "Perform voluntary coughing \n" "Perform voluntary laugh\n\n" "Read aloud the following text in between the lines:\n-----------------------------------------------------------------------\nFour score and seven years ago our fathers brought forth on this continent, a new nation, conceived in Liberty, and dedicated to the proposition that all men are created equal… That this nation, under God, shall have a new birth of freedom-and that government of the people, by the people, for the people, shall not perish from the earth.\n\n-----------------------------------------------------------------------\nWhen finished, take a deep breath and open mouth say \"Ah\" (like doctor checking your throat).\nPerform normal breathing until next instruction." "Exhale current breath and HOLD. Push abdomen inwards." "Relax abdomen back to normal and keep holding breath."] -> w1524
          frame 0, Default {
          }
          frame 1 {
          }
          frame 2 {
          }
          frame 3 {
          }
          frame 4 {
          }
          frame 5 {
          }
          frame 6 {
          }
          frame 7 {
          }
          frame 8 {
          }
          frame 9 {
          }
          frame 10 {
          }
          frame 12 {
          }
          frame 13 {
          }
        }
        n760 = case shown="0, Default" w1528 {
          tunnel: ["\nPerform normal breathing, NO deep breathing or breath hold." "Inhale a slow deep breath." "\nExhale slowly." "Quick inhale.\n\n\n\nIf you cannot sustain for long, resume normal breathing." "\nQuick exhale.\n\n\nIf you cannot sustain for long, resume normal breathing." "Slow shallow inhale.\n\n\n\nIf you cannot sustain for long, resume normal breathing." "\nSlow exhale.\n\n\nIf you cannot sustain for long, resume normal breathing." "Exhale the current breath  and HOLD.\n\n\nIf you cannot sustain for long, resume normal breathing." "Perform voluntary coughing \n" "Perform voluntary laugh\n\n" "Read aloud the following text in between the lines:\n-----------------------------------------------------------------------\nFour score and ...\n-----------------------------------------------------------------------\nWhen finished, take a deep breath and open mouth say \"Ah\" (like doctor checking your throat).\nPerform normal breathing until next instruction." "Exhale current breath and HOLD. Push abdomen inwards." "Relax abdomen back to normal and keep holding breath." "Study completed!"] -> w1522
          frame 0, Default {
          }
          frame 1 {
          }
          frame 2 {
          }
          frame 3 {
          }
          frame 4 {
          }
          frame 5 {
          }
          frame 6 {
          }
          frame 7 {
          }
          frame 8 {
          }
          frame 9 {
          }
          frame 10 {
          }
          frame 12 {
          }
          frame 13 {
          }
          frame 14 {
          }
        }
        n761 = case shown="0, Default" w1526 {
          tunnel: w1527 -> [w1538 w1540 w1542 w1544 w1546]
          tunnel: [w1537 w1539 w1541 w1543 w1545] -> w1523
          frame 1 {
            n762 = property on="Current Task time" class="Slide (strict)"("Scale.Maximum"=w1538) -> ()  [unwired: 2 in, 2 out]
            n763 = call "Elapsed Time77"("Time Target (s)"=w1538) -> ("Elapsed Time (s)"=w1537:dbl)  [unwired: 11 in, 7 out]
          }
          frame 2 {
            n764 = property on="Current Task time" class="Slide (strict)"("Scale.Maximum"=w1540) -> ()  [unwired: 2 in, 2 out]
            n765 = call "Elapsed Time78"("Time Target (s)"=w1540) -> ("Elapsed Time (s)"=w1539:dbl)  [unwired: 11 in, 7 out]
          }
          frame 3 {
            n766 = property on="Current Task time" class="Slide (strict)"("Scale.Maximum"=w1542) -> ()  [unwired: 2 in, 2 out]
            n767 = call "Elapsed Time79"("Time Target (s)"=w1542) -> ("Elapsed Time (s)"=w1541:dbl)  [unwired: 11 in, 7 out]
          }
          frame 4 {
            n768 = property on="Current Task time" class="Slide (strict)"("Scale.Maximum"=w1544) -> ()  [unwired: 2 in, 2 out]
            n769 = call "Elapsed Time80"("Time Target (s)"=w1544) -> ("Elapsed Time (s)"=w1543:dbl)  [unwired: 11 in, 7 out]
          }
          frame 0, Default {
            n770 = property on="Current Task time" class="Slide (strict)"("Scale.Maximum"=w1546) -> ()  [unwired: 2 in, 2 out]
            n771 = call "Elapsed Time81"("Time Target (s)"=w1546) -> ("Elapsed Time (s)"=w1545:dbl)  [unwired: 11 in, 7 out]
          }
        }
      }
      frame 13 {
        w1600 = 51.0  # Routine Time
        # "Calibration Routine 4"
        n772 = property on="Total Routine Time" class="Slide (strict)"("Scale.Maximum"=w1600) -> ()  [unwired: 2 in, 2 out]
        n773 = call "Elapsed Time82"("Time Target (s)"=w1600, "Auto Reset"=FALSE ("Timer Reset")) -> ("Get Start Time (s)"=w1598:dbl, "Elapsed Time (s)"=w1594:dbl, "Time has Elapsed"=w1601:bool)  [unwired: 10 in, 5 out]
        "Calib 4" <- w1601
        n774 = Seconds To Date/Time(time stamp (now)=w1598) -> (date time rec=w1599:T2)  [unwired: 1 in]
        n775 = Not(x=w1601) -> (.not. x?=w1604:bool)
        n776 = script code="t = [0,15,18,22.5,25.5,30,33,37.5,40.5,45,45.75,46.5,47.25,48,48.75,49.5,50.25,51];\n\nevent = [0,1,2,1,2,1,2,1,2,3,4,3,4,3,4,3,4,3,4,14];\n\nfor i = 2:length(t)\n    if ((x>=t(i-1)) &&  (x<t(i)))\n        y = event(i-1);\n        yNext = event(i);\n        dt = t(i) - t(i-1);\n        break;\n    end\nend"("x"=w1594) -> ("y"=w1595:dbl, "dt"=w1596:dbl, "yNext"=w1597:dbl)  [unwired: 1 in, 1 out]
        n777 = case shown="False" w1604 {
          tunnel: [w1643 w1655] -> w1603
          frame False {
            n778 = flat-sequence {
              tunnel: [w1651] -> w1643
              frame #0 {
                n779 = local write "Buffer"(FALSE ("Buffer")) -> ()
                n780 = local write "Play/Stop"(FALSE ("Play\nCalibration")) -> ()
              }
              frame #1 {
                n781 = local write "Output"(0 ("Output")) -> ()
                n782 = local write "Save"(TRUE ("Save")) -> ()
              }
              frame #2 {
                n783 = Wait (ms)(milliseconds to wait=u32 500) -> ()  [unwired: 1 out]
              }
              frame #3 {
                n784 = local write "Flush"(TRUE ("Flush")) -> ()
              }
              frame #4 {
                w1650 = u16 0 items=["No sound", "Demo deep breathing", "Demo fast shallow breathing", "Demo slow shallow breathing", "Demo breath hold", "Demo cough/ laugh", "Demo abdomen movement", "Calibration", "Routine 1", "Routine 3", "Routine 4/5/7", "Calm music"] ("Play sound")
                w1651 = T4."Default"
                n785 = local write "Flush"(FALSE ("Flush")) -> ()
                n786 = local write "Save"(FALSE ("Save")) -> ()
                n787 = local write "Protocol"(w1651) -> ()
                n788 = local write "Play sound"(w1650) -> ()
              }
            }
          }
          frame True {
            w1654 = u16 7 items=["No sound", "Demo deep breathing", "Demo fast shallow breathing", "Demo slow shallow breathing", "Demo breath hold", "Demo cough/ laugh", "Demo abdomen movement", "Calibration", "Routine 1", "Routine 3", "Routine 4/5/7", "Calm music"] ("Play sound")
            n789 = local write "Play sound"(w1654) -> ()
            n790 = flat-sequence {
              tunnel: [T4."Calib4"] -> w1655
              frame #0 {
                n791 = local write "Output"(1 ("Open")) -> ()
                n792 = local write "Play/Stop"(TRUE ("Play\nCalibration")) -> ()
              }
              frame #1 {
                n793 = local write "Buffer"(TRUE ("Buffer")) -> ()
              }
              frame #2 {
              }
            }
          }
        }
        n794 = case shown="0, Default" w1595 {
          tunnel: ["\nPerform normal breathing, NO deep breathing or breath hold." "Inhale a slow deep breath." "\nExhale slowly." "Quick inhale.\n\n\n\nIf you cannot sustain for long, resume normal breathing." "\nQuick exhale.\n\n\nIf you cannot sustain for long, resume normal breathing." "Slow shallow inhale.\n\n\n\nIf you cannot sustain for long, resume normal breathing." "\nSlow exhale.\n\n\nIf you cannot sustain for long, resume normal breathing." "Exhale the current breath  and HOLD.\n\n\nIf you cannot sustain for long, resume normal breathing." "Perform voluntary coughing \n" "Perform voluntary laugh\n\n" "Read aloud the following text in between the lines:\n-----------------------------------------------------------------------\nFour score and seven years ago our fathers brought forth on this continent, a new nation, conceived in Liberty, and dedicated to the proposition that all men are created equal… That this nation, under God, shall have a new birth of freedom-and that government of the people, by the people, for the people, shall not perish from the earth.\n\n-----------------------------------------------------------------------\nWhen finished, take a deep breath and open mouth say \"Ah\" (like doctor checking your throat).\nPerform normal breathing until next instruction." "Exhale current breath and HOLD. Push abdomen inwards." "Relax abdomen back to normal and keep holding breath."] -> w1593
          frame 0, Default {
          }
          frame 1 {
          }
          frame 2 {
          }
          frame 3 {
          }
          frame 4 {
          }
          frame 5 {
          }
          frame 6 {
          }
          frame 7 {
          }
          frame 8 {
          }
          frame 9 {
          }
          frame 10 {
          }
          frame 12 {
          }
          frame 13 {
          }
        }
        n795 = case shown="0, Default" w1597 {
          tunnel: ["\nPerform normal breathing, NO deep breathing or breath hold." "Inhale a slow deep breath." "\nExhale slowly." "Quick inhale.\n\n\n\nIf you cannot sustain for long, resume normal breathing." "\nQuick exhale.\n\n\nIf you cannot sustain for long, resume normal breathing." "Slow shallow inhale.\n\n\n\nIf you cannot sustain for long, resume normal breathing." "\nSlow exhale.\n\n\nIf you cannot sustain for long, resume normal breathing." "Exhale the current breath  and HOLD.\n\n\nIf you cannot sustain for long, resume normal breathing." "Perform voluntary coughing \n" "Perform voluntary laugh\n\n" "Read aloud the following text in between the lines:\n-----------------------------------------------------------------------\nFour score and ...\n-----------------------------------------------------------------------\nWhen finished, take a deep breath and open mouth say \"Ah\" (like doctor checking your throat).\nPerform normal breathing until next instruction." "Exhale current breath and HOLD. Push abdomen inwards." "Relax abdomen back to normal and keep holding breath." "Study completed!"] -> w1591
          frame 0, Default {
          }
          frame 1 {
          }
          frame 2 {
          }
          frame 3 {
          }
          frame 4 {
          }
          frame 5 {
          }
          frame 6 {
          }
          frame 7 {
          }
          frame 8 {
          }
          frame 9 {
          }
          frame 10 {
          }
          frame 12 {
          }
          frame 13 {
          }
          frame 14 {
          }
        }
        n796 = case shown="0, Default" w1595 {
          tunnel: w1596 -> [w1607 w1609 w1611 w1613 w1615]
          tunnel: [w1606 w1608 w1610 w1612 w1614] -> w1592
          frame 1 {
            n797 = property on="Current Task time" class="Slide (strict)"("Scale.Maximum"=w1607) -> ()  [unwired: 2 in, 2 out]
            n798 = call "Elapsed Time83"("Time Target (s)"=w1607) -> ("Elapsed Time (s)"=w1606:dbl)  [unwired: 11 in, 7 out]
          }
          frame 2 {
            n799 = property on="Current Task time" class="Slide (strict)"("Scale.Maximum"=w1609) -> ()  [unwired: 2 in, 2 out]
            n800 = call "Elapsed Time84"("Time Target (s)"=w1609) -> ("Elapsed Time (s)"=w1608:dbl)  [unwired: 11 in, 7 out]
          }
          frame 3 {
            n801 = property on="Current Task time" class="Slide (strict)"("Scale.Maximum"=w1611) -> ()  [unwired: 2 in, 2 out]
            n802 = call "Elapsed Time85"("Time Target (s)"=w1611) -> ("Elapsed Time (s)"=w1610:dbl)  [unwired: 11 in, 7 out]
          }
          frame 4 {
            n803 = property on="Current Task time" class="Slide (strict)"("Scale.Maximum"=w1613) -> ()  [unwired: 2 in, 2 out]
            n804 = call "Elapsed Time86"("Time Target (s)"=w1613) -> ("Elapsed Time (s)"=w1612:dbl)  [unwired: 11 in, 7 out]
          }
          frame 0, Default {
            n805 = property on="Current Task time" class="Slide (strict)"("Scale.Maximum"=w1615) -> ()  [unwired: 2 in, 2 out]
            n806 = call "Elapsed Time87"("Time Target (s)"=w1615) -> ("Elapsed Time (s)"=w1614:dbl)  [unwired: 11 in, 7 out]
          }
        }
      }
      frame 14 {
        w1669 = 51.0  # Routine Time
        # "Calibration Routine 5"
        n807 = property on="Total Routine Time" class="Slide (strict)"("Scale.Maximum"=w1669) -> ()  [unwired: 2 in, 2 out]
        n808 = call "Elapsed Time88"("Time Target (s)"=w1669, "Auto Reset"=FALSE ("Timer Reset")) -> ("Get Start Time (s)"=w1667:dbl, "Elapsed Time (s)"=w1663:dbl, "Time has Elapsed"=w1670:bool)  [unwired: 10 in, 5 out]
        "Calib 5" <- w1670
        n809 = Seconds To Date/Time(time stamp (now)=w1667) -> (date time rec=w1668:T2)  [unwired: 1 in]
        n810 = Not(x=w1670) -> (.not. x?=w1673:bool)
        n811 = script code="t = [0,15,18,22.5,25.5,30,33,37.5,40.5,45,45.75,46.5,47.25,48,48.75,49.5,50.25,51];\n\nevent = [0,1,2,1,2,1,2,1,2,3,4,3,4,3,4,3,4,3,4,14];\n\nfor i = 2:length(t)\n    if ((x>=t(i-1)) &&  (x<t(i)))\n        y = event(i-1);\n        yNext = event(i);\n        dt = t(i) - t(i-1);\n        break;\n    end\nend"("x"=w1663) -> ("y"=w1664:dbl, "dt"=w1665:dbl, "yNext"=w1666:dbl)  [unwired: 1 in, 1 out]
        n812 = case shown="True" w1673 {
          tunnel: [w1712 w1724] -> w1672
          frame False {
            n813 = flat-sequence {
              tunnel: [w1720] -> w1712
              frame #0 {
                n814 = local write "Buffer"(FALSE ("Buffer")) -> ()
                n815 = local write "Play/Stop"(FALSE ("Play\nCalibration")) -> ()
              }
              frame #1 {
                n816 = local write "Output"(0 ("Output")) -> ()
                n817 = local write "Save"(TRUE ("Save")) -> ()
              }
              frame #2 {
                n818 = Wait (ms)(milliseconds to wait=u32 500) -> ()  [unwired: 1 out]
              }
              frame #3 {
                n819 = local write "Flush"(TRUE ("Flush")) -> ()
              }
              frame #4 {
                w1719 = u16 0 items=["No sound", "Demo deep breathing", "Demo fast shallow breathing", "Demo slow shallow breathing", "Demo breath hold", "Demo cough/ laugh", "Demo abdomen movement", "Calibration", "Routine 1", "Routine 3", "Routine 4/5/7", "Calm music"] ("Play sound")
                w1720 = T4."Default"
                n820 = local write "Flush"(FALSE ("Flush")) -> ()
                n821 = local write "Save"(FALSE ("Save")) -> ()
                n822 = local write "Protocol"(w1720) -> ()
                n823 = local write "Play sound"(w1719) -> ()
              }
            }
          }
          frame True {
            w1723 = u16 7 items=["No sound", "Demo deep breathing", "Demo fast shallow breathing", "Demo slow shallow breathing", "Demo breath hold", "Demo cough/ laugh", "Demo abdomen movement", "Calibration", "Routine 1", "Routine 3", "Routine 4/5/7", "Calm music"] ("Play sound")
            n824 = local write "Play sound"(w1723) -> ()
            n825 = flat-sequence {
              tunnel: [T4."Calib5"] -> w1724
              frame #0 {
                n826 = local write "Output"(1 ("Open")) -> ()
                n827 = local write "Play/Stop"(TRUE ("Play\nCalibration")) -> ()
              }
              frame #1 {
                n828 = local write "Buffer"(TRUE ("Buffer")) -> ()
              }
              frame #2 {
              }
            }
          }
        }
        n829 = case shown="0, Default" w1664 {
          tunnel: ["\nPerform normal breathing, NO deep breathing or breath hold." "Inhale a slow deep breath." "\nExhale slowly." "Quick inhale.\n\n\n\nIf you cannot sustain for long, resume normal breathing." "\nQuick exhale.\n\n\nIf you cannot sustain for long, resume normal breathing." "Slow shallow inhale.\n\n\n\nIf you cannot sustain for long, resume normal breathing." "\nSlow exhale.\n\n\nIf you cannot sustain for long, resume normal breathing." "Exhale the current breath  and HOLD.\n\n\nIf you cannot sustain for long, resume normal breathing." "Perform voluntary coughing \n" "Perform voluntary laugh\n\n" "Read aloud the following text in between the lines:\n-----------------------------------------------------------------------\nFour score and seven years ago our fathers brought forth on this continent, a new nation, conceived in Liberty, and dedicated to the proposition that all men are created equal… That this nation, under God, shall have a new birth of freedom-and that government of the people, by the people, for the people, shall not perish from the earth.\n\n-----------------------------------------------------------------------\nWhen finished, take a deep breath and open mouth say \"Ah\" (like doctor checking your throat).\nPerform normal breathing until next instruction." "Exhale current breath and HOLD. Push abdomen inwards." "Relax abdomen back to normal and keep holding breath."] -> w1662
          frame 0, Default {
          }
          frame 1 {
          }
          frame 2 {
          }
          frame 3 {
          }
          frame 4 {
          }
          frame 5 {
          }
          frame 6 {
          }
          frame 7 {
          }
          frame 8 {
          }
          frame 9 {
          }
          frame 10 {
          }
          frame 12 {
          }
          frame 13 {
          }
        }
        n830 = case shown="0, Default" w1666 {
          tunnel: ["\nPerform normal breathing, NO deep breathing or breath hold." "Inhale a slow deep breath." "\nExhale slowly." "Quick inhale.\n\n\n\nIf you cannot sustain for long, resume normal breathing." "\nQuick exhale.\n\n\nIf you cannot sustain for long, resume normal breathing." "Slow shallow inhale.\n\n\n\nIf you cannot sustain for long, resume normal breathing." "\nSlow exhale.\n\n\nIf you cannot sustain for long, resume normal breathing." "Exhale the current breath  and HOLD.\n\n\nIf you cannot sustain for long, resume normal breathing." "Perform voluntary coughing \n" "Perform voluntary laugh\n\n" "Read aloud the following text in between the lines:\n-----------------------------------------------------------------------\nFour score and ...\n-----------------------------------------------------------------------\nWhen finished, take a deep breath and open mouth say \"Ah\" (like doctor checking your throat).\nPerform normal breathing until next instruction." "Exhale current breath and HOLD. Push abdomen inwards." "Relax abdomen back to normal and keep holding breath." "Study completed!"] -> w1660
          frame 0, Default {
          }
          frame 1 {
          }
          frame 2 {
          }
          frame 3 {
          }
          frame 4 {
          }
          frame 5 {
          }
          frame 6 {
          }
          frame 7 {
          }
          frame 8 {
          }
          frame 9 {
          }
          frame 10 {
          }
          frame 12 {
          }
          frame 13 {
          }
          frame 14 {
          }
        }
        n831 = case shown="0, Default" w1664 {
          tunnel: w1665 -> [w1676 w1678 w1680 w1682 w1684]
          tunnel: [w1675 w1677 w1679 w1681 w1683] -> w1661
          frame 1 {
            n832 = property on="Current Task time" class="Slide (strict)"("Scale.Maximum"=w1676) -> ()  [unwired: 2 in, 2 out]
            n833 = call "Elapsed Time89"("Time Target (s)"=w1676) -> ("Elapsed Time (s)"=w1675:dbl)  [unwired: 11 in, 7 out]
          }
          frame 2 {
            n834 = property on="Current Task time" class="Slide (strict)"("Scale.Maximum"=w1678) -> ()  [unwired: 2 in, 2 out]
            n835 = call "Elapsed Time90"("Time Target (s)"=w1678) -> ("Elapsed Time (s)"=w1677:dbl)  [unwired: 11 in, 7 out]
          }
          frame 3 {
            n836 = property on="Current Task time" class="Slide (strict)"("Scale.Maximum"=w1680) -> ()  [unwired: 2 in, 2 out]
            n837 = call "Elapsed Time91"("Time Target (s)"=w1680) -> ("Elapsed Time (s)"=w1679:dbl)  [unwired: 11 in, 7 out]
          }
          frame 4 {
            n838 = property on="Current Task time" class="Slide (strict)"("Scale.Maximum"=w1682) -> ()  [unwired: 2 in, 2 out]
            n839 = call "Elapsed Time92"("Time Target (s)"=w1682) -> ("Elapsed Time (s)"=w1681:dbl)  [unwired: 11 in, 7 out]
          }
          frame 0, Default {
            n840 = property on="Current Task time" class="Slide (strict)"("Scale.Maximum"=w1684) -> ()  [unwired: 2 in, 2 out]
            n841 = call "Elapsed Time93"("Time Target (s)"=w1684) -> ("Elapsed Time (s)"=w1683:dbl)  [unwired: 11 in, 7 out]
          }
        }
      }
      frame 15 {
        w1738 = 51.0  # Routine Time
        # "Calibration Routine 7"
        n842 = property on="Total Routine Time" class="Slide (strict)"("Scale.Maximum"=w1738) -> ()  [unwired: 2 in, 2 out]
        n843 = call "Elapsed Time94"("Time Target (s)"=w1738, "Auto Reset"=FALSE ("Timer Reset")) -> ("Get Start Time (s)"=w1736:dbl, "Elapsed Time (s)"=w1732:dbl, "Time has Elapsed"=w1739:bool)  [unwired: 10 in, 5 out]
        "Calib 7" <- w1739
        n844 = Seconds To Date/Time(time stamp (now)=w1736) -> (date time rec=w1737:T2)  [unwired: 1 in]
        n845 = Not(x=w1739) -> (.not. x?=w1742:bool)
        n846 = script code="t = [0,15,18,22.5,25.5,30,33,37.5,40.5,45,45.75,46.5,47.25,48,48.75,49.5,50.25,51];\n\nevent = [0,1,2,1,2,1,2,1,2,3,4,3,4,3,4,3,4,3,4,14];\n\nfor i = 2:length(t)\n    if ((x>=t(i-1)) &&  (x<t(i)))\n        y = event(i-1);\n        yNext = event(i);\n        dt = t(i) - t(i-1);\n        break;\n    end\nend"("x"=w1732) -> ("y"=w1733:dbl, "dt"=w1734:dbl, "yNext"=w1735:dbl)  [unwired: 1 in, 1 out]
        n847 = case shown="False" w1742 {
          tunnel: [w1781 w1793] -> w1741
          frame False {
            n848 = flat-sequence {
              tunnel: [w1789] -> w1781
              frame #0 {
                n849 = local write "Buffer"(FALSE ("Buffer")) -> ()
                n850 = local write "Play/Stop"(FALSE ("Play\nCalibration")) -> ()
              }
              frame #1 {
                n851 = local write "Output"(0 ("Output")) -> ()
                n852 = local write "Save"(TRUE ("Save")) -> ()
              }
              frame #2 {
                n853 = Wait (ms)(milliseconds to wait=u32 500) -> ()  [unwired: 1 out]
              }
              frame #3 {
                n854 = local write "Flush"(TRUE ("Flush")) -> ()
              }
              frame #4 {
                w1788 = u16 0 items=["No sound", "Demo deep breathing", "Demo fast shallow breathing", "Demo slow shallow breathing", "Demo breath hold", "Demo cough/ laugh", "Demo abdomen movement", "Calibration", "Routine 1", "Routine 3", "Routine 4/5/7", "Calm music"] ("Play sound")
                w1789 = T4."Default"
                n855 = local write "Flush"(FALSE ("Flush")) -> ()
                n856 = local write "Save"(FALSE ("Save")) -> ()
                n857 = local write "Play sound"(w1788) -> ()
                n858 = local write "Protocol"(w1789) -> ()
              }
            }
          }
          frame True {
            w1792 = u16 7 items=["No sound", "Demo deep breathing", "Demo fast shallow breathing", "Demo slow shallow breathing", "Demo breath hold", "Demo cough/ laugh", "Demo abdomen movement", "Calibration", "Routine 1", "Routine 3", "Routine 4/5/7", "Calm music"] ("Play sound")
            n859 = local write "Play sound"(w1792) -> ()
            n860 = flat-sequence {
              tunnel: [T4."Calib7"] -> w1793
              frame #0 {
                n861 = local write "Output"(1 ("Open")) -> ()
                n862 = local write "Play/Stop"(TRUE ("Play\nCalibration")) -> ()
              }
              frame #1 {
                n863 = local write "Buffer"(TRUE ("Buffer")) -> ()
              }
              frame #2 {
              }
            }
          }
        }
        n864 = case shown="0, Default" w1733 {
          tunnel: ["\nPerform normal breathing, NO deep breathing or breath hold." "Inhale a slow deep breath." "\nExhale slowly." "Quick inhale.\n\n\n\nIf you cannot sustain for long, resume normal breathing." "\nQuick exhale.\n\n\nIf you cannot sustain for long, resume normal breathing." "Slow shallow inhale.\n\n\n\nIf you cannot sustain for long, resume normal breathing." "\nSlow exhale.\n\n\nIf you cannot sustain for long, resume normal breathing." "Exhale the current breath  and HOLD.\n\n\nIf you cannot sustain for long, resume normal breathing." "Perform voluntary coughing \n" "Perform voluntary laugh\n\n" "Read aloud the following text in between the lines:\n-----------------------------------------------------------------------\nFour score and seven years ago our fathers brought forth on this continent, a new nation, conceived in Liberty, and dedicated to the proposition that all men are created equal… That this nation, under God, shall have a new birth of freedom-and that government of the people, by the people, for the people, shall not perish from the earth.\n\n-----------------------------------------------------------------------\nWhen finished, take a deep breath and open mouth say \"Ah\" (like doctor checking your throat).\nPerform normal breathing until next instruction." "Exhale current breath and HOLD. Push abdomen inwards." "Relax abdomen back to normal and keep holding breath."] -> w1731
          frame 0, Default {
          }
          frame 1 {
          }
          frame 2 {
          }
          frame 3 {
          }
          frame 4 {
          }
          frame 5 {
          }
          frame 6 {
          }
          frame 7 {
          }
          frame 8 {
          }
          frame 9 {
          }
          frame 10 {
          }
          frame 12 {
          }
          frame 13 {
          }
        }
        n865 = case shown="0, Default" w1735 {
          tunnel: ["\nPerform normal breathing, NO deep breathing or breath hold." "Inhale a slow deep breath." "\nExhale slowly." "Quick inhale.\n\n\n\nIf you cannot sustain for long, resume normal breathing." "\nQuick exhale.\n\n\nIf you cannot sustain for long, resume normal breathing." "Slow shallow inhale.\n\n\n\nIf you cannot sustain for long, resume normal breathing." "\nSlow exhale.\n\n\nIf you cannot sustain for long, resume normal breathing." "Exhale the current breath  and HOLD.\n\n\nIf you cannot sustain for long, resume normal breathing." "Perform voluntary coughing \n" "Perform voluntary laugh\n\n" "Read aloud the following text in between the lines:\n-----------------------------------------------------------------------\nFour score and ...\n-----------------------------------------------------------------------\nWhen finished, take a deep breath and open mouth say \"Ah\" (like doctor checking your throat).\nPerform normal breathing until next instruction." "Exhale current breath and HOLD. Push abdomen inwards." "Relax abdomen back to normal and keep holding breath." "Study completed!"] -> w1729
          frame 0, Default {
          }
          frame 1 {
          }
          frame 2 {
          }
          frame 3 {
          }
          frame 4 {
          }
          frame 5 {
          }
          frame 6 {
          }
          frame 7 {
          }
          frame 8 {
          }
          frame 9 {
          }
          frame 10 {
          }
          frame 12 {
          }
          frame 13 {
          }
          frame 14 {
          }
        }
        n866 = case shown="0, Default" w1733 {
          tunnel: w1734 -> [w1745 w1747 w1749 w1751 w1753]
          tunnel: [w1744 w1746 w1748 w1750 w1752] -> w1730
          frame 1 {
            n867 = property on="Current Task time" class="Slide (strict)"("Scale.Maximum"=w1745) -> ()  [unwired: 2 in, 2 out]
            n868 = call "Elapsed Time95"("Time Target (s)"=w1745) -> ("Elapsed Time (s)"=w1744:dbl)  [unwired: 11 in, 7 out]
          }
          frame 2 {
            n869 = property on="Current Task time" class="Slide (strict)"("Scale.Maximum"=w1747) -> ()  [unwired: 2 in, 2 out]
            n870 = call "Elapsed Time96"("Time Target (s)"=w1747) -> ("Elapsed Time (s)"=w1746:dbl)  [unwired: 11 in, 7 out]
          }
          frame 3 {
            n871 = property on="Current Task time" class="Slide (strict)"("Scale.Maximum"=w1749) -> ()  [unwired: 2 in, 2 out]
            n872 = call "Elapsed Time97"("Time Target (s)"=w1749) -> ("Elapsed Time (s)"=w1748:dbl)  [unwired: 11 in, 7 out]
          }
          frame 4 {
            n873 = property on="Current Task time" class="Slide (strict)"("Scale.Maximum"=w1751) -> ()  [unwired: 2 in, 2 out]
            n874 = call "Elapsed Time98"("Time Target (s)"=w1751) -> ("Elapsed Time (s)"=w1750:dbl)  [unwired: 11 in, 7 out]
          }
          frame 0, Default {
            n875 = property on="Current Task time" class="Slide (strict)"("Scale.Maximum"=w1753) -> ()  [unwired: 2 in, 2 out]
            n876 = call "Elapsed Time99"("Time Target (s)"=w1753) -> ("Elapsed Time (s)"=w1752:dbl)  [unwired: 11 in, 7 out]
          }
        }
      }
    }
    "Numeric 2" <- w882
    "Elapsed Time (s)" <- w880
    "Current Task" <- w881
    "Total Routine Time" <- w880
    "date time rec" <- w879
    "Current Task time" <- w878
    "Next Task" <- w876
    n877 = Wait (ms)(milliseconds to wait=u32 2 ("millisecond timer value")) -> ()  [unwired: 1 out]
    n878 = property on="Current Task time" class="Slide (strict)"("Scale.Minimum"=0.0 ("Scale.Range:Minimum")) -> ()  [unwired: 2 in, 2 out]
  }
  n879 = call <vilib>:"Sound Input Configure.vi"("number of samples/ch"="Number of Samples/ch", "sample mode"=w8, "sound format"=T5 {"sample rate (S/s)"=50000.0, "number of channels"=1, "bits per sample"=16} ("Sound Format"), "device ID"="Device ID") -> ("error out"=w13:errorcluster, "task ID"=w11:T11)  [unwired: 6 in]
  n880 = while {
    tunnel: w11 -> [w1810]
    tunnel: [w1809] -> w10
    tunnel: "Number of Samples/ch" -> [w1808]
    tunnel: w13 -> [w1811]
    tunnel: [w1805] -> w9
    tunnel: w2 -> [w1801]
    stop <- w1806 stop-if-true
    # "Read Sound Data"
    n881 = call-poly <vilib>:"Sound Input Read.vi"("number of samples/ch"=w1808, "error in (no error)"=w1811, "task ID"=w1810) -> ("error out"=w1805:errorcluster, "data"=w1798:waveform(dbl)[], "task ID out"=w1809:T11)  [unwired: 6 in]
    "Mic" <- w1798
    n882 = Get Queue Status(queue=w1801) -> (# elements in queue=→"# elements in Mic":i32)  [unwired: 2 in, 7 out]
    n883 = Or(x=w1805, y="Stop 3") -> (x .or. y?=w1806:bool)
    n884 = Index Array(array=w1798, index=0) -> (element=w1803:waveform(dbl))
    n885 = Unbundle By Name(w1803) -> ("Y"=w1802:dbl[])
    n886 = case shown="False" "FlushMic" {
      tunnel: w1802 -> [_ w1814]
      tunnel: w1801 -> [w1812 w1813]
      frame True {
        n887 = Flush Queue(queue=w1812) -> ()  [unwired: 1 in, 3 out]
      }
      frame False {
        n888 = for {
          tunnel: w1813 -> [w1816]
          tunnel: w1814 -> [w1815] mode=indexing
          n889 = Enqueue Element(queue=w1816, element=w1815) -> ()  [unwired: 2 in, 3 out]
        }
      }
    }
  }
  n890 = call <vilib>:"Sound Input Clear.vi"("error in (no error)"=w9, "task ID"=w10) -> ("error out"=w6:errorcluster)  [unwired: 9 in]
  n891 = call <vilib>:"Simple Error Handler.vi"("error in (no error)"=w6) -> ()  [unwired: 4 in, 5 out]
  n892 = local read "DownSamplingRatio"() -> (w43:i32)
  n893 = local read "Waveform Size 1"() -> (w44:dbl)
  n894 = Divide(x=w44, y=w43) -> (x/y=w31:dbl)
  n895 = Divide(x=w31, y="DownSamplingRatio 2") -> (x/y=w15:dbl)
  n896 = Multiply(x=w17, y=w15) -> (x*y=w38:dbl)
  n897 = Initialize Array(w16, w17, w15) -> (w42:dbl[][])
  n898 = Initialize Array(w16, w17, w15) -> (w41:dbl[][])
  n899 = Initialize Array(w16, w17, w15) -> (w40:dbl[][])
  n900 = Initialize Array(w16, w17, w15) -> (w39:dbl[][])
  n901 = while {
    tunnel: w17 -> [w1888]
    tunnel: w45 -> [w1881]
    shift-right: [w1878] -> _
    shift-left: w42 -> [w1847]
    tunnel: w38 -> [w1824]
    shift-right: [w1869] -> _
    shift-left: w41 -> [w1884]
    shift-right: [w1868] -> _
    shift-left: w40 -> [w1883]
    shift-right: [w1867] -> _
    shift-left: w39 -> [w1882]
    tunnel: "DownSamplingRatio 2" -> [w1821]
    tunnel: w15 -> [w1825]
    tunnel: "DownSamplingRatio 2" -> [w1827]
    stop <- FALSE stop-if-true
    n902 = local read "Sampling Rate"() -> (w1828:dbl)
    n903 = Get Queue Status(queue=w1881) -> (# elements in queue=→"# elements in queue":i32)  [unwired: 2 in, 7 out]
    n904 = Dequeue Element(queue=w1881) -> (element=w1826:dbl[][])  [unwired: 2 in, 3 out]
    n905 = Decrement(x=w1888) -> (x-1=w1822:i32)
    n906 = Divide(x=w1828, y=w1827) -> (x/y=→"Dis Sampling Rate":dbl)
    n907 = Index Array(array=w1826, index (row)=0 ("index")) -> (element=w1845:dbl[])  [unwired: 1 in]
    n908 = Index Array(array=w1826, index (row)=1 ("index")) -> (element=w1844:dbl[])  [unwired: 1 in]
    n909 = Index Array(array=w1826, index (row)=2 ("index")) -> (element=w1843:dbl[])  [unwired: 1 in]
    n910 = Index Array(array=w1826, index (row)=3 ("index")) -> (element=w1842:dbl[])  [unwired: 1 in]
    n911 = Reshape Array(w1844, w1825, w1821) -> (w1838:dbl[][])
    n912 = Reshape Array(w1843, w1825, w1821) -> (w1837:dbl[][])
    n913 = Reshape Array(w1842, w1825, w1821) -> (w1836:dbl[][])
    n914 = Reshape Array(w1845, w1825, w1821) -> (w1841:dbl[][])
    n915 = for {
      tunnel: w1837 -> [w1898] mode=indexing
      tunnel: [w1897] -> w1834 mode=indexing
      n916 = Add Array Elements(numeric array=w1898) -> (sum=w1897:dbl)
    }
    n917 = for {
      tunnel: w1836 -> [w1896] mode=indexing
      tunnel: [w1895] -> w1833 mode=indexing
      n918 = Add Array Elements(numeric array=w1896) -> (sum=w1895:dbl)
    }
    n919 = for {
      tunnel: w1838 -> [w1900] mode=indexing
      tunnel: [w1899] -> w1835 mode=indexing
      n920 = Add Array Elements(numeric array=w1900) -> (sum=w1899:dbl)
    }
    n921 = for {
      tunnel: w1841 -> [w1902] mode=indexing
      tunnel: [w1901] -> w1840 mode=indexing
      n922 = Add Array Elements(numeric array=w1902) -> (sum=w1901:dbl)
    }
    n923 = Array Subset(array=w1883, index (row)=0 ("index"), length (row)=w1822) -> (w1871:dbl[][])  [unwired: 2 in]
    n924 = Array Subset(array=w1882, index (row)=0 ("index"), length (row)=w1822) -> (w1870:dbl[][])  [unwired: 2 in]
    n925 = Array Subset(array=w1884, index (row)=0 ("index"), length (row)=w1822) -> (w1872:dbl[][])  [unwired: 2 in]
    n926 = Array Subset(array=w1847, index (row)=0 ("index"), length (row)=w1822) -> (w1879:dbl[][])  [unwired: 2 in]
    n927 = Divide(x=w1840, y=w1821) -> (x/y=w1839:dbl[])
    n928 = Divide(x=w1835, y=w1821) -> (x/y=w1830:dbl[])
    n929 = Divide(x=w1834, y=w1821) -> (x/y=w1831:dbl[])
    n930 = Divide(x=w1833, y=w1821) -> (x/y=w1832:dbl[])
    n931 = Build Array (concatenate)(w1832, w1870) -> (w1867:dbl[][])
    n932 = Build Array (concatenate)(w1831, w1871) -> (w1868:dbl[][])
    n933 = Build Array (concatenate)(w1830, w1872) -> (w1869:dbl[][])
    n934 = local read "Dis Sampling Rate"() -> (w1823:dbl)
    n935 = Build Array (concatenate)(w1839, w1879) -> (w1878:dbl[][])
    n936 = Reshape Array(w1867, w1824) -> (w1849:dbl[])
    n937 = Reshape Array(w1868, w1824) -> (w1848:dbl[])
    n938 = Reshape Array(w1869, w1824) -> (w1850:dbl[])
    n939 = Reshape Array(w1878, w1824) -> (w1851:dbl[])
    n940 = call-poly <vilib>:"Butterworth Filter.vi"("init/cont (init:F)"=TRUE, "order"=3, "filter type"=Filter_Passband_Type."Bandpass", "low cutoff freq: fl"="fl 3", "high cutoff freq: fh"="fh 3", "sampling freq: fs"=w1823, "X"=w1848) -> ("Filtered X"=w1852:dbl[])  [unwired: 1 in, 1 out]
    n941 = call-poly <vilib>:"Butterworth Filter.vi"("init/cont (init:F)"=TRUE, "order"=3, "filter type"=Filter_Passband_Type."Lowpass", "low cutoff freq: fl"="fl 4", "high cutoff freq: fh"="fh 4", "sampling freq: fs"=w1823, "X"=w1849) -> ("Filtered X"=w1853:dbl[])  [unwired: 1 in, 1 out]
    n942 = call-poly <vilib>:"Butterworth Filter.vi"("init/cont (init:F)"=TRUE, "order"=3, "filter type"=Filter_Passband_Type."Lowpass", "low cutoff freq: fl"="fl 2", "high cutoff freq: fh"="fh 2", "sampling freq: fs"=w1823, "X"=w1850) -> ("Filtered X"=w1854:dbl[])  [unwired: 1 in, 1 out]
    n943 = call-poly <vilib>:"Butterworth Filter.vi"("init/cont (init:F)"=TRUE, "order"=3, "filter type"=Filter_Passband_Type."Bandpass", "low cutoff freq: fl"="fl 1", "high cutoff freq: fh"="fh 1", "sampling freq: fs"=w1823, "X"=w1851) -> ("Filtered X"=w1855:dbl[])  [unwired: 1 in, 1 out]
    n944 = Build Array(w1855, w1854, w1852, w1853) -> (→"2Ch Waveforms":dbl[][])
  }
  n945 = while {
    tunnel: w34 -> [w1906]
    tunnel: w27 -> [w1905]
    stop <- FALSE stop-if-true
    n946 = Get Queue Status(queue=w1906) -> (queue out=w1908:refnum<queue>, # elements in queue=w1909:i32)  [unwired: 2 in, 6 out]
    "# elements in queue 2" <- w1909
    n947 = local read "Save"() -> (w1903:bool)
    n948 = Wait (ms)(milliseconds to wait=u32 20) -> ()  [unwired: 1 out]
    n949 = case shown="False" w1903 {
      tunnel: w1909 -> [_ w1951]
      tunnel: w1908 -> [_ w1953]
      tunnel: w1905 -> [_ w1950]
      frame False {
      }
      frame True {
        # "Top 2 are amplitude"
        n950 = Multiply(x=w1951, y=w1950) -> (x*y=w1913:dbl)
        n951 = local read "date time rec"() -> (w1940:T2)
        n952 = for {
          N: w1951 -> [_]
          tunnel: [w2053] -> w1952 mode=indexing
          tunnel: [w2049] -> w1949 mode=indexing
          tunnel: [w2048] -> w1948 mode=indexing
          tunnel: [w2047] -> w1947 mode=indexing
          shift-right: [w2045] -> _
          shift-left: w1953 -> [w2055]
          tunnel: [w2042] -> w1914 mode=indexing
          i -> [w2046]
          # "Microphone"
          n953 = Dequeue Element(queue=w2055) -> (queue out=w2045:refnum<queue>, element=w2043:dbl[][])  [unwired: 2 in, 2 out]
          n954 = Index Array(array=w2043, index (row)=2) -> (element=w2048:dbl[])  [unwired: 1 in]
          n955 = Index Array(array=w2043, index (row)=1) -> (element=w2049:dbl[])  [unwired: 1 in]
          n956 = Index Array(array=w2043, index (row)=3) -> (element=w2047:dbl[])  [unwired: 1 in]
          n957 = Index Array(array=w2043, index (row)=0) -> (element=w2053:dbl[])  [unwired: 1 in]
          n958 = Index Array(array=w2043, index (row)=4) -> (element=w2042:dbl[])  [unwired: 1 in]
          "IterationNum" <- w2046
        }
        n959 = Unbundle By Name(w1940) -> ("fractional second"=w1933:dbl, "second"=w1934:i32, "minute"=w1935:i32, "hour"=w1936:i32, "day of month"=w1937:i32, "month"=w1938:i32, "year"=w1939:i32)
        n960 = property on="month" class="DigNum (strict)"() -> ("Label.Text"=w1929:string)  [unwired: 2 in, 2 out]
        n961 = property on="year" class="DigNum (strict)"() -> ("Label.Text"=w1930:string)  [unwired: 2 in, 2 out]
        n962 = property on="hour" class="DigNum (strict)"() -> ("Label.Text"=w1927:string)  [unwired: 2 in, 2 out]
        n963 = property on="day" class="DigNum (strict)"() -> ("Label.Text"=w1928:string)  [unwired: 2 in, 2 out]
        n964 = property on="fractionalSecond" class="DigNum (strict)"() -> ("Label.Text"=w1924:string)  [unwired: 2 in, 2 out]
        n965 = property on="second" class="DigNum (strict)"() -> ("Label.Text"=w1925:string)  [unwired: 2 in, 2 out]
        n966 = property on="minute" class="DigNum (strict)"() -> ("Label.Text"=w1926:string)  [unwired: 2 in, 2 out]
        n967 = Format Date/Time String(time format string (%c)="%m%d_%H%M%S") -> (date/time string=w1922:string)  [unwired: 2 in]
        n968 = property on="Protocol" class="Ring (strict)"() -> ("RingText.Text"=w1942:string)  [unwired: 2 in, 2 out]
        n969 = Concatenate Strings(w1922, w1942) -> (w1941:string)
        n970 = flat-sequence {
          tunnel: w1941 -> [w2027]
          tunnel: path "E:/NCS/HumanStudyMarch2019/Data" ("base path") -> [w2037]
          tunnel: w1916 -> [w1967]
          tunnel: w1915 -> [w1968]
          tunnel: "Case Number" -> [w2034]
          tunnel: "Sex" -> [w2030]
          tunnel: w1944 -> [w1966]
          tunnel: w1943 -> [w1965]
          tunnel: w1939 -> [w2017]
          tunnel: w1938 -> [w2012]
          tunnel: w1937 -> [w2007]
          tunnel: w1936 -> [w2006]
          tunnel: w1935 -> [w2005]
          tunnel: w1934 -> [w2000]
          tunnel: w1933 -> [w1999]
          tunnel: "Age (years)" -> [w1994]
          tunnel: "Height (cm)" -> [w1993]
          tunnel: "Weight (lbs)" -> [w1992]
          tunnel: w1930 -> [w1988]
          tunnel: w1929 -> [w1987]
          tunnel: w1928 -> [w1986]
          tunnel: w1927 -> [w1985]
          tunnel: w1926 -> [w1984]
          tunnel: w1925 -> [w1983]
          tunnel: w1924 -> [w1982]
          tunnel: "Comments" -> [w1975]
          tunnel: w1912 -> [w1969]
          tunnel: "Thorax Circumference (cm)" -> [w1957]
          tunnel: "Abd Circumference (cm)" -> [w1956]
          frame #0 {
            n971 = Build Path(base path=w2037, name or relative path=w2027) -> (appended path=w2040:path)
            n972 = TDMS Open(6:FALSE ("disable buffering (T)"), 10:T12."open or create" ("operation"), 11:w2040) -> (0:w2035:errorcluster, 3:w2036:refnum<k34>)  [unwired: 4 in]
            n973 = TDMS Set Properties(5:w2034, 7:"CaseNumber" ("property names"), 8:w2035, 11:w2036) -> (0:w2032:errorcluster, 3:w2031:refnum<k34>)  [unwired: 2 in, 2 out]
            n974 = TDMS Set Properties(5:w2030, 7:"Sex" ("property names"), 8:w2032, 11:w2031) -> (0:w1998:errorcluster, 3:w1997:refnum<k34>)  [unwired: 2 in, 2 out]
            n975 = TDMS Set Properties(5:w1994, 7:"Age_yr" ("property names"), 8:w1998, 11:w1997) -> (0:w1996:errorcluster, 3:w1995:refnum<k34>)  [unwired: 2 in, 2 out]
            n976 = TDMS Set Properties(5:w1993, 7:"Height_cm" ("property names"), 8:w1996, 11:w1995) -> (0:w1963:errorcluster, 3:w1962:refnum<k34>)  [unwired: 2 in, 2 out]
            n977 = TDMS Set Properties(5:w1956, 7:"Abd_cm" ("property names"), 8:w1963, 11:w1962) -> (0:w1961:errorcluster, 3:w1960:refnum<k34>)  [unwired: 2 in, 2 out]
            n978 = TDMS Set Properties(5:w1957, 7:"Th_cm" ("property names"), 8:w1961, 11:w1960) -> (0:w1958:errorcluster, 3:w1959:refnum<k34>)  [unwired: 2 in, 2 out]
            n979 = TDMS Set Properties(5:w1992, 7:"Weight_lbs" ("property names"), 8:w1958, 11:w1959) -> (0:w1979:errorcluster, 3:w1978:refnum<k34>)  [unwired: 2 in, 2 out]
            n980 = TDMS Set Properties(5:w1975, 7:"Comments" ("property names"), 8:w1979, 11:w1978) -> (0:w1976:errorcluster, 3:w1977:refnum<k34>)  [unwired: 2 in, 2 out]
            n981 = TDMS Set Properties(5:w2017, 7:w1988, 8:w1976, 11:w1977) -> (0:w2016:errorcluster, 3:w2015:refnum<k34>)  [unwired: 2 in, 2 out]
            n982 = TDMS Set Properties(5:w2012, 7:w1987, 8:w2016, 11:w2015) -> (0:w2014:errorcluster, 3:w2013:refnum<k34>)  [unwired: 2 in, 2 out]
            n983 = TDMS Set Properties(5:w2007, 7:w1986, 8:w2014, 11:w2013) -> (0:w2011:errorcluster, 3:w2010:refnum<k34>)  [unwired: 2 in, 2 out]
            n984 = TDMS Set Properties(5:w2006, 7:w1985, 8:w2011, 11:w2010) -> (0:w2009:errorcluster, 3:w2008:refnum<k34>)  [unwired: 2 in, 2 out]
            n985 = TDMS Set Properties(5:w2005, 7:w1984, 8:w2009, 11:w2008) -> (0:w2004:errorcluster, 3:w2003:refnum<k34>)  [unwired: 2 in, 2 out]
            n986 = TDMS Set Properties(5:w2000, 7:w1983, 8:w2004, 11:w2003) -> (0:w2001:errorcluster, 3:w2002:refnum<k34>)  [unwired: 2 in, 2 out]
            n987 = TDMS Set Properties(5:w1999, 7:w1982, 8:w2001, 11:w2002) -> (0:w1980:errorcluster, 3:w1981:refnum<k34>)  [unwired: 2 in, 2 out]
            n988 = TDMS Write(0:w1981, 7:"Tx1Rx1Amp" ("channel name(s) in (Untitled)"), 9:w1965, 11:w1980) -> (4:w2026:refnum<k34>, 15:w2025:errorcluster)  [unwired: 2 in, 2 out]
            n989 = TDMS Write(0:w2026, 7:"Tx2Rx2Amp" ("channel name(s) in (Untitled)"), 9:w1966, 11:w2025) -> (4:w2023:refnum<k34>, 15:w2022:errorcluster)  [unwired: 2 in, 2 out]
            n990 = TDMS Write(0:w2023, 7:"Tx1Rx1Ph" ("channel name(s) in (Untitled)"), 9:w1967, 11:w2022) -> (4:w2021:refnum<k34>, 15:w2020:errorcluster)  [unwired: 2 in, 2 out]
            n991 = TDMS Write(0:w2021, 7:"Tx2Rx2Ph" ("channel name(s) in (Untitled)"), 9:w1968, 11:w2020) -> (4:w1973:refnum<k34>, 15:w1970:errorcluster)  [unwired: 2 in, 2 out]
            n992 = TDMS Write(0:w1973, 7:"Mic" ("channel name(s) in (Untitled)"), 9:w1969, 11:w1970) -> (4:w1972:refnum<k34>, 15:w1971:errorcluster)  [unwired: 2 in, 2 out]
            n993 = TDMS Close(8:w1971, 11:w1972) -> ()  [unwired: 2 out]
          }
          frame #1 {
            n994 = local write "Save"(FALSE) -> ()
          }
        }
        n995 = Reshape Array(w1948, w1913) -> (w1916:dbl[])
        n996 = Reshape Array(w1947, w1913) -> (w1915:dbl[])
        n997 = Reshape Array(w1949, w1913) -> (w1944:dbl[])
        n998 = Reshape Array(w1952, w1913) -> (w1943:dbl[])
        n999 = Reshape Array(w1914, w1913) -> (w1912:dbl[])
        n1000 = Build Array(w1943, w1944) -> (→"IQ Graph 5":dbl[][])
        n1001 = Build Array(w1916, w1915) -> (→"IQ Graph 6":dbl[][])
      }
    }
  }
  n1002 = while {
    stop <- FALSE stop-if-true
    n1003 = local read "2Ch Waveforms"() -> (w2059:dbl[][])
    n1004 = Index Array(array=w2059, index (row)=0 ("index")) -> (element=→"Ch1Amp":dbl[])  [unwired: 1 in]
    n1005 = Index Array(array=w2059, index (row)=1 ("index")) -> (element=→"Ch2Amp":dbl[])  [unwired: 1 in]
    n1006 = Index Array(array=w2059, index (row)=2 ("index")) -> (element=→"Ch1Ph":dbl[])  [unwired: 1 in]
    n1007 = Index Array(array=w2059, index (row)=3 ("index")) -> (element=→"Ch2Ph":dbl[])  [unwired: 1 in]
    n1008 = Wait (ms)(milliseconds to wait=u32 20) -> ()  [unwired: 1 out]
  }
  "error out" <- w82
